vi "Straight.vi"() -> (4 "left":T2[](array[typedef])=[{"dt"=0.005, "x"=0.0, "y"=232.0, "position"=-3.125e-05, "velocity"=-0.0125, "acceleration"=-2.5, "jerk"=-500.0, "heading"=-0.0}, {"dt"=0.005, "x"=0.0, "y"=232.0, "position"=-3.125e-05, "velocity"=-0.0, "acceleration"=2.5, "jerk"=1000.0, "heading"=-0.0}, {"dt"=0.005, "x"=0.0, "y"=232.0, "position"=-3.125e-05, "velocity"=-0.0, "acceleration"=-0.0, "jerk"=-500.0, "heading"=-0.0}, {"dt"=0.005, "x"=0.0, "y"=232.0, "position"=-3.125e-05, "velocity"=-0.0, "acceleration"=-0.0, "jerk"=-0.0, "heading"=-0.0}, {"dt"=0.005, "x"=0.0, "y"=232.0, "position"=-3.125e-05, "velocity"=-0.0, "acceleration"=-0.0, "jerk"=-0.0, "heading"=-0.0}, {"dt"=0.005, "x"=0.0, "y"=232.0, "position"=-3.125e-05, "velocity"=-0.0, "acceleration"=-0.0, "jerk"=-0.0, "heading"=-0.0}, {"dt"=0.005, "x"=0.0, "y"=232.0, "position"=-3.125e-05, "velocity"=-0.0, "acceleration"=-0.0, "jerk"=-0.0, "heading"=-0.0}, {"dt"=0.005, "x"=0.0, "y"=232.0, "position"=-3.125e-05, "velocity"=-0.0, "acceleration"=-0.0, "jerk"=-0.0, "heading"=-0.0}, {"dt"=0.005, "x"=0.0, "y"=232.0, "position"=-3.125e-05, "velocity"=-0.0, "acceleration"=-0.0, "jerk"=-0.0, "heading"=-0.0}, {"dt"=0.005, "x"=3.124999999999981e-05, "y"=232.0, "position"=-6.249999999999981e-05, "velocity"=-0.006249999999999962, "acceleration"=-1.2499999999999925, "jerk"=-249.9999999999985, "heading"=-0.0}, {"dt"=0.005, "x"=0.003812499999999998, "y"=232.0, "position"=-0.0038437499999999978, "velocity"=-0.7562499999999996, "acceleration"=-149.99999999999994, "jerk"=-29749.99999999999, "heading"=-0.0}, {"dt"=0.005, "x"=0.008312499999999999, "y"=232.0, "position"=-0.008343749999999999, "velocity"=-0.9000000000000001, "acceleration"=-28.750000000000096, "jerk"=24249.999999999967, "heading"=-0.0}, {"dt"=0.005, "x"=0.013593749999999998, "y"=232.0, "position"=-0.013624999999999998, "velocity"=-1.05625, "acceleration"=-31.249999999999954, "jerk"=-499.9999999999716, "heading"=-0.0}, {"dt"=0.005, "x"=0.019718749999999997, "y"=232.0, "position"=-0.019749999999999997, "velocity"=-1.2249999999999996, "acceleration"=-33.74999999999994, "jerk"=-499.99999999999784, "heading"=-0.0}, {"dt"=0.005, "x"=0.026749999999999996, "y"=232.0, "position"=-0.026781249999999996, "velocity"=-1.4062499999999998, "acceleration"=-36.25000000000003, "jerk"=-500.00000000001705, "heading"=-0.0}, {"dt"=0.005, "x"=0.03474999999999999, "y"=232.0, "position"=-0.034781249999999986, "velocity"=-1.5999999999999985, "acceleration"=-38.74999999999975, "jerk"=-499.9999999999446, "heading"=-0.0}, {"dt"=0.005, "x"=0.04378125, "y"=232.0, "position"=-0.0438125, "velocity"=-1.8062500000000024, "acceleration"=-41.25000000000076, "jerk"=-500.0000000002018, "heading"=-0.0}, {"dt"=0.005, "x"=0.053906249999999996, "y"=232.0, "position"=-0.05393749999999999, "velocity"=-2.024999999999999, "acceleration"=-43.74999999999933, "jerk"=-499.99999999971436, "heading"=-0.0}, {"dt"=0.005, "x"=0.06518749999999998, "y"=232.0, "position"=-0.06521874999999998, "velocity"=-2.256249999999997, "acceleration"=-46.24999999999959, "jerk"=-500.00000000005116, "heading"=-0.0}, {"dt"=0.005, "x"=0.07768749999999996, "y"=232.0, "position"=-0.07771874999999996, "velocity"=-2.4999999999999964, "acceleration"=-48.74999999999989, "jerk"=-500.0000000000611, "heading"=-0.0}, {"dt"=0.005, "x"=0.09143749999999998, "y"=232.0, "position"=-0.09146874999999997, "velocity"=-2.750000000000002, "acceleration"=-50.00000000000115, "jerk"=-250.00000000025153, "heading"=-0.0}, {"dt"=0.005, "x"=0.10643749999999996, "y"=232.0, "position"=-0.10646874999999996, "velocity"=-2.999999999999997, "acceleration"=-49.999999999998934, "jerk"=4.433786671143025e-10, "heading"=-0.0}, {"dt"=0.005, "x"=0.12268749999999996, "y"=232.0, "position"=-0.12271874999999996, "velocity"=-3.25, "acceleration"=-50.00000000000062, "jerk"=-3.367972567502875e-10, "heading"=-0.0}, {"dt"=0.005, "x"=0.1401874999999999, "y"=232.0, "position"=-0.1402187499999999, "velocity"=-3.4999999999999893, "acceleration"=-49.99999999999787, "jerk"=5.499600774783175e-10, "heading"=-0.0}, {"dt"=0.005, "x"=0.1589374999999999, "y"=232.0, "position"=-0.15896874999999988, "velocity"=-3.749999999999998, "acceleration"=-50.000000000001684, "jerk"=-7.631228982063476e-10, "heading"=-0.0}, {"dt"=0.005, "x"=0.1789374999999999, "y"=232.0, "position"=-0.17896874999999987, "velocity"=-3.999999999999998, "acceleration"=-50.0, "jerk"=3.367972567502875e-10, "heading"=-0.0}, {"dt"=0.005, "x"=0.20018749999999985, "y"=232.0, "position"=-0.20021874999999983, "velocity"=-4.249999999999993, "acceleration"=-49.99999999999902, "jerk"=1.9610979506978765e-10, "heading"=-0.0}, {"dt"=0.005, "x"=0.22268749999999984, "y"=232.0, "position"=-0.22271874999999983, "velocity"=-4.499999999999998, "acceleration"=-50.000000000001066, "jerk"=-4.092726157978177e-10, "heading"=-0.0}, {"dt"=0.005, "x"=0.24643749999999992, "y"=232.0, "position"=-0.2464687499999999, "velocity"=-4.750000000000015, "acceleration"=-50.000000000003375, "jerk"=-4.618527782440651e-10, "heading"=-0.0}, {"dt"=0.005, "x"=0.2714375, "y"=232.0, "position"=-0.27146875, "velocity"=-5.000000000000015, "acceleration"=-50.0, "jerk"=6.750155989720952e-10, "heading"=-0.0}, {"dt"=0.005, "x"=0.2976875, "y"=232.0, "position"=-0.29771875, "velocity"=-5.249999999999999, "acceleration"=-49.9999999999968, "jerk"=6.394884621840902e-10, "heading"=-0.0}, {"dt"=0.005, "x"=0.3251875000000001, "y"=232.0, "position"=-0.32521875000000006, "velocity"=-5.500000000000016, "acceleration"=-50.000000000003375, "jerk"=-1.3145040611561853e-09, "heading"=-0.0}, {"dt"=0.005, "x"=0.3539375000000001, "y"=232.0, "position"=-0.3539687500000001, "velocity"=-5.750000000000011, "acceleration"=-49.999999999998934, "jerk"=8.881784197001252e-10, "heading"=-0.0}, {"dt"=0.005, "x"=0.38393750000000015, "y"=232.0, "position"=-0.38396875000000014, "velocity"=-6.000000000000005, "acceleration"=-49.999999999998934, "jerk"=-0.0, "heading"=-0.0}, {"dt"=0.005, "x"=0.4151875000000002, "y"=232.0, "position"=-0.4152187500000002, "velocity"=-6.250000000000011, "acceleration"=-50.000000000001066, "jerk"=-4.263256414560601e-10, "heading"=-0.0}, {"dt"=0.005, "x"=0.44768750000000024, "y"=232.0, "position"=-0.4477187500000002, "velocity"=-6.500000000000005, "acceleration"=-49.999999999998934, "jerk"=4.263256414560601e-10, "heading"=-0.0}, {"dt"=0.005, "x"=0.4814375000000002, "y"=232.0, "position"=-0.48146875000000017, "velocity"=-6.749999999999989, "acceleration"=-49.9999999999968, "jerk"=4.263256414560601e-10, "heading"=-0.0}, {"dt"=0.005, "x"=0.5164375000000001, "y"=232.0, "position"=-0.51646875, "velocity"=-6.999999999999984, "acceleration"=-49.999999999998934, "jerk"=-4.263256414560601e-10, "heading"=-0.0}, {"dt"=0.005, "x"=0.5526875, "y"=232.0, "position"=-0.5527187499999999, "velocity"=-7.249999999999979, "acceleration"=-49.999999999998934, "jerk"=-0.0, "heading"=-0.0}, {"dt"=0.005, "x"=0.5901874999999999, "y"=232.0, "position"=-0.5902187499999998, "velocity"=-7.499999999999973, "acceleration"=-49.999999999998934, "jerk"=-0.0, "heading"=-0.0}, {"dt"=0.005, "x"=0.6289374999999997, "y"=232.0, "position"=-0.6289687499999996, "velocity"=-7.749999999999968, "acceleration"=-49.999999999998934, "jerk"=-0.0, "heading"=-0.0}, {"dt"=0.005, "x"=0.6689374999999996, "y"=232.0, "position"=-0.6689687499999996, "velocity"=-7.999999999999985, "acceleration"=-50.000000000003375, "jerk"=-8.881784197001252e-10, "heading"=-0.0}, {"dt"=0.005, "x"=0.7101874999999995, "y"=232.0, "position"=-0.7102187499999995, "velocity"=-8.249999999999979, "acceleration"=-49.99999999999876, "jerk"=9.237055564881302e-10, "heading"=-0.0}, {"dt"=0.005, "x"=0.7526874999999994, "y"=232.0, "position"=-0.7527187499999993, "velocity"=-8.499999999999973, "acceleration"=-49.999999999998934, "jerk"=-3.552713678800501e-11, "heading"=-0.0}, {"dt"=0.005, "x"=0.7964374999999992, "y"=232.0, "position"=-0.7964687499999992, "velocity"=-8.749999999999968, "acceleration"=-49.999999999998934, "jerk"=-0.0, "heading"=-0.0}, {"dt"=0.005, "x"=0.8414374999999993, "y"=232.0, "position"=-0.8414687499999992, "velocity"=-9.000000000000007, "acceleration"=-50.000000000007816, "jerk"=-1.7763568394002505e-09, "heading"=-0.0}, {"dt"=0.005, "x"=0.8876874999999992, "y"=232.0, "position"=-0.8877187499999991, "velocity"=-9.24999999999998, "acceleration"=-49.99999999999467, "jerk"=2.6290081223123707e-09, "heading"=-0.0}, {"dt"=0.005, "x"=0.9351874999999988, "y"=232.0, "position"=-0.9352187499999988, "velocity"=-9.49999999999993, "acceleration"=-49.99999999999005, "jerk"=9.237055564881302e-10, "heading"=-0.0}, {"dt"=0.005, "x"=0.9839374999999992, "y"=232.0, "position"=-0.9839687499999992, "velocity"=-9.75000000000008, "acceleration"=-50.00000000002984, "jerk"=-7.958078640513122e-09, "heading"=-0.0}, {"dt"=0.005, "x"=1.0339374999999993, "y"=232.0, "position"=-1.0339687499999992, "velocity"=-10.000000000000009, "acceleration"=-49.99999999998579, "jerk"=8.810729923425242e-09, "heading"=-0.0}, {"dt"=0.005, "x"=1.0851874999999997, "y"=232.0, "position"=-1.0852187499999997, "velocity"=-10.250000000000092, "acceleration"=-50.0000000000167, "jerk"=-6.181721801112872e-09, "heading"=-0.0}, {"dt"=0.005, "x"=1.1376875, "y"=232.0, "position"=-1.13771875, "velocity"=-10.500000000000043, "acceleration"=-49.99999999999005, "jerk"=5.329070518200751e-09, "heading"=-0.0}, {"dt"=0.005, "x"=1.1914375000000004, "y"=232.0, "position"=-1.1914687500000003, "velocity"=-10.750000000000082, "acceleration"=-50.000000000007816, "jerk"=-3.552713678800501e-09, "heading"=-0.0}, {"dt"=0.005, "x"=1.2464375000000005, "y"=232.0, "position"=-1.2464687500000005, "velocity"=-11.000000000000032, "acceleration"=-49.99999999999005, "jerk"=3.552713678800501e-09, "heading"=-0.0}, {"dt"=0.005, "x"=1.3026875000000009, "y"=232.0, "position"=-1.3027187500000008, "velocity"=-11.250000000000071, "acceleration"=-50.000000000007816, "jerk"=-3.552713678800501e-09, "heading"=-0.0}, {"dt"=0.005, "x"=1.3601875000000012, "y"=232.0, "position"=-1.3602187500000011, "velocity"=-11.500000000000066, "acceleration"=-49.999999999998934, "jerk"=1.7763568394002505e-09, "heading"=-0.0}, {"dt"=0.005, "x"=1.418937500000002, "y"=232.0, "position"=-1.4189687500000019, "velocity"=-11.75000000000015, "acceleration"=-50.0000000000167, "jerk"=-3.552713678800501e-09, "heading"=-0.0}, {"dt"=0.005, "x"=1.4789375000000022, "y"=232.0, "position"=-1.4789687500000022, "velocity"=-12.000000000000055, "acceleration"=-49.99999999998117, "jerk"=7.105427357601002e-09, "heading"=-0.0}, {"dt"=0.005, "x"=1.5401875000000025, "y"=232.0, "position"=-1.5402187500000024, "velocity"=-12.25000000000005, "acceleration"=-49.999999999998934, "jerk"=-3.552713678800501e-09, "heading"=-0.0}, {"dt"=0.005, "x"=1.602687500000003, "y"=232.0, "position"=-1.6027187500000029, "velocity"=-12.500000000000089, "acceleration"=-50.000000000007816, "jerk"=-1.7763568394002505e-09, "heading"=-0.0}, {"dt"=0.005, "x"=1.6664375000000031, "y"=232.0, "position"=-1.666468750000003, "velocity"=-12.750000000000039, "acceleration"=-49.99999999999005, "jerk"=3.552713678800501e-09, "heading"=-0.0}, {"dt"=0.005, "x"=1.7314375000000037, "y"=232.0, "position"=-1.7314687500000037, "velocity"=-13.000000000000123, "acceleration"=-50.0000000000167, "jerk"=-5.329070518200751e-09, "heading"=-0.0}, {"dt"=0.005, "x"=1.7976875000000039, "y"=232.0, "position"=-1.7977187500000038, "velocity"=-13.250000000000028, "acceleration"=-49.99999999998117, "jerk"=7.105427357601002e-09, "heading"=-0.0}, {"dt"=0.005, "x"=1.8651875000000044, "y"=232.0, "position"=-1.8652187500000044, "velocity"=-13.500000000000112, "acceleration"=-50.0000000000167, "jerk"=-7.105427357601002e-09, "heading"=-0.0}, {"dt"=0.005, "x"=1.9339375000000047, "y"=232.0, "position"=-1.9339687500000047, "velocity"=-13.750000000000062, "acceleration"=-49.99999999999005, "jerk"=5.329070518200751e-09, "heading"=-0.0}, {"dt"=0.005, "x"=2.0039375000000055, "y"=232.0, "position"=-2.0039687500000056, "velocity"=-14.000000000000146, "acceleration"=-50.0000000000167, "jerk"=-5.329070518200751e-09, "heading"=-0.0}, {"dt"=0.005, "x"=2.075187500000006, "y"=232.0, "position"=-2.075218750000006, "velocity"=-14.250000000000096, "acceleration"=-49.99999999999005, "jerk"=5.329070518200751e-09, "heading"=-0.0}, {"dt"=0.005, "x"=2.1476875000000057, "y"=232.0, "position"=-2.147718750000006, "velocity"=-14.499999999999957, "acceleration"=-49.99999999997229, "jerk"=3.552713678800501e-09, "heading"=-0.0}, {"dt"=0.005, "x"=2.2214375000000066, "y"=232.0, "position"=-2.2214687500000068, "velocity"=-14.750000000000174, "acceleration"=-50.00000000004334, "jerk"=-1.4210854715202004e-08, "heading"=-0.0}, {"dt"=0.005, "x"=2.296437500000007, "y"=232.0, "position"=-2.296468750000007, "velocity"=-15.000000000000036, "acceleration"=-49.99999999997229, "jerk"=1.4210854715202004e-08, "heading"=-0.0}, {"dt"=0.005, "x"=2.3726875000000076, "y"=232.0, "position"=-2.3727187500000078, "velocity"=-15.250000000000163, "acceleration"=-50.00000000002558, "jerk"=-1.0658141036401503e-08, "heading"=-0.0}, {"dt"=0.005, "x"=2.450187500000008, "y"=232.0, "position"=-2.4502187500000083, "velocity"=-15.500000000000114, "acceleration"=-49.99999999999005, "jerk"=7.105427357601002e-09, "heading"=-0.0}, {"dt"=0.005, "x"=2.5289375000000085, "y"=232.0, "position"=-2.5289687500000086, "velocity"=-15.750000000000064, "acceleration"=-49.99999999999005, "jerk"=-0.0, "heading"=-0.0}, {"dt"=0.005, "x"=2.608937500000009, "y"=232.0, "position"=-2.608968750000009, "velocity"=-16.000000000000103, "acceleration"=-50.000000000007816, "jerk"=-3.552713678800501e-09, "heading"=-0.0}, {"dt"=0.005, "x"=2.6901875000000093, "y"=232.0, "position"=-2.6902187500000094, "velocity"=-16.250000000000053, "acceleration"=-49.99999999999005, "jerk"=3.552713678800501e-09, "heading"=-0.0}, {"dt"=0.005, "x"=2.7726875000000097, "y"=232.0, "position"=-2.77271875000001, "velocity"=-16.500000000000092, "acceleration"=-50.000000000007816, "jerk"=-3.552713678800501e-09, "heading"=-0.0}, {"dt"=0.005, "x"=2.8564375000000104, "y"=232.0, "position"=-2.8564687500000105, "velocity"=-16.75000000000013, "acceleration"=-50.000000000007816, "jerk"=-0.0, "heading"=-0.0}, {"dt"=0.005, "x"=2.9414375000000113, "y"=232.0, "position"=-2.9414687500000114, "velocity"=-17.00000000000017, "acceleration"=-50.000000000007816, "jerk"=-0.0, "heading"=-0.0}, {"dt"=0.005, "x"=3.027687500000012, "y"=232.0, "position"=-3.027718750000012, "velocity"=-17.25000000000012, "acceleration"=-49.99999999999005, "jerk"=3.552713678800501e-09, "heading"=-0.0}, {"dt"=0.005, "x"=3.115187500000012, "y"=232.0, "position"=-3.1152187500000124, "velocity"=-17.50000000000007, "acceleration"=-49.99999999999005, "jerk"=-0.0, "heading"=-0.0}, {"dt"=0.005, "x"=3.2039375000000128, "y"=232.0, "position"=-3.203968750000013, "velocity"=-17.75000000000011, "acceleration"=-50.000000000007816, "jerk"=-3.552713678800501e-09, "heading"=-0.0}, {"dt"=0.005, "x"=3.293937500000013, "y"=232.0, "position"=-3.293968750000013, "velocity"=-18.00000000000006, "acceleration"=-49.99999999999005, "jerk"=3.552713678800501e-09, "heading"=-0.0}, {"dt"=0.005, "x"=3.3851875000000136, "y"=232.0, "position"=-3.3852187500000137, "velocity"=-18.2500000000001, "acceleration"=-50.000000000007816, "jerk"=-3.552713678800501e-09, "heading"=-0.0}, {"dt"=0.005, "x"=3.4776875000000143, "y"=232.0, "position"=-3.4777187500000144, "velocity"=-18.50000000000014, "acceleration"=-50.000000000007816, "jerk"=-0.0, "heading"=-0.0}, {"dt"=0.005, "x"=3.5714375000000147, "y"=232.0, "position"=-3.571468750000015, "velocity"=-18.75000000000009, "acceleration"=-49.99999999999005, "jerk"=3.552713678800501e-09, "heading"=-0.0}, {"dt"=0.005, "x"=3.6664375000000153, "y"=232.0, "position"=-3.6664687500000155, "velocity"=-19.000000000000128, "acceleration"=-50.000000000007816, "jerk"=-3.552713678800501e-09, "heading"=-0.0}, {"dt"=0.005, "x"=3.762687500000014, "y"=232.0, "position"=-3.762718750000014, "velocity"=-19.249999999999723, "acceleration"=-49.999999999919, "jerk"=1.7763568394002505e-08, "heading"=-0.0}, {"dt"=0.005, "x"=3.8601875000000123, "y"=232.0, "position"=-3.8602187500000125, "velocity"=-19.499999999999673, "acceleration"=-49.99999999999005, "jerk"=-1.4210854715202004e-08, "heading"=-0.0}, {"dt"=0.005, "x"=3.958937500000009, "y"=232.0, "position"=-3.9589687500000093, "velocity"=-19.749999999999357, "acceleration"=-49.99999999993676, "jerk"=1.0658141036401503e-08, "heading"=-0.0}, {"dt"=0.005, "x"=4.058937500000005, "y"=232.0, "position"=-4.058968750000005, "velocity"=-19.99999999999922, "acceleration"=-49.99999999997229, "jerk"=-7.105427357601002e-09, "heading"=-0.0}, {"dt"=0.005, "x"=4.160187500000004, "y"=232.0, "position"=-4.160218750000004, "velocity"=-20.2499999999997, "acceleration"=-50.000000000096634, "jerk"=-2.4868995751603507e-08, "heading"=-0.0}, {"dt"=0.005, "x"=4.2626875, "y"=232.0, "position"=-4.26271875, "velocity"=-20.499999999999297, "acceleration"=-49.999999999919, "jerk"=3.552713678800501e-08, "heading"=-0.0}, {"dt"=0.005, "x"=4.366437499999997, "y"=232.0, "position"=-4.3664687499999975, "velocity"=-20.749999999999424, "acceleration"=-50.00000000002558, "jerk"=-2.1316282072803006e-08, "heading"=-0.0}, {"dt"=0.005, "x"=4.471437499999994, "y"=232.0, "position"=-4.471468749999994, "velocity"=-20.999999999999375, "acceleration"=-49.99999999999005, "jerk"=7.105427357601002e-09, "heading"=-0.0}, {"dt"=0.005, "x"=4.577687499999992, "y"=232.0, "position"=-4.577718749999992, "velocity"=-21.249999999999503, "acceleration"=-50.00000000002558, "jerk"=-7.105427357601002e-09, "heading"=-0.0}, {"dt"=0.005, "x"=4.685187499999989, "y"=232.0, "position"=-4.685218749999989, "velocity"=-21.499999999999453, "acceleration"=-49.99999999999005, "jerk"=7.105427357601002e-09, "heading"=-0.0}, {"dt"=0.005, "x"=4.793937499999985, "y"=232.0, "position"=-4.793968749999985, "velocity"=-21.749999999999226, "acceleration"=-49.999999999954525, "jerk"=7.105427357601002e-09, "heading"=-0.0}, {"dt"=0.005, "x"=4.903937499999983, "y"=232.0, "position"=-4.903968749999983, "velocity"=-21.99999999999953, "acceleration"=-50.00000000006111, "jerk"=-2.1316282072803006e-08, "heading"=-0.0}, {"dt"=0.005, "x"=5.015187499999979, "y"=232.0, "position"=-5.015218749999979, "velocity"=-22.249999999999304, "acceleration"=-49.999999999954525, "jerk"=2.1316282072803006e-08, "heading"=-0.0}, {"dt"=0.005, "x"=5.1276874999999755, "y"=232.0, "position"=-5.127718749999976, "velocity"=-22.499999999999254, "acceleration"=-49.99999999999005, "jerk"=-7.105427357601002e-09, "heading"=-0.0}, {"dt"=0.005, "x"=5.241437499999972, "y"=232.0, "position"=-5.241468749999973, "velocity"=-22.749999999999382, "acceleration"=-50.00000000002558, "jerk"=-7.105427357601002e-09, "heading"=-0.0}, {"dt"=0.005, "x"=5.356437499999968, "y"=232.0, "position"=-5.356468749999968, "velocity"=-22.999999999999154, "acceleration"=-49.999999999954525, "jerk"=1.4210854715202004e-08, "heading"=-0.0}, {"dt"=0.005, "x"=5.4726874999999655, "y"=232.0, "position"=-5.472718749999966, "velocity"=-23.24999999999946, "acceleration"=-50.00000000006111, "jerk"=-2.1316282072803006e-08, "heading"=-0.0}, {"dt"=0.005, "x"=5.590187499999963, "y"=232.0, "position"=-5.590218749999963, "velocity"=-23.49999999999941, "acceleration"=-49.99999999999005, "jerk"=1.4210854715202004e-08, "heading"=-0.0}, {"dt"=0.005, "x"=5.708937499999959, "y"=232.0, "position"=-5.7089687499999595, "velocity"=-23.74999999999936, "acceleration"=-49.99999999999005, "jerk"=-0.0, "heading"=-0.0}, {"dt"=0.005, "x"=5.828937499999956, "y"=232.0, "position"=-5.828968749999956, "velocity"=-23.99999999999931, "acceleration"=-49.99999999999005, "jerk"=-0.0, "heading"=-0.0}, {"dt"=0.005, "x"=5.950187499999952, "y"=232.0, "position"=-5.950218749999952, "velocity"=-24.24999999999926, "acceleration"=-49.99999999999005, "jerk"=-0.0, "heading"=-0.0}, {"dt"=0.005, "x"=6.072687499999948, "y"=232.0, "position"=-6.072718749999948, "velocity"=-24.49999999999921, "acceleration"=-49.99999999999005, "jerk"=-0.0, "heading"=-0.0}, {"dt"=0.005, "x"=6.196437499999945, "y"=232.0, "position"=-6.196468749999945, "velocity"=-24.74999999999934, "acceleration"=-50.00000000002558, "jerk"=-7.105427357601002e-09, "heading"=-0.0}, {"dt"=0.005, "x"=6.321437499999941, "y"=232.0, "position"=-6.321468749999942, "velocity"=-24.99999999999929, "acceleration"=-49.99999999999005, "jerk"=7.105427357601002e-09, "heading"=-0.0}, {"dt"=0.005, "x"=6.447687499999938, "y"=232.0, "position"=-6.447718749999938, "velocity"=-25.24999999999924, "acceleration"=-49.99999999999005, "jerk"=-0.0, "heading"=-0.0}, {"dt"=0.005, "x"=6.5751874999999345, "y"=232.0, "position"=-6.575218749999935, "velocity"=-25.499999999999368, "acceleration"=-50.00000000002558, "jerk"=-7.105427357601002e-09, "heading"=-0.0}, {"dt"=0.005, "x"=6.703937499999931, "y"=232.0, "position"=-6.703968749999931, "velocity"=-25.749999999999318, "acceleration"=-49.99999999999005, "jerk"=7.105427357601002e-09, "heading"=-0.0}, {"dt"=0.005, "x"=6.833937499999927, "y"=232.0, "position"=-6.8339687499999275, "velocity"=-25.999999999999268, "acceleration"=-49.99999999999005, "jerk"=-0.0, "heading"=-0.0}, {"dt"=0.005, "x"=6.965187499999923, "y"=232.0, "position"=-6.965218749999923, "velocity"=-26.24999999999904, "acceleration"=-49.999999999954525, "jerk"=7.105427357601002e-09, "heading"=-0.0}, {"dt"=0.005, "x"=7.09768749999992, "y"=232.0, "position"=-7.09771874999992, "velocity"=-26.499999999999524, "acceleration"=-50.000000000096634, "jerk"=-2.8421709430404007e-08, "heading"=-0.0}, {"dt"=0.005, "x"=7.231437499999915, "y"=232.0, "position"=-7.231468749999915, "velocity"=-26.74999999999894, "acceleration"=-49.99999999988347, "jerk"=4.263256414560601e-08, "heading"=-0.0}, {"dt"=0.005, "x"=7.366437499999912, "y"=232.0, "position"=-7.366468749999912, "velocity"=-26.999999999999424, "acceleration"=-50.000000000096634, "jerk"=-4.263256414560601e-08, "heading"=-0.0}, {"dt"=0.005, "x"=7.502687499999908, "y"=232.0, "position"=-7.502718749999908, "velocity"=-27.249999999999197, "acceleration"=-49.999999999954525, "jerk"=2.8421709430404007e-08, "heading"=-0.0}, {"dt"=0.005, "x"=7.640187499999904, "y"=232.0, "position"=-7.640218749999904, "velocity"=-27.499999999999147, "acceleration"=-49.99999999999005, "jerk"=-7.105427357601002e-09, "heading"=-0.0}, {"dt"=0.005, "x"=7.7789374999999, "y"=232.0, "position"=-7.7789687499999, "velocity"=-27.749999999999275, "acceleration"=-50.00000000002558, "jerk"=-7.105427357601002e-09, "heading"=-0.0}, {"dt"=0.005, "x"=7.918937499999897, "y"=232.0, "position"=-7.918968749999897, "velocity"=-27.999999999999403, "acceleration"=-50.00000000002558, "jerk"=-0.0, "heading"=-0.0}, {"dt"=0.005, "x"=8.060187499999891, "y"=232.0, "position"=-8.06021874999989, "velocity"=-28.24999999999882, "acceleration"=-49.99999999988347, "jerk"=2.8421709430404007e-08, "heading"=-0.0}, {"dt"=0.005, "x"=8.20268749999989, "y"=232.0, "position"=-8.202718749999889, "velocity"=-28.49999999999966, "acceleration"=-50.00000000016769, "jerk"=-5.6843418860808015e-08, "heading"=-0.0}, {"dt"=0.005, "x"=8.346437499999885, "y"=232.0, "position"=-8.346468749999884, "velocity"=-28.749999999999076, "acceleration"=-49.99999999988347, "jerk"=5.6843418860808015e-08, "heading"=-0.0}, {"dt"=0.005, "x"=8.491437499999881, "y"=232.0, "position"=-8.49146874999988, "velocity"=-28.999999999999204, "acceleration"=-50.00000000002558, "jerk"=-2.8421709430404007e-08, "heading"=-0.0}, {"dt"=0.005, "x"=8.637687499999876, "y"=232.0, "position"=-8.637718749999875, "velocity"=-29.249999999998977, "acceleration"=-49.999999999954525, "jerk"=1.4210854715202004e-08, "heading"=-0.0}, {"dt"=0.005, "x"=8.785187499999873, "y"=232.0, "position"=-8.785218749999872, "velocity"=-29.49999999999946, "acceleration"=-50.000000000096634, "jerk"=-2.8421709430404007e-08, "heading"=-0.0}, {"dt"=0.005, "x"=8.933937499999868, "y"=232.0, "position"=-8.933968749999867, "velocity"=-29.749999999998877, "acceleration"=-49.99999999988347, "jerk"=4.263256414560601e-08, "heading"=-0.0}, {"dt"=0.005, "x"=9.083937499999864, "y"=232.0, "position"=-9.083968749999864, "velocity"=-29.99999999999936, "acceleration"=-50.000000000096634, "jerk"=-4.263256414560601e-08, "heading"=-0.0}, {"dt"=0.005, "x"=9.235187499999858, "y"=232.0, "position"=-9.235218749999857, "velocity"=-30.249999999998778, "acceleration"=-49.99999999988347, "jerk"=4.263256414560601e-08, "heading"=-0.0}, {"dt"=0.005, "x"=9.387687499999853, "y"=232.0, "position"=-9.387718749999852, "velocity"=-30.499999999998906, "acceleration"=-50.00000000002558, "jerk"=-2.8421709430404007e-08, "heading"=-0.0}, {"dt"=0.005, "x"=9.541437499999851, "y"=232.0, "position"=-9.54146874999985, "velocity"=-30.749999999999744, "acceleration"=-50.00000000016769, "jerk"=-2.8421709430404007e-08, "heading"=-0.0}, {"dt"=0.005, "x"=9.696437499999845, "y"=232.0, "position"=-9.696468749999845, "velocity"=-30.999999999998806, "acceleration"=-49.99999999981242, "jerk"=7.105427357601002e-08, "heading"=-0.0}, {"dt"=0.005, "x"=9.85268749999984, "y"=232.0, "position"=-9.85271874999984, "velocity"=-31.249999999998934, "acceleration"=-50.00000000002558, "jerk"=-4.263256414560601e-08, "heading"=-0.0}, {"dt"=0.005, "x"=10.010187499999837, "y"=232.0, "position"=-10.010218749999837, "velocity"=-31.499999999999417, "acceleration"=-50.000000000096634, "jerk"=-1.4210854715202004e-08, "heading"=-0.0}, {"dt"=0.005, "x"=10.168937499999831, "y"=232.0, "position"=-10.16896874999983, "velocity"=-31.749999999998835, "acceleration"=-49.99999999988347, "jerk"=4.263256414560601e-08, "heading"=-0.0}, {"dt"=0.005, "x"=10.328937499999828, "y"=232.0, "position"=-10.328968749999827, "velocity"=-31.999999999999318, "acceleration"=-50.000000000096634, "jerk"=-4.263256414560601e-08, "heading"=-0.0}, {"dt"=0.005, "x"=10.490187499999823, "y"=232.0, "position"=-10.490218749999823, "velocity"=-32.24999999999909, "acceleration"=-49.999999999954525, "jerk"=2.8421709430404007e-08, "heading"=-0.0}, {"dt"=0.005, "x"=10.65268749999982, "y"=232.0, "position"=-10.652718749999819, "velocity"=-32.49999999999922, "acceleration"=-50.00000000002558, "jerk"=-1.4210854715202004e-08, "heading"=-0.0}, {"dt"=0.005, "x"=10.816437499999815, "y"=232.0, "position"=-10.816468749999814, "velocity"=-32.74999999999899, "acceleration"=-49.999999999954525, "jerk"=1.4210854715202004e-08, "heading"=-0.0}, {"dt"=0.005, "x"=10.98143749999981, "y"=232.0, "position"=-10.98146874999981, "velocity"=-32.99999999999912, "acceleration"=-50.00000000002558, "jerk"=-1.4210854715202004e-08, "heading"=-0.0}, {"dt"=0.005, "x"=11.147687499999805, "y"=232.0, "position"=-11.147718749999804, "velocity"=-33.24999999999889, "acceleration"=-49.999999999954525, "jerk"=1.4210854715202004e-08, "heading"=-0.0}, {"dt"=0.005, "x"=11.3151874999998, "y"=232.0, "position"=-11.315218749999799, "velocity"=-33.49999999999902, "acceleration"=-50.00000000002558, "jerk"=-1.4210854715202004e-08, "heading"=-0.0}, {"dt"=0.005, "x"=11.483937499999794, "y"=232.0, "position"=-11.483968749999793, "velocity"=-33.74999999999879, "acceleration"=-49.999999999954525, "jerk"=1.4210854715202004e-08, "heading"=-0.0}, {"dt"=0.005, "x"=11.653937499999788, "y"=232.0, "position"=-11.653968749999787, "velocity"=-33.99999999999892, "acceleration"=-50.00000000002558, "jerk"=-1.4210854715202004e-08, "heading"=-0.0}, {"dt"=0.005, "x"=11.825187499999783, "y"=232.0, "position"=-11.825218749999783, "velocity"=-34.24999999999905, "acceleration"=-50.00000000002558, "jerk"=-0.0, "heading"=-0.0}, {"dt"=0.005, "x"=11.997687499999781, "y"=232.0, "position"=-11.99771874999978, "velocity"=-34.49999999999953, "acceleration"=-50.000000000096634, "jerk"=-1.4210854715202004e-08, "heading"=-0.0}, {"dt"=0.005, "x"=12.171437499999774, "y"=232.0, "position"=-12.171468749999773, "velocity"=-34.74999999999859, "acceleration"=-49.99999999981242, "jerk"=5.6843418860808015e-08, "heading"=-0.0}, {"dt"=0.005, "x"=12.346437499999771, "y"=232.0, "position"=-12.34646874999977, "velocity"=-34.99999999999943, "acceleration"=-50.00000000016769, "jerk"=-7.105427357601002e-08, "heading"=-0.0}, {"dt"=0.005, "x"=12.522687499999764, "y"=232.0, "position"=-12.522718749999763, "velocity"=-35.249999999998494, "acceleration"=-49.99999999981242, "jerk"=7.105427357601002e-08, "heading"=-0.0}, {"dt"=0.005, "x"=12.700187499999759, "y"=232.0, "position"=-12.700218749999758, "velocity"=-35.49999999999898, "acceleration"=-50.000000000096634, "jerk"=-5.6843418860808015e-08, "heading"=-0.0}, {"dt"=0.005, "x"=12.878937499999756, "y"=232.0, "position"=-12.878968749999755, "velocity"=-35.74999999999946, "acceleration"=-50.000000000096634, "jerk"=-0.0, "heading"=-0.0}, {"dt"=0.005, "x"=13.058937499999749, "y"=232.0, "position"=-13.058968749999748, "velocity"=-35.99999999999852, "acceleration"=-49.99999999981242, "jerk"=5.6843418860808015e-08, "heading"=-0.0}, {"dt"=0.005, "x"=13.240187499999745, "y"=232.0, "position"=-13.240218749999745, "velocity"=-36.24999999999936, "acceleration"=-50.00000000016769, "jerk"=-7.105427357601002e-08, "heading"=-0.0}, {"dt"=0.005, "x"=13.42268749999974, "y"=232.0, "position"=-13.422718749999738, "velocity"=-36.49999999999878, "acceleration"=-49.99999999988347, "jerk"=5.6843418860808015e-08, "heading"=-0.0}, {"dt"=0.005, "x"=13.606437499999734, "y"=232.0, "position"=-13.606468749999733, "velocity"=-36.749999999998906, "acceleration"=-50.00000000002558, "jerk"=-2.8421709430404007e-08, "heading"=-0.0}, {"dt"=0.005, "x"=13.791437499999729, "y"=232.0, "position"=-13.791468749999728, "velocity"=-36.999999999999034, "acceleration"=-50.00000000002558, "jerk"=-0.0, "heading"=-0.0}, {"dt"=0.005, "x"=13.977687499999725, "y"=232.0, "position"=-13.977718749999724, "velocity"=-37.24999999999916, "acceleration"=-50.00000000002558, "jerk"=-0.0, "heading"=-0.0}, {"dt"=0.005, "x"=14.165187499999718, "y"=232.0, "position"=-14.165218749999717, "velocity"=-37.49999999999858, "acceleration"=-49.99999999988347, "jerk"=2.8421709430404007e-08, "heading"=-0.0}, {"dt"=0.005, "x"=14.353937499999713, "y"=232.0, "position"=-14.353968749999712, "velocity"=-37.74999999999906, "acceleration"=-50.000000000096634, "jerk"=-4.263256414560601e-08, "heading"=-0.0}, {"dt"=0.005, "x"=14.543937499999707, "y"=232.0, "position"=-14.543968749999706, "velocity"=-37.999999999998835, "acceleration"=-49.999999999954525, "jerk"=2.8421709430404007e-08, "heading"=-0.0}, {"dt"=0.005, "x"=14.735187499999702, "y"=232.0, "position"=-14.735218749999701, "velocity"=-38.24999999999896, "acceleration"=-50.00000000002558, "jerk"=-1.4210854715202004e-08, "heading"=-0.0}, {"dt"=0.005, "x"=14.927687499999696, "y"=232.0, "position"=-14.927718749999695, "velocity"=-38.499999999998735, "acceleration"=-49.999999999954525, "jerk"=1.4210854715202004e-08, "heading"=-0.0}, {"dt"=0.005, "x"=15.121437499999708, "y"=232.0, "position"=-15.121468749999707, "velocity"=-38.750000000002416, "acceleration"=-50.00000000073612, "jerk"=-1.5631940186722204e-07, "heading"=-0.0}, {"dt"=0.005, "x"=15.316437499999733, "y"=232.0, "position"=-15.316468749999732, "velocity"=-39.00000000000503, "acceleration"=-50.00000000052296, "jerk"=4.263256414560601e-08, "heading"=-0.0}, {"dt"=0.005, "x"=15.512687499999753, "y"=232.0, "position"=-15.512718749999753, "velocity"=-39.25000000000409, "acceleration"=-49.99999999981242, "jerk"=1.4210854715202004e-07, "heading"=-0.0}, {"dt"=0.005, "x"=15.710187499999774, "y"=232.0, "position"=-15.710218749999774, "velocity"=-39.50000000000422, "acceleration"=-50.00000000002558, "jerk"=-4.263256414560601e-08, "heading"=-0.0}, {"dt"=0.005, "x"=15.908937499999794, "y"=232.0, "position"=-15.908968749999794, "velocity"=-39.75000000000399, "acceleration"=-49.999999999954525, "jerk"=1.4210854715202004e-08, "heading"=-0.0}, {"dt"=0.005, "x"=16.10893749999982, "y"=232.0, "position"=-16.108968749999818, "velocity"=-40.00000000000483, "acceleration"=-50.00000000016769, "jerk"=-4.263256414560601e-08, "heading"=-0.0}, {"dt"=0.005, "x"=16.31018749999984, "y"=232.0, "position"=-16.31021874999984, "velocity"=-40.250000000004604, "acceleration"=-49.999999999954525, "jerk"=4.263256414560601e-08, "heading"=-0.0}, {"dt"=0.005, "x"=16.512687499999863, "y"=232.0, "position"=-16.512718749999863, "velocity"=-40.50000000000438, "acceleration"=-49.999999999954525, "jerk"=-0.0, "heading"=-0.0}, {"dt"=0.005, "x"=16.716437499999884, "y"=232.0, "position"=-16.716468749999883, "velocity"=-40.75000000000415, "acceleration"=-49.999999999954525, "jerk"=-0.0, "heading"=-0.0}, {"dt"=0.005, "x"=16.92143749999991, "y"=232.0, "position"=-16.92146874999991, "velocity"=-41.00000000000534, "acceleration"=-50.00000000023874, "jerk"=-5.6843418860808015e-08, "heading"=-0.0}, {"dt"=0.005, "x"=17.127687499999933, "y"=232.0, "position"=-17.127718749999932, "velocity"=-41.250000000004405, "acceleration"=-49.99999999981242, "jerk"=8.526512829121202e-08, "heading"=-0.0}, {"dt"=0.005, "x"=17.335187499999954, "y"=232.0, "position"=-17.335218749999953, "velocity"=-41.50000000000418, "acceleration"=-49.999999999954525, "jerk"=-2.8421709430404007e-08, "heading"=-0.0}, {"dt"=0.005, "x"=17.543937499999974, "y"=232.0, "position"=-17.543968749999973, "velocity"=-41.75000000000395, "acceleration"=-49.999999999954525, "jerk"=-0.0, "heading"=-0.0}, {"dt"=0.005, "x"=17.7539375, "y"=232.0, "position"=-17.75396875, "velocity"=-42.000000000005144, "acceleration"=-50.00000000023874, "jerk"=-5.6843418860808015e-08, "heading"=-0.0}, {"dt"=0.005, "x"=17.96518750000002, "y"=232.0, "position"=-17.96521875000002, "velocity"=-42.250000000004206, "acceleration"=-49.99999999981242, "jerk"=8.526512829121202e-08, "heading"=-0.0}, {"dt"=0.005, "x"=18.177687500000044, "y"=232.0, "position"=-18.177718750000043, "velocity"=-42.50000000000469, "acceleration"=-50.000000000096634, "jerk"=-5.6843418860808015e-08, "heading"=-0.0}, {"dt"=0.005, "x"=18.391437500000066, "y"=232.0, "position"=-18.391468750000065, "velocity"=-42.75000000000446, "acceleration"=-49.999999999954525, "jerk"=2.8421709430404007e-08, "heading"=-0.0}, {"dt"=0.005, "x"=18.60643750000009, "y"=232.0, "position"=-18.60646875000009, "velocity"=-43.000000000004945, "acceleration"=-50.000000000096634, "jerk"=-2.8421709430404007e-08, "heading"=-0.0}, {"dt"=0.005, "x"=18.822687500000114, "y"=232.0, "position"=-18.822718750000114, "velocity"=-43.25000000000472, "acceleration"=-49.999999999954525, "jerk"=2.8421709430404007e-08, "heading"=-0.0}, {"dt"=0.005, "x"=19.04018750000014, "y"=232.0, "position"=-19.04021875000014, "velocity"=-43.5000000000052, "acceleration"=-50.000000000096634, "jerk"=-2.8421709430404007e-08, "heading"=-0.0}, {"dt"=0.005, "x"=19.25893750000016, "y"=232.0, "position"=-19.25896875000016, "velocity"=-43.75000000000426, "acceleration"=-49.99999999981242, "jerk"=5.6843418860808015e-08, "heading"=-0.0}, {"dt"=0.005, "x"=19.478937500000185, "y"=232.0, "position"=-19.478968750000185, "velocity"=-44.000000000004746, "acceleration"=-50.000000000096634, "jerk"=-5.6843418860808015e-08, "heading"=-0.0}, {"dt"=0.005, "x"=19.700187500000215, "y"=232.0, "position"=-19.700218750000214, "velocity"=-44.25000000000594, "acceleration"=-50.00000000023874, "jerk"=-2.8421709430404007e-08, "heading"=-0.0}, {"dt"=0.005, "x"=19.922687500000237, "y"=232.0, "position"=-19.922718750000236, "velocity"=-44.50000000000429, "acceleration"=-49.99999999967031, "jerk"=1.1368683772161603e-07, "heading"=-0.0}, {"dt"=0.005, "x"=20.14643750000026, "y"=232.0, "position"=-20.14646875000026, "velocity"=-44.750000000004775, "acceleration"=-50.000000000096634, "jerk"=-8.526512829121202e-08, "heading"=-0.0}, {"dt"=0.005, "x"=20.371437500000287, "y"=232.0, "position"=-20.371468750000286, "velocity"=-45.00000000000526, "acceleration"=-50.000000000096634, "jerk"=-0.0, "heading"=-0.0}, {"dt"=0.005, "x"=20.597687500000312, "y"=232.0, "position"=-20.59771875000031, "velocity"=-45.25000000000503, "acceleration"=-49.999999999954525, "jerk"=2.8421709430404007e-08, "heading"=-0.0}, {"dt"=0.005, "x"=20.825187500000336, "y"=232.0, "position"=-20.825218750000335, "velocity"=-45.5000000000048, "acceleration"=-49.999999999954525, "jerk"=-0.0, "heading"=-0.0}, {"dt"=0.005, "x"=21.05393750000036, "y"=232.0, "position"=-21.053968750000358, "velocity"=-45.750000000004576, "acceleration"=-49.999999999954525, "jerk"=-0.0, "heading"=-0.0}, {"dt"=0.005, "x"=21.283937500000388, "y"=232.0, "position"=-21.283968750000387, "velocity"=-46.00000000000577, "acceleration"=-50.00000000023874, "jerk"=-5.6843418860808015e-08, "heading"=-0.0}, {"dt"=0.005, "x"=21.515187500000412, "y"=232.0, "position"=-21.51521875000041, "velocity"=-46.25000000000483, "acceleration"=-49.99999999981242, "jerk"=8.526512829121202e-08, "heading"=-0.0}, {"dt"=0.005, "x"=21.74768750000044, "y"=232.0, "position"=-21.747718750000438, "velocity"=-46.500000000005315, "acceleration"=-50.000000000096634, "jerk"=-5.6843418860808015e-08, "heading"=-0.0}, {"dt"=0.005, "x"=21.981437500000467, "y"=232.0, "position"=-21.981468750000467, "velocity"=-46.7500000000058, "acceleration"=-50.000000000096634, "jerk"=-0.0, "heading"=-0.0}, {"dt"=0.005, "x"=22.21643750000049, "y"=232.0, "position"=-22.21646875000049, "velocity"=-47.00000000000486, "acceleration"=-49.99999999981242, "jerk"=5.6843418860808015e-08, "heading"=-0.0}, {"dt"=0.005, "x"=22.45268750000052, "y"=232.0, "position"=-22.452718750000518, "velocity"=-47.25000000000534, "acceleration"=-50.000000000096634, "jerk"=-5.6843418860808015e-08, "heading"=-0.0}, {"dt"=0.005, "x"=22.69018750000054, "y"=232.0, "position"=-22.69021875000054, "velocity"=-47.500000000004405, "acceleration"=-49.99999999981242, "jerk"=5.6843418860808015e-08, "heading"=-0.0}, {"dt"=0.005, "x"=22.92890625000057, "y"=232.0, "position"=-22.92893750000057, "velocity"=-47.74375000000575, "acceleration"=-48.7500000002683, "jerk"=249.99999990882316, "heading"=-0.0}, {"dt"=0.005, "x"=23.168781250000595, "y"=232.0, "position"=-23.168812500000595, "velocity"=-47.97500000000525, "acceleration"=-46.24999999990109, "jerk"=500.0000000734417, "heading"=-0.0}, {"dt"=0.005, "x"=23.409750000000624, "y"=232.0, "position"=-23.409781250000623, "velocity"=-48.193750000005764, "acceleration"=-43.75000000010232, "jerk"=499.99999995975486, "heading"=-0.0}, {"dt"=0.005, "x"=23.65175000000065, "y"=232.0, "position"=-23.65178125000065, "velocity"=-48.40000000000515, "acceleration"=-41.24999999987722, "jerk"=500.00000004502, "heading"=-0.0}, {"dt"=0.005, "x"=23.894718750000678, "y"=232.0, "position"=-23.894750000000677, "velocity"=-48.59375000000554, "acceleration"=-38.750000000078444, "jerk"=499.99999995975486, "heading"=-0.0}, {"dt"=0.005, "x"=24.1385937500007, "y"=232.0, "position"=-24.1386250000007, "velocity"=-48.77500000000481, "acceleration"=-36.249999999853344, "jerk"=500.00000004502, "heading"=-0.0}, {"dt"=0.005, "x"=24.383312500000727, "y"=232.0, "position"=-24.383343750000726, "velocity"=-48.94375000000508, "acceleration"=-33.75000000005457, "jerk"=499.99999995975486, "heading"=-0.0}, {"dt"=0.005, "x"=24.62881250000076, "y"=232.0, "position"=-24.628843750000758, "velocity"=-49.10000000000636, "acceleration"=-31.250000000255795, "jerk"=499.99999995975486, "heading"=-0.0}, {"dt"=0.005, "x"=24.875031250000788, "y"=232.0, "position"=-24.875062500000787, "velocity"=-49.243750000005804, "acceleration"=-28.749999999888587, "jerk"=500.0000000734417, "heading"=-0.0}, {"dt"=0.005, "x"=25.121906250000812, "y"=232.0, "position"=-25.12193750000081, "velocity"=-49.37500000000483, "acceleration"=-26.249999999805596, "jerk"=500.0000000165983, "heading"=-0.0}, {"dt"=0.005, "x"=25.36937500000084, "y"=232.0, "position"=-25.36940625000084, "velocity"=-49.493750000005576, "acceleration"=-23.75000000014893, "jerk"=499.99999993133315, "heading"=-0.0}, {"dt"=0.005, "x"=25.61737500000087, "y"=232.0, "position"=-25.61740625000087, "velocity"=-49.600000000005906, "acceleration"=-21.25000000006594, "jerk"=500.0000000165983, "heading"=-0.0}, {"dt"=0.005, "x"=25.865843750000895, "y"=232.0, "position"=-25.865875000000894, "velocity"=-49.69375000000511, "acceleration"=-18.74999999984084, "jerk"=500.00000004502, "heading"=-0.0}, {"dt"=0.005, "x"=26.114718750000925, "y"=232.0, "position"=-26.114750000000925, "velocity"=-49.77500000000603, "acceleration"=-16.250000000184173, "jerk"=499.99999993133315, "heading"=-0.0}, {"dt"=0.005, "x"=26.363937500000954, "y"=232.0, "position"=-26.363968750000954, "velocity"=-49.84375000000583, "acceleration"=-13.749999999959073, "jerk"=500.00000004502, "heading"=-0.0}, {"dt"=0.005, "x"=26.61343750000098, "y"=232.0, "position"=-26.61346875000098, "velocity"=-49.90000000000521, "acceleration"=-11.249999999876081, "jerk"=500.0000000165983, "heading"=-0.0}, {"dt"=0.005, "x"=26.86315625000101, "y"=232.0, "position"=-26.863187500001008, "velocity"=-49.94375000000559, "acceleration"=-8.750000000077307, "jerk"=499.99999995975486, "heading"=-0.0}, {"dt"=0.005, "x"=27.11303125000104, "y"=232.0, "position"=-27.11306250000104, "velocity"=-49.975000000006276, "acceleration"=-6.250000000136424, "jerk"=499.99999998817657, "heading"=-0.0}, {"dt"=0.005, "x"=27.363000000001062, "y"=232.0, "position"=-27.36303125000106, "velocity"=-49.99375000000441, "acceleration"=-3.749999999627107, "jerk"=500.0000001018634, "heading"=-0.0}, {"dt"=0.005, "x"=27.613000000001094, "y"=232.0, "position"=-27.613031250001093, "velocity"=-50.000000000006395, "acceleration"=-1.250000000396767, "jerk"=499.999999846068, "heading"=-0.0}, {"dt"=0.005, "x"=27.86300000000112, "y"=232.0, "position"=-27.863031250001118, "velocity"=-50.000000000004974, "acceleration"=2.842170943040401e-10, "jerk"=250.00000013619683, "heading"=-0.0}, {"dt"=0.005, "x"=28.113000000001147, "y"=232.0, "position"=-28.113031250001146, "velocity"=-50.000000000005684, "acceleration"=-1.4210854715202004e-10, "jerk"=-8.526512829121202e-08, "heading"=-0.0}, {"dt"=0.005, "x"=28.363000000001172, "y"=232.0, "position"=-28.36303125000117, "velocity"=-50.000000000004974, "acceleration"=1.4210854715202004e-10, "jerk"=5.6843418860808015e-08, "heading"=-0.0}, {"dt"=0.005, "x"=28.6130000000012, "y"=232.0, "position"=-28.6130312500012, "velocity"=-50.000000000005684, "acceleration"=-1.4210854715202004e-10, "jerk"=-5.6843418860808015e-08, "heading"=-0.0}, {"dt"=0.005, "x"=28.863000000001232, "y"=232.0, "position"=-28.86303125000123, "velocity"=-50.000000000006395, "acceleration"=-1.4210854715202004e-10, "jerk"=-0.0, "heading"=-0.0}, {"dt"=0.005, "x"=29.113000000001257, "y"=232.0, "position"=-29.113031250001256, "velocity"=-50.000000000004974, "acceleration"=2.842170943040401e-10, "jerk"=8.526512829121202e-08, "heading"=-0.0}, {"dt"=0.005, "x"=29.363000000001282, "y"=232.0, "position"=-29.36303125000128, "velocity"=-50.000000000004974, "acceleration"=-0.0, "jerk"=-5.6843418860808015e-08, "heading"=-0.0}, {"dt"=0.005, "x"=29.61300000000131, "y"=232.0, "position"=-29.61303125000131, "velocity"=-50.000000000005684, "acceleration"=-1.4210854715202004e-10, "jerk"=-2.8421709430404007e-08, "heading"=-0.0}, {"dt"=0.005, "x"=29.863000000001342, "y"=232.0, "position"=-29.86303125000134, "velocity"=-50.000000000006395, "acceleration"=-1.4210854715202004e-10, "jerk"=-0.0, "heading"=-0.0}, {"dt"=0.005, "x"=30.113000000001367, "y"=232.0, "position"=-30.113031250001367, "velocity"=-50.000000000004974, "acceleration"=2.842170943040401e-10, "jerk"=8.526512829121202e-08, "heading"=-0.0}, {"dt"=0.005, "x"=30.363000000001392, "y"=232.0, "position"=-30.36303125000139, "velocity"=-50.000000000004974, "acceleration"=-0.0, "jerk"=-5.6843418860808015e-08, "heading"=-0.0}, {"dt"=0.005, "x"=30.613000000001417, "y"=232.0, "position"=-30.613031250001416, "velocity"=-50.000000000004974, "acceleration"=-0.0, "jerk"=-0.0, "heading"=-0.0}, {"dt"=0.005, "x"=30.86300000000145, "y"=232.0, "position"=-30.86303125000145, "velocity"=-50.000000000006395, "acceleration"=-2.842170943040401e-10, "jerk"=-5.6843418860808015e-08, "heading"=-0.0}, {"dt"=0.005, "x"=31.113000000001477, "y"=232.0, "position"=-31.113031250001477, "velocity"=-50.000000000005684, "acceleration"=1.4210854715202004e-10, "jerk"=8.526512829121202e-08, "heading"=-0.0}, {"dt"=0.005, "x"=31.36300000000151, "y"=232.0, "position"=-31.36303125000151, "velocity"=-50.000000000006395, "acceleration"=-1.4210854715202004e-10, "jerk"=-5.6843418860808015e-08, "heading"=-0.0}, {"dt"=0.005, "x"=31.613000000001534, "y"=232.0, "position"=-31.613031250001534, "velocity"=-50.000000000004974, "acceleration"=2.842170943040401e-10, "jerk"=8.526512829121202e-08, "heading"=-0.0}, {"dt"=0.005, "x"=31.86300000000156, "y"=232.0, "position"=-31.86303125000156, "velocity"=-50.000000000004974, "acceleration"=-0.0, "jerk"=-5.6843418860808015e-08, "heading"=-0.0}, {"dt"=0.005, "x"=32.113000000001584, "y"=232.0, "position"=-32.11303125000158, "velocity"=-50.000000000004974, "acceleration"=-0.0, "jerk"=-0.0, "heading"=-0.0}, {"dt"=0.005, "x"=32.36300000000161, "y"=232.0, "position"=-32.36303125000161, "velocity"=-50.000000000005684, "acceleration"=-1.4210854715202004e-10, "jerk"=-2.8421709430404007e-08, "heading"=-0.0}, {"dt"=0.005, "x"=32.613000000001634, "y"=232.0, "position"=-32.61303125000163, "velocity"=-50.00000000000426, "acceleration"=2.842170943040401e-10, "jerk"=8.526512829121202e-08, "heading"=-0.0}, {"dt"=0.005, "x"=32.86300000000167, "y"=232.0, "position"=-32.86303125000167, "velocity"=-50.000000000007105, "acceleration"=-5.684341886080801e-10, "jerk"=-1.7053025658242404e-07, "heading"=-0.0}, {"dt"=0.005, "x"=33.113000000001705, "y"=232.0, "position"=-33.113031250001704, "velocity"=-50.000000000007105, "acceleration"=-0.0, "jerk"=1.1368683772161603e-07, "heading"=-0.0}, {"dt"=0.005, "x"=33.363000000001726, "y"=232.0, "position"=-33.363031250001725, "velocity"=-50.00000000000426, "acceleration"=5.684341886080801e-10, "jerk"=1.1368683772161603e-07, "heading"=-0.0}, {"dt"=0.005, "x"=33.613000000001755, "y"=232.0, "position"=-33.613031250001754, "velocity"=-50.000000000005684, "acceleration"=-2.842170943040401e-10, "jerk"=-1.7053025658242404e-07, "heading"=-0.0}, {"dt"=0.005, "x"=33.863000000001776, "y"=232.0, "position"=-33.863031250001775, "velocity"=-50.00000000000426, "acceleration"=2.842170943040401e-10, "jerk"=1.1368683772161603e-07, "heading"=-0.0}, {"dt"=0.005, "x"=34.113000000001804, "y"=232.0, "position"=-34.113031250001804, "velocity"=-50.000000000005684, "acceleration"=-2.842170943040401e-10, "jerk"=-1.1368683772161603e-07, "heading"=-0.0}, {"dt"=0.005, "x"=34.36300000000183, "y"=232.0, "position"=-34.36303125000183, "velocity"=-50.000000000005684, "acceleration"=-0.0, "jerk"=5.6843418860808015e-08, "heading"=-0.0}, {"dt"=0.005, "x"=34.61300000000186, "y"=232.0, "position"=-34.61303125000186, "velocity"=-50.000000000005684, "acceleration"=-0.0, "jerk"=-0.0, "heading"=-0.0}, {"dt"=0.005, "x"=34.8630000000019, "y"=232.0, "position"=-34.863031250001896, "velocity"=-50.000000000007105, "acceleration"=-2.842170943040401e-10, "jerk"=-5.6843418860808015e-08, "heading"=-0.0}, {"dt"=0.005, "x"=35.11300000000192, "y"=232.0, "position"=-35.11303125000192, "velocity"=-50.00000000000426, "acceleration"=5.684341886080801e-10, "jerk"=1.7053025658242404e-07, "heading"=-0.0}, {"dt"=0.005, "x"=35.363000000001946, "y"=232.0, "position"=-35.363031250001946, "velocity"=-50.000000000005684, "acceleration"=-2.842170943040401e-10, "jerk"=-1.7053025658242404e-07, "heading"=-0.0}, {"dt"=0.005, "x"=35.613000000001975, "y"=232.0, "position"=-35.613031250001974, "velocity"=-50.000000000005684, "acceleration"=-0.0, "jerk"=5.6843418860808015e-08, "heading"=-0.0}, {"dt"=0.005, "x"=35.863000000001996, "y"=232.0, "position"=-35.863031250001995, "velocity"=-50.00000000000426, "acceleration"=2.842170943040401e-10, "jerk"=5.6843418860808015e-08, "heading"=-0.0}, {"dt"=0.005, "x"=36.113000000002025, "y"=232.0, "position"=-36.113031250002024, "velocity"=-50.000000000005684, "acceleration"=-2.842170943040401e-10, "jerk"=-1.1368683772161603e-07, "heading"=-0.0}, {"dt"=0.005, "x"=36.36300000000205, "y"=232.0, "position"=-36.36303125000205, "velocity"=-50.000000000005684, "acceleration"=-0.0, "jerk"=5.6843418860808015e-08, "heading"=-0.0}, {"dt"=0.005, "x"=36.61300000000209, "y"=232.0, "position"=-36.61303125000209, "velocity"=-50.000000000007105, "acceleration"=-2.842170943040401e-10, "jerk"=-5.6843418860808015e-08, "heading"=-0.0}, {"dt"=0.005, "x"=36.86300000000211, "y"=232.0, "position"=-36.86303125000211, "velocity"=-50.00000000000426, "acceleration"=5.684341886080801e-10, "jerk"=1.7053025658242404e-07, "heading"=-0.0}, {"dt"=0.005, "x"=37.11300000000214, "y"=232.0, "position"=-37.11303125000214, "velocity"=-50.000000000005684, "acceleration"=-2.842170943040401e-10, "jerk"=-1.7053025658242404e-07, "heading"=-0.0}, {"dt"=0.005, "x"=37.36300000000217, "y"=232.0, "position"=-37.363031250002166, "velocity"=-50.000000000005684, "acceleration"=-0.0, "jerk"=5.6843418860808015e-08, "heading"=-0.0}, {"dt"=0.005, "x"=37.613000000002195, "y"=232.0, "position"=-37.613031250002194, "velocity"=-50.000000000005684, "acceleration"=-0.0, "jerk"=-0.0, "heading"=-0.0}, {"dt"=0.005, "x"=37.863000000002216, "y"=232.0, "position"=-37.863031250002216, "velocity"=-50.00000000000426, "acceleration"=2.842170943040401e-10, "jerk"=5.6843418860808015e-08, "heading"=-0.0}, {"dt"=0.005, "x"=38.113000000002245, "y"=232.0, "position"=-38.113031250002244, "velocity"=-50.000000000005684, "acceleration"=-2.842170943040401e-10, "jerk"=-1.1368683772161603e-07, "heading"=-0.0}, {"dt"=0.005, "x"=38.36300000000227, "y"=232.0, "position"=-38.36303125000227, "velocity"=-50.000000000005684, "acceleration"=-0.0, "jerk"=5.6843418860808015e-08, "heading"=-0.0}, {"dt"=0.005, "x"=38.6130000000023, "y"=232.0, "position"=-38.6130312500023, "velocity"=-50.000000000005684, "acceleration"=-0.0, "jerk"=-0.0, "heading"=-0.0}, {"dt"=0.005, "x"=38.86300000000234, "y"=232.0, "position"=-38.86303125000234, "velocity"=-50.000000000007105, "acceleration"=-2.842170943040401e-10, "jerk"=-5.6843418860808015e-08, "heading"=-0.0}, {"dt"=0.005, "x"=39.11300000000236, "y"=232.0, "position"=-39.11303125000236, "velocity"=-50.00000000000426, "acceleration"=5.684341886080801e-10, "jerk"=1.7053025658242404e-07, "heading"=-0.0}, {"dt"=0.005, "x"=39.36300000000239, "y"=232.0, "position"=-39.363031250002386, "velocity"=-50.000000000005684, "acceleration"=-2.842170943040401e-10, "jerk"=-1.7053025658242404e-07, "heading"=-0.0}, {"dt"=0.005, "x"=39.613000000002415, "y"=232.0, "position"=-39.613031250002415, "velocity"=-50.000000000005684, "acceleration"=-0.0, "jerk"=5.6843418860808015e-08, "heading"=-0.0}, {"dt"=0.005, "x"=39.86300000000244, "y"=232.0, "position"=-39.863031250002436, "velocity"=-50.00000000000426, "acceleration"=2.842170943040401e-10, "jerk"=5.6843418860808015e-08, "heading"=-0.0}, {"dt"=0.005, "x"=40.113000000002465, "y"=232.0, "position"=-40.113031250002464, "velocity"=-50.000000000005684, "acceleration"=-2.842170943040401e-10, "jerk"=-1.1368683772161603e-07, "heading"=-0.0}, {"dt"=0.005, "x"=40.36300000000249, "y"=232.0, "position"=-40.36303125000249, "velocity"=-50.000000000005684, "acceleration"=-0.0, "jerk"=5.6843418860808015e-08, "heading"=-0.0}, {"dt"=0.005, "x"=40.61300000000253, "y"=232.0, "position"=-40.61303125000253, "velocity"=-50.000000000007105, "acceleration"=-2.842170943040401e-10, "jerk"=-5.6843418860808015e-08, "heading"=-0.0}, {"dt"=0.005, "x"=40.86300000000256, "y"=232.0, "position"=-40.86303125000256, "velocity"=-50.000000000005684, "acceleration"=2.842170943040401e-10, "jerk"=1.1368683772161603e-07, "heading"=-0.0}, {"dt"=0.005, "x"=41.11300000000258, "y"=232.0, "position"=-41.11303125000258, "velocity"=-50.00000000000426, "acceleration"=2.842170943040401e-10, "jerk"=-0.0, "heading"=-0.0}, {"dt"=0.005, "x"=41.36300000000261, "y"=232.0, "position"=-41.36303125000261, "velocity"=-50.000000000005684, "acceleration"=-2.842170943040401e-10, "jerk"=-1.1368683772161603e-07, "heading"=-0.0}, {"dt"=0.005, "x"=41.61300000000263, "y"=232.0, "position"=-41.61303125000263, "velocity"=-50.00000000000426, "acceleration"=2.842170943040401e-10, "jerk"=1.1368683772161603e-07, "heading"=-0.0}, {"dt"=0.005, "x"=41.86300000000266, "y"=232.0, "position"=-41.863031250002656, "velocity"=-50.000000000005684, "acceleration"=-2.842170943040401e-10, "jerk"=-1.1368683772161603e-07, "heading"=-0.0}, {"dt"=0.005, "x"=42.11300000000269, "y"=232.0, "position"=-42.11303125000269, "velocity"=-50.000000000007105, "acceleration"=-2.842170943040401e-10, "jerk"=-0.0, "heading"=-0.0}, {"dt"=0.005, "x"=42.36300000000272, "y"=232.0, "position"=-42.36303125000272, "velocity"=-50.000000000005684, "acceleration"=2.842170943040401e-10, "jerk"=1.1368683772161603e-07, "heading"=-0.0}, {"dt"=0.005, "x"=42.61300000000275, "y"=232.0, "position"=-42.61303125000275, "velocity"=-50.000000000005684, "acceleration"=-0.0, "jerk"=-5.6843418860808015e-08, "heading"=-0.0}, {"dt"=0.005, "x"=42.86300000000277, "y"=232.0, "position"=-42.86303125000277, "velocity"=-50.00000000000426, "acceleration"=2.842170943040401e-10, "jerk"=5.6843418860808015e-08, "heading"=-0.0}, {"dt"=0.005, "x"=43.1130000000028, "y"=232.0, "position"=-43.1130312500028, "velocity"=-50.000000000005684, "acceleration"=-2.842170943040401e-10, "jerk"=-1.1368683772161603e-07, "heading"=-0.0}, {"dt"=0.005, "x"=43.36300000000283, "y"=232.0, "position"=-43.36303125000283, "velocity"=-50.000000000005684, "acceleration"=-0.0, "jerk"=5.6843418860808015e-08, "heading"=-0.0}, {"dt"=0.005, "x"=43.61300000000285, "y"=232.0, "position"=-43.61303125000285, "velocity"=-50.00000000000426, "acceleration"=2.842170943040401e-10, "jerk"=5.6843418860808015e-08, "heading"=-0.0}, {"dt"=0.005, "x"=43.86300000000288, "y"=232.0, "position"=-43.86303125000288, "velocity"=-50.000000000005684, "acceleration"=-2.842170943040401e-10, "jerk"=-1.1368683772161603e-07, "heading"=-0.0}, {"dt"=0.005, "x"=44.11300000000291, "y"=232.0, "position"=-44.11303125000291, "velocity"=-50.000000000007105, "acceleration"=-2.842170943040401e-10, "jerk"=-0.0, "heading"=-0.0}, {"dt"=0.005, "x"=44.363000000002934, "y"=232.0, "position"=-44.36303125000293, "velocity"=-50.00000000000426, "acceleration"=5.684341886080801e-10, "jerk"=1.7053025658242404e-07, "heading"=-0.0}, {"dt"=0.005, "x"=44.61300000000297, "y"=232.0, "position"=-44.61303125000297, "velocity"=-50.000000000007105, "acceleration"=-5.684341886080801e-10, "jerk"=-2.2737367544323206e-07, "heading"=-0.0}, {"dt"=0.005, "x"=44.86300000000299, "y"=232.0, "position"=-44.86303125000299, "velocity"=-50.00000000000426, "acceleration"=5.684341886080801e-10, "jerk"=2.2737367544323206e-07, "heading"=-0.0}, {"dt"=0.005, "x"=45.11300000000302, "y"=232.0, "position"=-45.11303125000302, "velocity"=-50.000000000005684, "acceleration"=-2.842170943040401e-10, "jerk"=-1.7053025658242404e-07, "heading"=-0.0}, {"dt"=0.005, "x"=45.36300000000304, "y"=232.0, "position"=-45.36303125000304, "velocity"=-50.00000000000426, "acceleration"=2.842170943040401e-10, "jerk"=1.1368683772161603e-07, "heading"=-0.0}, {"dt"=0.005, "x"=45.61300000000307, "y"=232.0, "position"=-45.61303125000307, "velocity"=-50.000000000005684, "acceleration"=-2.842170943040401e-10, "jerk"=-1.1368683772161603e-07, "heading"=-0.0}, {"dt"=0.005, "x"=45.863000000003105, "y"=232.0, "position"=-45.863031250003104, "velocity"=-50.000000000007105, "acceleration"=-2.842170943040401e-10, "jerk"=-0.0, "heading"=-0.0}, {"dt"=0.005, "x"=46.113000000003126, "y"=232.0, "position"=-46.113031250003125, "velocity"=-50.00000000000426, "acceleration"=5.684341886080801e-10, "jerk"=1.7053025658242404e-07, "heading"=-0.0}, {"dt"=0.005, "x"=46.36300000000316, "y"=232.0, "position"=-46.36303125000316, "velocity"=-50.000000000007105, "acceleration"=-5.684341886080801e-10, "jerk"=-2.2737367544323206e-07, "heading"=-0.0}, {"dt"=0.005, "x"=46.61300000000318, "y"=232.0, "position"=-46.61303125000318, "velocity"=-50.00000000000426, "acceleration"=5.684341886080801e-10, "jerk"=2.2737367544323206e-07, "heading"=-0.0}, {"dt"=0.005, "x"=46.86300000000321, "y"=232.0, "position"=-46.86303125000321, "velocity"=-50.000000000005684, "acceleration"=-2.842170943040401e-10, "jerk"=-1.7053025658242404e-07, "heading"=-0.0}, {"dt"=0.005, "x"=47.11300000000324, "y"=232.0, "position"=-47.11303125000324, "velocity"=-50.000000000005684, "acceleration"=-0.0, "jerk"=5.6843418860808015e-08, "heading"=-0.0}, {"dt"=0.005, "x"=47.36300000000326, "y"=232.0, "position"=-47.36303125000326, "velocity"=-50.00000000000426, "acceleration"=2.842170943040401e-10, "jerk"=5.6843418860808015e-08, "heading"=-0.0}, {"dt"=0.005, "x"=47.61300000000329, "y"=232.0, "position"=-47.61303125000329, "velocity"=-50.000000000005684, "acceleration"=-2.842170943040401e-10, "jerk"=-1.1368683772161603e-07, "heading"=-0.0}, {"dt"=0.005, "x"=47.863000000003325, "y"=232.0, "position"=-47.863031250003324, "velocity"=-50.000000000007105, "acceleration"=-2.842170943040401e-10, "jerk"=-0.0, "heading"=-0.0}, {"dt"=0.005, "x"=48.11300000000335, "y"=232.0, "position"=-48.11303125000335, "velocity"=-50.000000000005684, "acceleration"=2.842170943040401e-10, "jerk"=1.1368683772161603e-07, "heading"=-0.0}, {"dt"=0.005, "x"=48.36300000000338, "y"=232.0, "position"=-48.36303125000338, "velocity"=-50.000000000005684, "acceleration"=-0.0, "jerk"=-5.6843418860808015e-08, "heading"=-0.0}, {"dt"=0.005, "x"=48.6130000000034, "y"=232.0, "position"=-48.6130312500034, "velocity"=-50.00000000000426, "acceleration"=2.842170943040401e-10, "jerk"=5.6843418860808015e-08, "heading"=-0.0}, {"dt"=0.005, "x"=48.86300000000343, "y"=232.0, "position"=-48.86303125000343, "velocity"=-50.000000000005684, "acceleration"=-2.842170943040401e-10, "jerk"=-1.1368683772161603e-07, "heading"=-0.0}, {"dt"=0.005, "x"=49.11300000000346, "y"=232.0, "position"=-49.11303125000346, "velocity"=-50.000000000005684, "acceleration"=-0.0, "jerk"=5.6843418860808015e-08, "heading"=-0.0}, {"dt"=0.005, "x"=49.36300000000348, "y"=232.0, "position"=-49.36303125000348, "velocity"=-50.00000000000426, "acceleration"=2.842170943040401e-10, "jerk"=5.6843418860808015e-08, "heading"=-0.0}, {"dt"=0.005, "x"=49.61300000000352, "y"=232.0, "position"=-49.613031250003516, "velocity"=-50.000000000007105, "acceleration"=-5.684341886080801e-10, "jerk"=-1.7053025658242404e-07, "heading"=-0.0}, {"dt"=0.005, "x"=49.863000000003545, "y"=232.0, "position"=-49.863031250003544, "velocity"=-50.000000000005684, "acceleration"=2.842170943040401e-10, "jerk"=1.7053025658242404e-07, "heading"=-0.0}, {"dt"=0.005, "x"=50.113000000003574, "y"=232.0, "position"=-50.11303125000357, "velocity"=-50.000000000005684, "acceleration"=-0.0, "jerk"=-5.6843418860808015e-08, "heading"=-0.0}, {"dt"=0.005, "x"=50.3630000000036, "y"=232.0, "position"=-50.3630312500036, "velocity"=-50.000000000005684, "acceleration"=-0.0, "jerk"=-0.0, "heading"=-0.0}, {"dt"=0.005, "x"=50.61300000000362, "y"=232.0, "position"=-50.61303125000362, "velocity"=-50.00000000000426, "acceleration"=2.842170943040401e-10, "jerk"=5.6843418860808015e-08, "heading"=-0.0}, {"dt"=0.005, "x"=50.86300000000365, "y"=232.0, "position"=-50.86303125000365, "velocity"=-50.000000000005684, "acceleration"=-2.842170943040401e-10, "jerk"=-1.1368683772161603e-07, "heading"=-0.0}, {"dt"=0.005, "x"=51.11300000000368, "y"=232.0, "position"=-51.11303125000368, "velocity"=-50.000000000005684, "acceleration"=-0.0, "jerk"=5.6843418860808015e-08, "heading"=-0.0}, {"dt"=0.005, "x"=51.3630000000037, "y"=232.0, "position"=-51.3630312500037, "velocity"=-50.00000000000426, "acceleration"=2.842170943040401e-10, "jerk"=5.6843418860808015e-08, "heading"=-0.0}, {"dt"=0.005, "x"=51.613000000003744, "y"=232.0, "position"=-51.61303125000374, "velocity"=-50.00000000000853, "acceleration"=-8.526512829121202e-10, "jerk"=-2.2737367544323206e-07, "heading"=-0.0}, {"dt"=0.005, "x"=51.86300000000376, "y"=232.0, "position"=-51.86303125000376, "velocity"=-50.00000000000284, "acceleration"=1.1368683772161603e-09, "jerk"=3.979039320256561e-07, "heading"=-0.0}, {"dt"=0.005, "x"=52.113000000003794, "y"=232.0, "position"=-52.11303125000379, "velocity"=-50.000000000007105, "acceleration"=-8.526512829121202e-10, "jerk"=-3.979039320256561e-07, "heading"=-0.0}, {"dt"=0.005, "x"=52.36300000000382, "y"=232.0, "position"=-52.36303125000382, "velocity"=-50.000000000005684, "acceleration"=2.842170943040401e-10, "jerk"=2.2737367544323206e-07, "heading"=-0.0}, {"dt"=0.005, "x"=52.613000000003844, "y"=232.0, "position"=-52.61303125000384, "velocity"=-50.00000000000426, "acceleration"=2.842170943040401e-10, "jerk"=-0.0, "heading"=-0.0}, {"dt"=0.005, "x"=52.86300000000387, "y"=232.0, "position"=-52.86303125000387, "velocity"=-50.000000000005684, "acceleration"=-2.842170943040401e-10, "jerk"=-1.1368683772161603e-07, "heading"=-0.0}, {"dt"=0.005, "x"=53.11300000000389, "y"=232.0, "position"=-53.11303125000389, "velocity"=-50.00000000000426, "acceleration"=2.842170943040401e-10, "jerk"=1.1368683772161603e-07, "heading"=-0.0}, {"dt"=0.005, "x"=53.36300000000393, "y"=232.0, "position"=-53.36303125000393, "velocity"=-50.000000000007105, "acceleration"=-5.684341886080801e-10, "jerk"=-1.7053025658242404e-07, "heading"=-0.0}, {"dt"=0.005, "x"=53.61300000000396, "y"=232.0, "position"=-53.61303125000396, "velocity"=-50.000000000005684, "acceleration"=2.842170943040401e-10, "jerk"=1.7053025658242404e-07, "heading"=-0.0}, {"dt"=0.005, "x"=53.863000000003986, "y"=232.0, "position"=-53.863031250003985, "velocity"=-50.000000000005684, "acceleration"=-0.0, "jerk"=-5.6843418860808015e-08, "heading"=-0.0}, {"dt"=0.005, "x"=54.113000000004014, "y"=232.0, "position"=-54.11303125000401, "velocity"=-50.000000000005684, "acceleration"=-0.0, "jerk"=-0.0, "heading"=-0.0}, {"dt"=0.005, "x"=54.363000000004035, "y"=232.0, "position"=-54.363031250004035, "velocity"=-50.00000000000426, "acceleration"=2.842170943040401e-10, "jerk"=5.6843418860808015e-08, "heading"=-0.0}, {"dt"=0.005, "x"=54.613000000004064, "y"=232.0, "position"=-54.61303125000406, "velocity"=-50.000000000005684, "acceleration"=-2.842170943040401e-10, "jerk"=-1.1368683772161603e-07, "heading"=-0.0}, {"dt"=0.005, "x"=54.86300000000409, "y"=232.0, "position"=-54.86303125000409, "velocity"=-50.000000000005684, "acceleration"=-0.0, "jerk"=5.6843418860808015e-08, "heading"=-0.0}, {"dt"=0.005, "x"=55.113000000004114, "y"=232.0, "position"=-55.11303125000411, "velocity"=-50.00000000000426, "acceleration"=2.842170943040401e-10, "jerk"=5.6843418860808015e-08, "heading"=-0.0}, {"dt"=0.005, "x"=55.36300000000415, "y"=232.0, "position"=-55.36303125000415, "velocity"=-50.000000000007105, "acceleration"=-5.684341886080801e-10, "jerk"=-1.7053025658242404e-07, "heading"=-0.0}, {"dt"=0.005, "x"=55.61300000000418, "y"=232.0, "position"=-55.61303125000418, "velocity"=-50.000000000005684, "acceleration"=2.842170943040401e-10, "jerk"=1.7053025658242404e-07, "heading"=-0.0}, {"dt"=0.005, "x"=55.863000000004206, "y"=232.0, "position"=-55.863031250004205, "velocity"=-50.000000000005684, "acceleration"=-0.0, "jerk"=-5.6843418860808015e-08, "heading"=-0.0}, {"dt"=0.005, "x"=56.113000000004234, "y"=232.0, "position"=-56.113031250004234, "velocity"=-50.000000000005684, "acceleration"=-0.0, "jerk"=-0.0, "heading"=-0.0}, {"dt"=0.005, "x"=56.363000000004256, "y"=232.0, "position"=-56.363031250004255, "velocity"=-50.00000000000426, "acceleration"=2.842170943040401e-10, "jerk"=5.6843418860808015e-08, "heading"=-0.0}, {"dt"=0.005, "x"=56.613000000004284, "y"=232.0, "position"=-56.61303125000428, "velocity"=-50.000000000005684, "acceleration"=-2.842170943040401e-10, "jerk"=-1.1368683772161603e-07, "heading"=-0.0}, {"dt"=0.005, "x"=56.863000000004305, "y"=232.0, "position"=-56.863031250004305, "velocity"=-50.00000000000426, "acceleration"=2.842170943040401e-10, "jerk"=1.1368683772161603e-07, "heading"=-0.0}, {"dt"=0.005, "x"=57.11300000000434, "y"=232.0, "position"=-57.11303125000434, "velocity"=-50.000000000007105, "acceleration"=-5.684341886080801e-10, "jerk"=-1.7053025658242404e-07, "heading"=-0.0}, {"dt"=0.005, "x"=57.36300000000438, "y"=232.0, "position"=-57.363031250004376, "velocity"=-50.000000000007105, "acceleration"=-0.0, "jerk"=1.1368683772161603e-07, "heading"=-0.0}, {"dt"=0.005, "x"=57.6130000000044, "y"=232.0, "position"=-57.6130312500044, "velocity"=-50.00000000000426, "acceleration"=5.684341886080801e-10, "jerk"=1.1368683772161603e-07, "heading"=-0.0}, {"dt"=0.005, "x"=57.863000000004426, "y"=232.0, "position"=-57.863031250004425, "velocity"=-50.000000000005684, "acceleration"=-2.842170943040401e-10, "jerk"=-1.7053025658242404e-07, "heading"=-0.0}, {"dt"=0.005, "x"=58.11300000000445, "y"=232.0, "position"=-58.11303125000445, "velocity"=-50.00000000000426, "acceleration"=2.842170943040401e-10, "jerk"=1.1368683772161603e-07, "heading"=-0.0}, {"dt"=0.005, "x"=58.363000000004476, "y"=232.0, "position"=-58.363031250004475, "velocity"=-50.000000000005684, "acceleration"=-2.842170943040401e-10, "jerk"=-1.1368683772161603e-07, "heading"=-0.0}, {"dt"=0.005, "x"=58.613000000004504, "y"=232.0, "position"=-58.613031250004504, "velocity"=-50.000000000005684, "acceleration"=-0.0, "jerk"=5.6843418860808015e-08, "heading"=-0.0}, {"dt"=0.005, "x"=58.863000000004526, "y"=232.0, "position"=-58.863031250004525, "velocity"=-50.00000000000426, "acceleration"=2.842170943040401e-10, "jerk"=5.6843418860808015e-08, "heading"=-0.0}, {"dt"=0.005, "x"=59.11300000000457, "y"=232.0, "position"=-59.11303125000457, "velocity"=-50.00000000000853, "acceleration"=-8.526512829121202e-10, "jerk"=-2.2737367544323206e-07, "heading"=-0.0}, {"dt"=0.005, "x"=59.36300000000459, "y"=232.0, "position"=-59.36303125000459, "velocity"=-50.00000000000426, "acceleration"=8.526512829121202e-10, "jerk"=3.410605131648481e-07, "heading"=-0.0}, {"dt"=0.005, "x"=59.61300000000462, "y"=232.0, "position"=-59.61303125000462, "velocity"=-50.000000000005684, "acceleration"=-2.842170943040401e-10, "jerk"=-2.2737367544323206e-07, "heading"=-0.0}, {"dt"=0.005, "x"=59.86300000000465, "y"=232.0, "position"=-59.863031250004646, "velocity"=-50.000000000005684, "acceleration"=-0.0, "jerk"=5.6843418860808015e-08, "heading"=-0.0}, {"dt"=0.005, "x"=60.11300000000467, "y"=232.0, "position"=-60.11303125000467, "velocity"=-50.00000000000426, "acceleration"=2.842170943040401e-10, "jerk"=5.6843418860808015e-08, "heading"=-0.0}, {"dt"=0.005, "x"=60.363000000004696, "y"=232.0, "position"=-60.363031250004695, "velocity"=-50.000000000005684, "acceleration"=-2.842170943040401e-10, "jerk"=-1.1368683772161603e-07, "heading"=-0.0}, {"dt"=0.005, "x"=60.613000000004725, "y"=232.0, "position"=-60.613031250004724, "velocity"=-50.000000000005684, "acceleration"=-0.0, "jerk"=5.6843418860808015e-08, "heading"=-0.0}, {"dt"=0.005, "x"=60.863000000004746, "y"=232.0, "position"=-60.863031250004745, "velocity"=-50.00000000000426, "acceleration"=2.842170943040401e-10, "jerk"=5.6843418860808015e-08, "heading"=-0.0}, {"dt"=0.005, "x"=61.113000000004774, "y"=232.0, "position"=-61.113031250004774, "velocity"=-50.000000000005684, "acceleration"=-2.842170943040401e-10, "jerk"=-1.1368683772161603e-07, "heading"=-0.0}, {"dt"=0.005, "x"=61.3630000000048, "y"=232.0, "position"=-61.3630312500048, "velocity"=-50.000000000005684, "acceleration"=-0.0, "jerk"=5.6843418860808015e-08, "heading"=-0.0}, {"dt"=0.005, "x"=61.613000000004824, "y"=232.0, "position"=-61.61303125000482, "velocity"=-50.00000000000426, "acceleration"=2.842170943040401e-10, "jerk"=5.6843418860808015e-08, "heading"=-0.0}, {"dt"=0.005, "x"=61.86300000000487, "y"=232.0, "position"=-61.863031250004866, "velocity"=-50.00000000000853, "acceleration"=-8.526512829121202e-10, "jerk"=-2.2737367544323206e-07, "heading"=-0.0}, {"dt"=0.005, "x"=62.1130000000049, "y"=232.0, "position"=-62.1130312500049, "velocity"=-50.000000000007105, "acceleration"=2.842170943040401e-10, "jerk"=2.2737367544323206e-07, "heading"=-0.0}, {"dt"=0.005, "x"=62.36300000000493, "y"=232.0, "position"=-62.36303125000493, "velocity"=-50.000000000005684, "acceleration"=2.842170943040401e-10, "jerk"=-0.0, "heading"=-0.0}, {"dt"=0.005, "x"=62.61300000000495, "y"=232.0, "position"=-62.61303125000495, "velocity"=-50.00000000000426, "acceleration"=2.842170943040401e-10, "jerk"=-0.0, "heading"=-0.0}, {"dt"=0.005, "x"=62.86300000000498, "y"=232.0, "position"=-62.86303125000498, "velocity"=-50.000000000005684, "acceleration"=-2.842170943040401e-10, "jerk"=-1.1368683772161603e-07, "heading"=-0.0}, {"dt"=0.005, "x"=63.11300000000501, "y"=232.0, "position"=-63.11303125000501, "velocity"=-50.000000000005684, "acceleration"=-0.0, "jerk"=5.6843418860808015e-08, "heading"=-0.0}, {"dt"=0.005, "x"=63.36300000000503, "y"=232.0, "position"=-63.36303125000503, "velocity"=-50.00000000000426, "acceleration"=2.842170943040401e-10, "jerk"=5.6843418860808015e-08, "heading"=-0.0}, {"dt"=0.005, "x"=63.61300000000506, "y"=232.0, "position"=-63.61303125000506, "velocity"=-50.000000000005684, "acceleration"=-2.842170943040401e-10, "jerk"=-1.1368683772161603e-07, "heading"=-0.0}, {"dt"=0.005, "x"=63.86300000000509, "y"=232.0, "position"=-63.863031250005086, "velocity"=-50.000000000005684, "acceleration"=-0.0, "jerk"=5.6843418860808015e-08, "heading"=-0.0}, {"dt"=0.005, "x"=64.11300000000512, "y"=232.0, "position"=-64.11303125000512, "velocity"=-50.000000000005684, "acceleration"=-0.0, "jerk"=-0.0, "heading"=-0.0}, {"dt"=0.005, "x"=64.36300000000513, "y"=232.0, "position"=-64.36303125000514, "velocity"=-50.00000000000284, "acceleration"=5.684341886080801e-10, "jerk"=1.1368683772161603e-07, "heading"=-0.0}, {"dt"=0.005, "x"=64.61300000000516, "y"=232.0, "position"=-64.61303125000516, "velocity"=-50.000000000005684, "acceleration"=-5.684341886080801e-10, "jerk"=-2.2737367544323206e-07, "heading"=-0.0}, {"dt"=0.005, "x"=64.86300000000519, "y"=232.0, "position"=-64.86303125000519, "velocity"=-50.000000000005684, "acceleration"=-0.0, "jerk"=1.1368683772161603e-07, "heading"=-0.0}, {"dt"=0.005, "x"=65.11300000000521, "y"=232.0, "position"=-65.11303125000522, "velocity"=-50.000000000005684, "acceleration"=-0.0, "jerk"=-0.0, "heading"=-0.0}, {"dt"=0.005, "x"=65.36300000000524, "y"=232.0, "position"=-65.36303125000525, "velocity"=-50.000000000005684, "acceleration"=-0.0, "jerk"=-0.0, "heading"=-0.0}, {"dt"=0.005, "x"=65.61300000000526, "y"=232.0, "position"=-65.61303125000526, "velocity"=-50.00000000000284, "acceleration"=5.684341886080801e-10, "jerk"=1.1368683772161603e-07, "heading"=-0.0}, {"dt"=0.005, "x"=65.8630000000053, "y"=232.0, "position"=-65.8630312500053, "velocity"=-50.00000000000853, "acceleration"=-1.1368683772161603e-09, "jerk"=-3.410605131648481e-07, "heading"=-0.0}, {"dt"=0.005, "x"=66.11300000000533, "y"=232.0, "position"=-66.11303125000533, "velocity"=-50.000000000005684, "acceleration"=5.684341886080801e-10, "jerk"=3.410605131648481e-07, "heading"=-0.0}, {"dt"=0.005, "x"=66.36300000000536, "y"=232.0, "position"=-66.36303125000536, "velocity"=-50.000000000005684, "acceleration"=-0.0, "jerk"=-1.1368683772161603e-07, "heading"=-0.0}, {"dt"=0.005, "x"=66.61300000000539, "y"=232.0, "position"=-66.61303125000539, "velocity"=-50.000000000005684, "acceleration"=-0.0, "jerk"=-0.0, "heading"=-0.0}, {"dt"=0.005, "x"=66.8630000000054, "y"=232.0, "position"=-66.8630312500054, "velocity"=-50.00000000000284, "acceleration"=5.684341886080801e-10, "jerk"=1.1368683772161603e-07, "heading"=-0.0}, {"dt"=0.005, "x"=67.11300000000543, "y"=232.0, "position"=-67.11303125000543, "velocity"=-50.000000000005684, "acceleration"=-5.684341886080801e-10, "jerk"=-2.2737367544323206e-07, "heading"=-0.0}, {"dt"=0.005, "x"=67.36300000000546, "y"=232.0, "position"=-67.36303125000546, "velocity"=-50.000000000005684, "acceleration"=-0.0, "jerk"=1.1368683772161603e-07, "heading"=-0.0}, {"dt"=0.005, "x"=67.6130000000055, "y"=232.0, "position"=-67.6130312500055, "velocity"=-50.00000000000853, "acceleration"=-5.684341886080801e-10, "jerk"=-1.1368683772161603e-07, "heading"=-0.0}, {"dt"=0.005, "x"=67.86300000000553, "y"=232.0, "position"=-67.86303125000553, "velocity"=-50.000000000005684, "acceleration"=5.684341886080801e-10, "jerk"=2.2737367544323206e-07, "heading"=-0.0}, {"dt"=0.005, "x"=68.11300000000554, "y"=232.0, "position"=-68.11303125000555, "velocity"=-50.00000000000284, "acceleration"=5.684341886080801e-10, "jerk"=-0.0, "heading"=-0.0}, {"dt"=0.005, "x"=68.36300000000557, "y"=232.0, "position"=-68.36303125000558, "velocity"=-50.000000000005684, "acceleration"=-5.684341886080801e-10, "jerk"=-2.2737367544323206e-07, "heading"=-0.0}, {"dt"=0.005, "x"=68.6130000000056, "y"=232.0, "position"=-68.6130312500056, "velocity"=-50.000000000005684, "acceleration"=-0.0, "jerk"=1.1368683772161603e-07, "heading"=-0.0}, {"dt"=0.005, "x"=68.86300000000563, "y"=232.0, "position"=-68.86303125000563, "velocity"=-50.000000000005684, "acceleration"=-0.0, "jerk"=-0.0, "heading"=-0.0}, {"dt"=0.005, "x"=69.11300000000566, "y"=232.0, "position"=-69.11303125000566, "velocity"=-50.000000000005684, "acceleration"=-0.0, "jerk"=-0.0, "heading"=-0.0}, {"dt"=0.005, "x"=69.36300000000568, "y"=232.0, "position"=-69.36303125000569, "velocity"=-50.000000000005684, "acceleration"=-0.0, "jerk"=-0.0, "heading"=-0.0}, {"dt"=0.005, "x"=69.61300000000571, "y"=232.0, "position"=-69.61303125000572, "velocity"=-50.000000000005684, "acceleration"=-0.0, "jerk"=-0.0, "heading"=-0.0}, {"dt"=0.005, "x"=69.86300000000574, "y"=232.0, "position"=-69.86303125000575, "velocity"=-50.000000000005684, "acceleration"=-0.0, "jerk"=-0.0, "heading"=-0.0}, {"dt"=0.005, "x"=70.11300000000577, "y"=232.0, "position"=-70.11303125000578, "velocity"=-50.000000000005684, "acceleration"=-0.0, "jerk"=-0.0, "heading"=-0.0}, {"dt"=0.005, "x"=70.3630000000058, "y"=232.0, "position"=-70.3630312500058, "velocity"=-50.000000000005684, "acceleration"=-0.0, "jerk"=-0.0, "heading"=-0.0}, {"dt"=0.005, "x"=70.61300000000583, "y"=232.0, "position"=-70.61303125000583, "velocity"=-50.000000000005684, "acceleration"=-0.0, "jerk"=-0.0, "heading"=-0.0}, {"dt"=0.005, "x"=70.86300000000584, "y"=232.0, "position"=-70.86303125000585, "velocity"=-50.00000000000284, "acceleration"=5.684341886080801e-10, "jerk"=1.1368683772161603e-07, "heading"=-0.0}, {"dt"=0.005, "x"=71.11300000000587, "y"=232.0, "position"=-71.11303125000587, "velocity"=-50.000000000005684, "acceleration"=-5.684341886080801e-10, "jerk"=-2.2737367544323206e-07, "heading"=-0.0}, {"dt"=0.005, "x"=71.36300000000591, "y"=232.0, "position"=-71.36303125000592, "velocity"=-50.00000000000853, "acceleration"=-5.684341886080801e-10, "jerk"=-0.0, "heading"=-0.0}, {"dt"=0.005, "x"=71.61300000000594, "y"=232.0, "position"=-71.61303125000595, "velocity"=-50.000000000005684, "acceleration"=5.684341886080801e-10, "jerk"=2.2737367544323206e-07, "heading"=-0.0}, {"dt"=0.005, "x"=71.86300000000597, "y"=232.0, "position"=-71.86303125000597, "velocity"=-50.000000000005684, "acceleration"=-0.0, "jerk"=-1.1368683772161603e-07, "heading"=-0.0}, {"dt"=0.005, "x"=72.11300000000598, "y"=232.0, "position"=-72.11303125000599, "velocity"=-50.00000000000284, "acceleration"=5.684341886080801e-10, "jerk"=1.1368683772161603e-07, "heading"=-0.0}, {"dt"=0.005, "x"=72.36300000000601, "y"=232.0, "position"=-72.36303125000602, "velocity"=-50.000000000005684, "acceleration"=-5.684341886080801e-10, "jerk"=-2.2737367544323206e-07, "heading"=-0.0}, {"dt"=0.005, "x"=72.61300000000604, "y"=232.0, "position"=-72.61303125000605, "velocity"=-50.000000000005684, "acceleration"=-0.0, "jerk"=1.1368683772161603e-07, "heading"=-0.0}, {"dt"=0.005, "x"=72.86300000000607, "y"=232.0, "position"=-72.86303125000607, "velocity"=-50.000000000005684, "acceleration"=-0.0, "jerk"=-0.0, "heading"=-0.0}, {"dt"=0.005, "x"=73.1130000000061, "y"=232.0, "position"=-73.1130312500061, "velocity"=-50.000000000005684, "acceleration"=-0.0, "jerk"=-0.0, "heading"=-0.0}, {"dt"=0.005, "x"=73.36300000000612, "y"=232.0, "position"=-73.36303125000613, "velocity"=-50.000000000005684, "acceleration"=-0.0, "jerk"=-0.0, "heading"=-0.0}, {"dt"=0.005, "x"=73.61300000000615, "y"=232.0, "position"=-73.61303125000616, "velocity"=-50.000000000005684, "acceleration"=-0.0, "jerk"=-0.0, "heading"=-0.0}, {"dt"=0.005, "x"=73.86300000000618, "y"=232.0, "position"=-73.86303125000619, "velocity"=-50.000000000005684, "acceleration"=-0.0, "jerk"=-0.0, "heading"=-0.0}, {"dt"=0.005, "x"=74.11300000000621, "y"=232.0, "position"=-74.11303125000622, "velocity"=-50.000000000005684, "acceleration"=-0.0, "jerk"=-0.0, "heading"=-0.0}, {"dt"=0.005, "x"=74.36300000000624, "y"=232.0, "position"=-74.36303125000624, "velocity"=-50.000000000005684, "acceleration"=-0.0, "jerk"=-0.0, "heading"=-0.0}, {"dt"=0.005, "x"=74.61300000000625, "y"=232.0, "position"=-74.61303125000626, "velocity"=-50.00000000000284, "acceleration"=5.684341886080801e-10, "jerk"=1.1368683772161603e-07, "heading"=-0.0}, {"dt"=0.005, "x"=74.86300000000628, "y"=232.0, "position"=-74.86303125000629, "velocity"=-50.000000000005684, "acceleration"=-5.684341886080801e-10, "jerk"=-2.2737367544323206e-07, "heading"=-0.0}, {"dt"=0.005, "x"=75.11300000000632, "y"=232.0, "position"=-75.11303125000633, "velocity"=-50.00000000000853, "acceleration"=-5.684341886080801e-10, "jerk"=-0.0, "heading"=-0.0}, {"dt"=0.005, "x"=75.36300000000635, "y"=232.0, "position"=-75.36303125000636, "velocity"=-50.000000000005684, "acceleration"=5.684341886080801e-10, "jerk"=2.2737367544323206e-07, "heading"=-0.0}, {"dt"=0.005, "x"=75.61300000000638, "y"=232.0, "position"=-75.61303125000639, "velocity"=-50.000000000005684, "acceleration"=-0.0, "jerk"=-1.1368683772161603e-07, "heading"=-0.0}, {"dt"=0.005, "x"=75.8630000000064, "y"=232.0, "position"=-75.8630312500064, "velocity"=-50.00000000000284, "acceleration"=5.684341886080801e-10, "jerk"=1.1368683772161603e-07, "heading"=-0.0}, {"dt"=0.005, "x"=76.11300000000642, "y"=232.0, "position"=-76.11303125000643, "velocity"=-50.000000000005684, "acceleration"=-5.684341886080801e-10, "jerk"=-2.2737367544323206e-07, "heading"=-0.0}, {"dt"=0.005, "x"=76.36300000000645, "y"=232.0, "position"=-76.36303125000646, "velocity"=-50.000000000005684, "acceleration"=-0.0, "jerk"=1.1368683772161603e-07, "heading"=-0.0}, {"dt"=0.005, "x"=76.61300000000648, "y"=232.0, "position"=-76.61303125000649, "velocity"=-50.000000000005684, "acceleration"=-0.0, "jerk"=-0.0, "heading"=-0.0}, {"dt"=0.005, "x"=76.86300000000651, "y"=232.0, "position"=-76.86303125000651, "velocity"=-50.000000000005684, "acceleration"=-0.0, "jerk"=-0.0, "heading"=-0.0}, {"dt"=0.005, "x"=77.11300000000654, "y"=232.0, "position"=-77.11303125000654, "velocity"=-50.000000000005684, "acceleration"=-0.0, "jerk"=-0.0, "heading"=-0.0}, {"dt"=0.005, "x"=77.36300000000656, "y"=232.0, "position"=-77.36303125000657, "velocity"=-50.000000000005684, "acceleration"=-0.0, "jerk"=-0.0, "heading"=-0.0}, {"dt"=0.005, "x"=77.6130000000066, "y"=232.0, "position"=-77.6130312500066, "velocity"=-50.000000000005684, "acceleration"=-0.0, "jerk"=-0.0, "heading"=-0.0}, {"dt"=0.005, "x"=77.86300000000662, "y"=232.0, "position"=-77.86303125000663, "velocity"=-50.000000000005684, "acceleration"=-0.0, "jerk"=-0.0, "heading"=-0.0}, {"dt"=0.005, "x"=78.11300000000665, "y"=232.0, "position"=-78.11303125000666, "velocity"=-50.000000000005684, "acceleration"=-0.0, "jerk"=-0.0, "heading"=-0.0}, {"dt"=0.005, "x"=78.36300000000666, "y"=232.0, "position"=-78.36303125000667, "velocity"=-50.00000000000284, "acceleration"=5.684341886080801e-10, "jerk"=1.1368683772161603e-07, "heading"=-0.0}, {"dt"=0.005, "x"=78.61300000000669, "y"=232.0, "position"=-78.6130312500067, "velocity"=-50.000000000005684, "acceleration"=-5.684341886080801e-10, "jerk"=-2.2737367544323206e-07, "heading"=-0.0}, {"dt"=0.005, "x"=78.86300000000674, "y"=232.0, "position"=-78.86303125000674, "velocity"=-50.00000000000853, "acceleration"=-5.684341886080801e-10, "jerk"=-0.0, "heading"=-0.0}, {"dt"=0.005, "x"=79.11300000000676, "y"=232.0, "position"=-79.11303125000677, "velocity"=-50.000000000005684, "acceleration"=5.684341886080801e-10, "jerk"=2.2737367544323206e-07, "heading"=-0.0}, {"dt"=0.005, "x"=79.36300000000679, "y"=232.0, "position"=-79.3630312500068, "velocity"=-50.000000000005684, "acceleration"=-0.0, "jerk"=-1.1368683772161603e-07, "heading"=-0.0}, {"dt"=0.005, "x"=79.6130000000068, "y"=232.0, "position"=-79.61303125000681, "velocity"=-50.00000000000284, "acceleration"=5.684341886080801e-10, "jerk"=1.1368683772161603e-07, "heading"=-0.0}, {"dt"=0.005, "x"=79.86300000000683, "y"=232.0, "position"=-79.86303125000684, "velocity"=-50.000000000005684, "acceleration"=-5.684341886080801e-10, "jerk"=-2.2737367544323206e-07, "heading"=-0.0}, {"dt"=0.005, "x"=80.11300000000686, "y"=232.0, "position"=-80.11303125000687, "velocity"=-50.000000000005684, "acceleration"=-0.0, "jerk"=1.1368683772161603e-07, "heading"=-0.0}, {"dt"=0.005, "x"=80.36300000000689, "y"=232.0, "position"=-80.3630312500069, "velocity"=-50.000000000005684, "acceleration"=-0.0, "jerk"=-0.0, "heading"=-0.0}, {"dt"=0.005, "x"=80.61300000000692, "y"=232.0, "position"=-80.61303125000693, "velocity"=-50.000000000005684, "acceleration"=-0.0, "jerk"=-0.0, "heading"=-0.0}, {"dt"=0.005, "x"=80.86300000000695, "y"=232.0, "position"=-80.86303125000696, "velocity"=-50.000000000005684, "acceleration"=-0.0, "jerk"=-0.0, "heading"=-0.0}, {"dt"=0.005, "x"=81.11300000000698, "y"=232.0, "position"=-81.11303125000698, "velocity"=-50.000000000005684, "acceleration"=-0.0, "jerk"=-0.0, "heading"=-0.0}, {"dt"=0.005, "x"=81.363000000007, "y"=232.0, "position"=-81.36303125000701, "velocity"=-50.000000000005684, "acceleration"=-0.0, "jerk"=-0.0, "heading"=-0.0}, {"dt"=0.005, "x"=81.61300000000703, "y"=232.0, "position"=-81.61303125000704, "velocity"=-50.000000000005684, "acceleration"=-0.0, "jerk"=-0.0, "heading"=-0.0}, {"dt"=0.005, "x"=81.86300000000706, "y"=232.0, "position"=-81.86303125000707, "velocity"=-50.000000000005684, "acceleration"=-0.0, "jerk"=-0.0, "heading"=-0.0}, {"dt"=0.005, "x"=82.11300000000708, "y"=232.0, "position"=-82.11303125000708, "velocity"=-50.00000000000284, "acceleration"=5.684341886080801e-10, "jerk"=1.1368683772161603e-07, "heading"=-0.0}, {"dt"=0.005, "x"=82.3630000000071, "y"=232.0, "position"=-82.36303125000711, "velocity"=-50.000000000005684, "acceleration"=-5.684341886080801e-10, "jerk"=-2.2737367544323206e-07, "heading"=-0.0}, {"dt"=0.005, "x"=82.61300000000715, "y"=232.0, "position"=-82.61303125000715, "velocity"=-50.00000000000853, "acceleration"=-5.684341886080801e-10, "jerk"=-0.0, "heading"=-0.0}, {"dt"=0.005, "x"=82.86300000000718, "y"=232.0, "position"=-82.86303125000718, "velocity"=-50.000000000005684, "acceleration"=5.684341886080801e-10, "jerk"=2.2737367544323206e-07, "heading"=-0.0}, {"dt"=0.005, "x"=83.1130000000072, "y"=232.0, "position"=-83.11303125000721, "velocity"=-50.000000000005684, "acceleration"=-0.0, "jerk"=-1.1368683772161603e-07, "heading"=-0.0}, {"dt"=0.005, "x"=83.36300000000722, "y"=232.0, "position"=-83.36303125000723, "velocity"=-50.00000000000284, "acceleration"=5.684341886080801e-10, "jerk"=1.1368683772161603e-07, "heading"=-0.0}, {"dt"=0.005, "x"=83.61300000000725, "y"=232.0, "position"=-83.61303125000725, "velocity"=-50.000000000005684, "acceleration"=-5.684341886080801e-10, "jerk"=-2.2737367544323206e-07, "heading"=-0.0}, {"dt"=0.005, "x"=83.86300000000728, "y"=232.0, "position"=-83.86303125000728, "velocity"=-50.000000000005684, "acceleration"=-0.0, "jerk"=1.1368683772161603e-07, "heading"=-0.0}, {"dt"=0.005, "x"=84.1130000000073, "y"=232.0, "position"=-84.11303125000731, "velocity"=-50.000000000005684, "acceleration"=-0.0, "jerk"=-0.0, "heading"=-0.0}, {"dt"=0.005, "x"=84.36300000000733, "y"=232.0, "position"=-84.36303125000734, "velocity"=-50.000000000005684, "acceleration"=-0.0, "jerk"=-0.0, "heading"=-0.0}, {"dt"=0.005, "x"=84.61300000000736, "y"=232.0, "position"=-84.61303125000737, "velocity"=-50.000000000005684, "acceleration"=-0.0, "jerk"=-0.0, "heading"=-0.0}, {"dt"=0.005, "x"=84.86300000000739, "y"=232.0, "position"=-84.8630312500074, "velocity"=-50.000000000005684, "acceleration"=-0.0, "jerk"=-0.0, "heading"=-0.0}, {"dt"=0.005, "x"=85.11300000000742, "y"=232.0, "position"=-85.11303125000742, "velocity"=-50.000000000005684, "acceleration"=-0.0, "jerk"=-0.0, "heading"=-0.0}, {"dt"=0.005, "x"=85.36300000000745, "y"=232.0, "position"=-85.36303125000745, "velocity"=-50.000000000005684, "acceleration"=-0.0, "jerk"=-0.0, "heading"=-0.0}, {"dt"=0.005, "x"=85.61300000000747, "y"=232.0, "position"=-85.61303125000748, "velocity"=-50.000000000005684, "acceleration"=-0.0, "jerk"=-0.0, "heading"=-0.0}, {"dt"=0.005, "x"=85.8630000000075, "y"=232.0, "position"=-85.86303125000751, "velocity"=-50.000000000005684, "acceleration"=-0.0, "jerk"=-0.0, "heading"=-0.0}, {"dt"=0.005, "x"=86.11300000000752, "y"=232.0, "position"=-86.11303125000752, "velocity"=-50.00000000000284, "acceleration"=5.684341886080801e-10, "jerk"=1.1368683772161603e-07, "heading"=-0.0}, {"dt"=0.005, "x"=86.36300000000756, "y"=232.0, "position"=-86.36303125000757, "velocity"=-50.00000000000853, "acceleration"=-1.1368683772161603e-09, "jerk"=-3.410605131648481e-07, "heading"=-0.0}, {"dt"=0.005, "x"=86.61300000000759, "y"=232.0, "position"=-86.6130312500076, "velocity"=-50.000000000005684, "acceleration"=5.684341886080801e-10, "jerk"=3.410605131648481e-07, "heading"=-0.0}, {"dt"=0.005, "x"=86.86300000000762, "y"=232.0, "position"=-86.86303125000762, "velocity"=-50.000000000005684, "acceleration"=-0.0, "jerk"=-1.1368683772161603e-07, "heading"=-0.0}, {"dt"=0.005, "x"=87.11300000000764, "y"=232.0, "position"=-87.11303125000765, "velocity"=-50.000000000005684, "acceleration"=-0.0, "jerk"=-0.0, "heading"=-0.0}, {"dt"=0.005, "x"=87.36300000000766, "y"=232.0, "position"=-87.36303125000767, "velocity"=-50.00000000000284, "acceleration"=5.684341886080801e-10, "jerk"=1.1368683772161603e-07, "heading"=-0.0}, {"dt"=0.005, "x"=87.61300000000769, "y"=232.0, "position"=-87.6130312500077, "velocity"=-50.000000000005684, "acceleration"=-5.684341886080801e-10, "jerk"=-2.2737367544323206e-07, "heading"=-0.0}, {"dt"=0.005, "x"=87.86300000000772, "y"=232.0, "position"=-87.86303125000772, "velocity"=-50.000000000005684, "acceleration"=-0.0, "jerk"=1.1368683772161603e-07, "heading"=-0.0}, {"dt"=0.005, "x"=88.11300000000774, "y"=232.0, "position"=-88.11303125000775, "velocity"=-50.000000000005684, "acceleration"=-0.0, "jerk"=-0.0, "heading"=-0.0}, {"dt"=0.005, "x"=88.36300000000779, "y"=232.0, "position"=-88.3630312500078, "velocity"=-50.00000000000853, "acceleration"=-5.684341886080801e-10, "jerk"=-1.1368683772161603e-07, "heading"=-0.0}, {"dt"=0.005, "x"=88.6130000000078, "y"=232.0, "position"=-88.61303125000781, "velocity"=-50.00000000000284, "acceleration"=1.1368683772161603e-09, "jerk"=3.410605131648481e-07, "heading"=-0.0}, {"dt"=0.005, "x"=88.86300000000783, "y"=232.0, "position"=-88.86303125000784, "velocity"=-50.000000000005684, "acceleration"=-5.684341886080801e-10, "jerk"=-3.410605131648481e-07, "heading"=-0.0}, {"dt"=0.005, "x"=89.11300000000786, "y"=232.0, "position"=-89.11303125000786, "velocity"=-50.000000000005684, "acceleration"=-0.0, "jerk"=1.1368683772161603e-07, "heading"=-0.0}, {"dt"=0.005, "x"=89.36300000000789, "y"=232.0, "position"=-89.3630312500079, "velocity"=-50.000000000005684, "acceleration"=-0.0, "jerk"=-0.0, "heading"=-0.0}, {"dt"=0.005, "x"=89.61300000000791, "y"=232.0, "position"=-89.61303125000792, "velocity"=-50.000000000005684, "acceleration"=-0.0, "jerk"=-0.0, "heading"=-0.0}, {"dt"=0.005, "x"=89.86300000000793, "y"=232.0, "position"=-89.86303125000794, "velocity"=-50.00000000000284, "acceleration"=5.684341886080801e-10, "jerk"=1.1368683772161603e-07, "heading"=-0.0}, {"dt"=0.005, "x"=90.11300000000797, "y"=232.0, "position"=-90.11303125000798, "velocity"=-50.00000000000853, "acceleration"=-1.1368683772161603e-09, "jerk"=-3.410605131648481e-07, "heading"=-0.0}, {"dt"=0.005, "x"=90.363000000008, "y"=232.0, "position"=-90.363031250008, "velocity"=-50.000000000005684, "acceleration"=5.684341886080801e-10, "jerk"=3.410605131648481e-07, "heading"=-0.0}, {"dt"=0.005, "x"=90.61300000000803, "y"=232.0, "position"=-90.61303125000804, "velocity"=-50.000000000005684, "acceleration"=-0.0, "jerk"=-1.1368683772161603e-07, "heading"=-0.0}, {"dt"=0.005, "x"=90.86300000000806, "y"=232.0, "position"=-90.86303125000806, "velocity"=-50.000000000005684, "acceleration"=-0.0, "jerk"=-0.0, "heading"=-0.0}, {"dt"=0.005, "x"=91.11300000000807, "y"=232.0, "position"=-91.11303125000808, "velocity"=-50.00000000000284, "acceleration"=5.684341886080801e-10, "jerk"=1.1368683772161603e-07, "heading"=-0.0}, {"dt"=0.005, "x"=91.3630000000081, "y"=232.0, "position"=-91.3630312500081, "velocity"=-50.000000000005684, "acceleration"=-5.684341886080801e-10, "jerk"=-2.2737367544323206e-07, "heading"=-0.0}, {"dt"=0.005, "x"=91.61300000000813, "y"=232.0, "position"=-91.61303125000813, "velocity"=-50.000000000005684, "acceleration"=-0.0, "jerk"=1.1368683772161603e-07, "heading"=-0.0}, {"dt"=0.005, "x"=91.86300000000816, "y"=232.0, "position"=-91.86303125000816, "velocity"=-50.000000000005684, "acceleration"=-0.0, "jerk"=-0.0, "heading"=-0.0}, {"dt"=0.005, "x"=92.1130000000082, "y"=232.0, "position"=-92.1130312500082, "velocity"=-50.00000000000853, "acceleration"=-5.684341886080801e-10, "jerk"=-1.1368683772161603e-07, "heading"=-0.0}, {"dt"=0.005, "x"=92.36300000000821, "y"=232.0, "position"=-92.36303125000822, "velocity"=-50.00000000000284, "acceleration"=1.1368683772161603e-09, "jerk"=3.410605131648481e-07, "heading"=-0.0}, {"dt"=0.005, "x"=92.61300000000824, "y"=232.0, "position"=-92.61303125000825, "velocity"=-50.000000000005684, "acceleration"=-5.684341886080801e-10, "jerk"=-3.410605131648481e-07, "heading"=-0.0}, {"dt"=0.005, "x"=92.86297025000827, "y"=232.0, "position"=-92.86300150000828, "velocity"=-49.994050000006496, "acceleration"=1.1899999998377098, "jerk"=238.0000000812288, "heading"=-0.0}, {"dt"=0.005, "x"=93.1128497500083, "y"=232.0, "position"=-93.1128810000083, "velocity"=-49.975900000004, "acceleration"=3.6300000004985122, "jerk"=488.0000001321605, "heading"=-0.0}, {"dt"=0.005, "x"=93.36257600000832, "y"=232.0, "position"=-93.36260725000832, "velocity"=-49.94525000000465, "acceleration"=6.129999999870961, "jerk"=499.99999987448973, "heading"=-0.0}, {"dt"=0.005, "x"=93.61208650000833, "y"=232.0, "position"=-93.61211775000834, "velocity"=-49.90210000000275, "acceleration"=8.630000000380278, "jerk"=500.0000001018634, "heading"=-0.0}, {"dt"=0.005, "x"=93.86131875000834, "y"=232.0, "position"=-93.86135000000834, "velocity"=-49.84645000000114, "acceleration"=11.13000000032116, "jerk"=499.99999998817657, "heading"=-0.0}, {"dt"=0.005, "x"=94.11021025000836, "y"=232.0, "position"=-94.11024150000837, "velocity"=-49.778300000005515, "acceleration"=13.629999999125175, "jerk"=499.9999997608029, "heading"=-0.0}, {"dt"=0.005, "x"=94.35869850000837, "y"=232.0, "position"=-94.35872975000838, "velocity"=-49.69765000000166, "acceleration"=16.13000000077136, "jerk"=500.0000003292371, "heading"=-0.0}, {"dt"=0.005, "x"=94.60672100000838, "y"=232.0, "position"=-94.60675225000838, "velocity"=-49.60450000000094, "acceleration"=18.63000000014381, "jerk"=499.99999987448973, "heading"=-0.0}, {"dt"=0.005, "x"=94.85421525000838, "y"=232.0, "position"=-94.85424650000839, "velocity"=-49.498850000000516, "acceleration"=21.130000000084692, "jerk"=499.99999998817657, "heading"=-0.0}, {"dt"=0.005, "x"=95.10111875000837, "y"=232.0, "position"=-95.10115000000837, "velocity"=-49.380699999997546, "acceleration"=23.63000000059401, "jerk"=500.0000001018634, "heading"=-0.0}, {"dt"=0.005, "x"=95.34736900000837, "y"=232.0, "position"=-95.34740025000838, "velocity"=-49.250050000000556, "acceleration"=26.129999999398024, "jerk"=499.9999997608029, "heading"=-0.0}, {"dt"=0.005, "x"=95.59290350000836, "y"=232.0, "position"=-95.59293475000837, "velocity"=-49.10689999999818, "acceleration"=28.630000000475775, "jerk"=500.00000021555024, "heading"=-0.0}, {"dt"=0.005, "x"=95.83765975000834, "y"=232.0, "position"=-95.83769100000835, "velocity"=-48.951249999996094, "acceleration"=31.130000000416658, "jerk"=499.99999998817657, "heading"=-0.0}, {"dt"=0.005, "x"=96.08157525000834, "y"=232.0, "position"=-96.08160650000835, "velocity"=-48.78309999999999, "acceleration"=33.62999999922067, "jerk"=499.9999997608029, "heading"=-0.0}, {"dt"=0.005, "x"=96.32458750000833, "y"=232.0, "position"=-96.32461875000834, "velocity"=-48.6024499999985, "acceleration"=36.13000000029842, "jerk"=500.00000021555024, "heading"=-0.0}, {"dt"=0.005, "x"=96.56663400000832, "y"=232.0, "position"=-96.56666525000833, "velocity"=-48.4092999999973, "acceleration"=38.630000000239306, "jerk"=499.99999998817657, "heading"=-0.0}, {"dt"=0.005, "x"=96.80765225000829, "y"=232.0, "position"=-96.8076835000083, "velocity"=-48.20364999999356, "acceleration"=41.13000000074862, "jerk"=500.0000001018634, "heading"=-0.0}, {"dt"=0.005, "x"=97.04757975000827, "y"=232.0, "position"=-97.04761100000827, "velocity"=-47.985499999995795, "acceleration"=43.62999999955264, "jerk"=499.9999997608029, "heading"=-0.0}, {"dt"=0.005, "x"=97.28635400000825, "y"=232.0, "position"=-97.28638525000825, "velocity"=-47.754849999995486, "acceleration"=46.130000000061955, "jerk"=500.0000001018634, "heading"=-0.0}, {"dt"=0.005, "x"=97.52391250000822, "y"=232.0, "position"=-97.52394375000823, "velocity"=-47.51169999999547, "acceleration"=48.63000000000284, "jerk"=499.99999998817657, "heading"=-0.0}, {"dt"=0.005, "x"=97.76022250000818, "y"=232.0, "position"=-97.76025375000819, "velocity"=-47.2619999999921, "acceleration"=49.940000000674445, "jerk"=262.00000013432145, "heading"=-0.0}, {"dt"=0.005, "x"=97.99528250000816, "y"=232.0, "position"=-97.99531375000817, "velocity"=-47.01199999999517, "acceleration"=49.99999999938609, "jerk"=11.999999742329237, "heading"=-0.0}, {"dt"=0.005, "x"=98.22909250000814, "y"=232.0, "position"=-98.22912375000814, "velocity"=-46.761999999995396, "acceleration"=49.999999999954525, "jerk"=1.1368683772161603e-07, "heading"=-0.0}, {"dt"=0.005, "x"=98.46165250000813, "y"=232.0, "position"=-98.46168375000813, "velocity"=-46.511999999998466, "acceleration"=49.99999999938609, "jerk"=-1.1368683772161603e-07, "heading"=-0.0}, {"dt"=0.005, "x"=98.6929625000081, "y"=232.0, "position"=-98.6929937500081, "velocity"=-46.26199999999301, "acceleration"=50.000000001091394, "jerk"=3.410605131648481e-07, "heading"=-0.0}, {"dt"=0.005, "x"=98.92302250000807, "y"=232.0, "position"=-98.92305375000808, "velocity"=-46.01199999999608, "acceleration"=49.99999999938609, "jerk"=-3.410605131648481e-07, "heading"=-0.0}, {"dt"=0.005, "x"=99.15183250000803, "y"=232.0, "position"=-99.15186375000803, "velocity"=-45.76199999999062, "acceleration"=50.000000001091394, "jerk"=3.410605131648481e-07, "heading"=-0.0}, {"dt"=0.005, "x"=99.37939250000798, "y"=232.0, "position"=-99.37942375000799, "velocity"=-45.51199999999085, "acceleration"=49.999999999954525, "jerk"=-2.2737367544323206e-07, "heading"=-0.0}, {"dt"=0.005, "x"=99.60570250000795, "y"=232.0, "position"=-99.60573375000796, "velocity"=-45.26199999999392, "acceleration"=49.99999999938609, "jerk"=-1.1368683772161603e-07, "heading"=-0.0}, {"dt"=0.005, "x"=99.83076250000792, "y"=232.0, "position"=-99.83079375000793, "velocity"=-45.011999999994146, "acceleration"=49.999999999954525, "jerk"=1.1368683772161603e-07, "heading"=-0.0}, {"dt"=0.005, "x"=100.0545725000079, "y"=232.0, "position"=-100.0546037500079, "velocity"=-44.76199999999437, "acceleration"=49.999999999954525, "jerk"=-0.0, "heading"=-0.0}, {"dt"=0.005, "x"=100.27713250000785, "y"=232.0, "position"=-100.27716375000786, "velocity"=-44.51199999999176, "acceleration"=50.00000000052296, "jerk"=1.1368683772161603e-07, "heading"=-0.0}, {"dt"=0.005, "x"=100.49844250000783, "y"=232.0, "position"=-100.49847375000783, "velocity"=-44.26199999999483, "acceleration"=49.99999999938609, "jerk"=-2.2737367544323206e-07, "heading"=-0.0}, {"dt"=0.005, "x"=100.71850250000782, "y"=232.0, "position"=-100.71853375000782, "velocity"=-44.0119999999979, "acceleration"=49.99999999938609, "jerk"=-0.0, "heading"=-0.0}, {"dt"=0.005, "x"=100.93731250000776, "y"=232.0, "position"=-100.93734375000777, "velocity"=-43.7619999999896, "acceleration"=50.00000000165983, "jerk"=4.547473508864641e-07, "heading"=-0.0}, {"dt"=0.005, "x"=101.15487250000774, "y"=232.0, "position"=-101.15490375000775, "velocity"=-43.51199999999551, "acceleration"=49.99999999881766, "jerk"=-5.684341886080801e-07, "heading"=-0.0}, {"dt"=0.005, "x"=101.3711825000077, "y"=232.0, "position"=-101.37121375000771, "velocity"=-43.261999999992895, "acceleration"=50.00000000052296, "jerk"=3.410605131648481e-07, "heading"=-0.0}, {"dt"=0.005, "x"=101.58624250000767, "y"=232.0, "position"=-101.58627375000768, "velocity"=-43.01199999999312, "acceleration"=49.999999999954525, "jerk"=-1.1368683772161603e-07, "heading"=-0.0}, {"dt"=0.005, "x"=101.80005250000765, "y"=232.0, "position"=-101.80008375000766, "velocity"=-42.76199999999619, "acceleration"=49.99999999938609, "jerk"=-1.1368683772161603e-07, "heading"=-0.0}, {"dt"=0.005, "x"=102.0126125000076, "y"=232.0, "position"=-102.01264375000761, "velocity"=-42.511999999990735, "acceleration"=50.000000001091394, "jerk"=3.410605131648481e-07, "heading"=-0.0}, {"dt"=0.005, "x"=102.22392250000756, "y"=232.0, "position"=-102.22395375000757, "velocity"=-42.26199999999096, "acceleration"=49.999999999954525, "jerk"=-2.2737367544323206e-07, "heading"=-0.0}, {"dt"=0.005, "x"=102.43398250000753, "y"=232.0, "position"=-102.43401375000754, "velocity"=-42.01199999999403, "acceleration"=49.99999999938609, "jerk"=-1.1368683772161603e-07, "heading"=-0.0}, {"dt"=0.005, "x"=102.6427925000075, "y"=232.0, "position"=-102.64282375000751, "velocity"=-41.76199999999426, "acceleration"=49.999999999954525, "jerk"=1.1368683772161603e-07, "heading"=-0.0}, {"dt"=0.005, "x"=102.85035250000746, "y"=232.0, "position"=-102.85038375000747, "velocity"=-41.511999999991644, "acceleration"=50.00000000052296, "jerk"=1.1368683772161603e-07, "heading"=-0.0}, {"dt"=0.005, "x"=103.05666250000743, "y"=232.0, "position"=-103.05669375000744, "velocity"=-41.261999999994714, "acceleration"=49.99999999938609, "jerk"=-2.2737367544323206e-07, "heading"=-0.0}, {"dt"=0.005, "x"=103.26172250000741, "y"=232.0, "position"=-103.26175375000741, "velocity"=-41.01199999999494, "acceleration"=49.999999999954525, "jerk"=1.1368683772161603e-07, "heading"=-0.0}, {"dt"=0.005, "x"=103.46553250000737, "y"=232.0, "position"=-103.46556375000738, "velocity"=-40.76199999999233, "acceleration"=50.00000000052296, "jerk"=1.1368683772161603e-07, "heading"=-0.0}, {"dt"=0.005, "x"=103.66809250000735, "y"=232.0, "position"=-103.66812375000735, "velocity"=-40.511999999995396, "acceleration"=49.99999999938609, "jerk"=-2.2737367544323206e-07, "heading"=-0.0}, {"dt"=0.005, "x"=103.86940250000733, "y"=232.0, "position"=-103.86943375000733, "velocity"=-40.26199999999562, "acceleration"=49.999999999954525, "jerk"=1.1368683772161603e-07, "heading"=-0.0}, {"dt"=0.005, "x"=104.06946250000728, "y"=232.0, "position"=-104.06949375000728, "velocity"=-40.01199999999017, "acceleration"=50.000000001091394, "jerk"=2.2737367544323206e-07, "heading"=-0.0}, {"dt"=0.005, "x"=104.26827250000726, "y"=232.0, "position"=-104.26830375000726, "velocity"=-39.76199999999608, "acceleration"=49.99999999881766, "jerk"=-4.547473508864641e-07, "heading"=-0.0}, {"dt"=0.005, "x"=104.46583250000721, "y"=232.0, "position"=-104.46586375000722, "velocity"=-39.51199999999062, "acceleration"=50.000000001091394, "jerk"=4.547473508864641e-07, "heading"=-0.0}, {"dt"=0.005, "x"=104.66214250000716, "y"=232.0, "position"=-104.66217375000717, "velocity"=-39.26199999999085, "acceleration"=49.999999999954525, "jerk"=-2.2737367544323206e-07, "heading"=-0.0}, {"dt"=0.005, "x"=104.85720250000713, "y"=232.0, "position"=-104.85723375000714, "velocity"=-39.01199999999392, "acceleration"=49.99999999938609, "jerk"=-1.1368683772161603e-07, "heading"=-0.0}, {"dt"=0.005, "x"=105.05101250000709, "y"=232.0, "position"=-105.0510437500071, "velocity"=-38.7619999999913, "acceleration"=50.00000000052296, "jerk"=2.2737367544323206e-07, "heading"=-0.0}, {"dt"=0.005, "x"=105.24357250000706, "y"=232.0, "position"=-105.24360375000707, "velocity"=-38.51199999999437, "acceleration"=49.99999999938609, "jerk"=-2.2737367544323206e-07, "heading"=-0.0}, {"dt"=0.005, "x"=105.43488250000703, "y"=232.0, "position"=-105.43491375000704, "velocity"=-38.2619999999946, "acceleration"=49.999999999954525, "jerk"=1.1368683772161603e-07, "heading"=-0.0}, {"dt"=0.005, "x"=105.624942500007, "y"=232.0, "position"=-105.624973750007, "velocity"=-38.011999999991986, "acceleration"=50.00000000052296, "jerk"=1.1368683772161603e-07, "heading"=-0.0}, {"dt"=0.005, "x"=105.81375250000697, "y"=232.0, "position"=-105.81378375000698, "velocity"=-37.761999999995055, "acceleration"=49.99999999938609, "jerk"=-2.2737367544323206e-07, "heading"=-0.0}, {"dt"=0.005, "x"=106.00131250000693, "y"=232.0, "position"=-106.00134375000694, "velocity"=-37.51199999999244, "acceleration"=50.00000000052296, "jerk"=2.2737367544323206e-07, "heading"=-0.0}, {"dt"=0.005, "x"=106.1876225000069, "y"=232.0, "position"=-106.1876537500069, "velocity"=-37.26199999999267, "acceleration"=49.999999999954525, "jerk"=-1.1368683772161603e-07, "heading"=-0.0}, {"dt"=0.005, "x"=106.37268250000686, "y"=232.0, "position"=-106.37271375000687, "velocity"=-37.011999999992895, "acceleration"=49.999999999954525, "jerk"=-0.0, "heading"=-0.0}, {"dt"=0.005, "x"=106.55649250000683, "y"=232.0, "position"=-106.55652375000683, "velocity"=-36.76199999999312, "acceleration"=49.999999999954525, "jerk"=-0.0, "heading"=-0.0}, {"dt"=0.005, "x"=106.73905250000678, "y"=232.0, "position"=-106.73908375000678, "velocity"=-36.51199999999051, "acceleration"=50.00000000052296, "jerk"=1.1368683772161603e-07, "heading"=-0.0}, {"dt"=0.005, "x"=106.92036250000675, "y"=232.0, "position"=-106.92039375000675, "velocity"=-36.26199999999358, "acceleration"=49.99999999938609, "jerk"=-2.2737367544323206e-07, "heading"=-0.0}, {"dt"=0.005, "x"=107.1004225000067, "y"=232.0, "position"=-107.10045375000671, "velocity"=-36.01199999999096, "acceleration"=50.00000000052296, "jerk"=2.2737367544323206e-07, "heading"=-0.0}, {"dt"=0.005, "x"=107.27923250000667, "y"=232.0, "position"=-107.27926375000668, "velocity"=-35.76199999999403, "acceleration"=49.99999999938609, "jerk"=-2.2737367544323206e-07, "heading"=-0.0}, {"dt"=0.005, "x"=107.45679250000663, "y"=232.0, "position"=-107.45682375000663, "velocity"=-35.51199999999142, "acceleration"=50.00000000052296, "jerk"=2.2737367544323206e-07, "heading"=-0.0}, {"dt"=0.005, "x"=107.6331025000066, "y"=232.0, "position"=-107.6331337500066, "velocity"=-35.26199999999449, "acceleration"=49.99999999938609, "jerk"=-2.2737367544323206e-07, "heading"=-0.0}, {"dt"=0.005, "x"=107.80816250000656, "y"=232.0, "position"=-107.80819375000657, "velocity"=-35.01199999999187, "acceleration"=50.00000000052296, "jerk"=2.2737367544323206e-07, "heading"=-0.0}, {"dt"=0.005, "x"=107.98197250000652, "y"=232.0, "position"=-107.98200375000653, "velocity"=-34.7619999999921, "acceleration"=49.999999999954525, "jerk"=-1.1368683772161603e-07, "heading"=-0.0}, {"dt"=0.005, "x"=108.15453250000648, "y"=232.0, "position"=-108.15456375000649, "velocity"=-34.51199999999233, "acceleration"=49.999999999954525, "jerk"=-0.0, "heading"=-0.0}, {"dt"=0.005, "x"=108.32584250000647, "y"=232.0, "position"=-108.32587375000648, "velocity"=-34.26199999999824, "acceleration"=49.99999999881766, "jerk"=-2.2737367544323206e-07, "heading"=-0.0}, {"dt"=0.005, "x"=108.49590250000642, "y"=232.0, "position"=-108.49593375000643, "velocity"=-34.01199999998994, "acceleration"=50.00000000165983, "jerk"=5.684341886080801e-07, "heading"=-0.0}, {"dt"=0.005, "x"=108.66471250000639, "y"=232.0, "position"=-108.6647437500064, "velocity"=-33.76199999999301, "acceleration"=49.99999999938609, "jerk"=-4.547473508864641e-07, "heading"=-0.0}, {"dt"=0.005, "x"=108.83227250000635, "y"=232.0, "position"=-108.83230375000636, "velocity"=-33.511999999993236, "acceleration"=49.999999999954525, "jerk"=1.1368683772161603e-07, "heading"=-0.0}, {"dt"=0.005, "x"=108.99858250000631, "y"=232.0, "position"=-108.99861375000631, "velocity"=-33.26199999999062, "acceleration"=50.00000000052296, "jerk"=1.1368683772161603e-07, "heading"=-0.0}, {"dt"=0.005, "x"=109.16364250000626, "y"=232.0, "position"=-109.16367375000627, "velocity"=-33.01199999999085, "acceleration"=49.999999999954525, "jerk"=-1.1368683772161603e-07, "heading"=-0.0}, {"dt"=0.005, "x"=109.32745250000623, "y"=232.0, "position"=-109.32748375000624, "velocity"=-32.76199999999392, "acceleration"=49.99999999938609, "jerk"=-1.1368683772161603e-07, "heading"=-0.0}, {"dt"=0.005, "x"=109.49001250000619, "y"=232.0, "position"=-109.4900437500062, "velocity"=-32.5119999999913, "acceleration"=50.00000000052296, "jerk"=2.2737367544323206e-07, "heading"=-0.0}, {"dt"=0.005, "x"=109.65132250000615, "y"=232.0, "position"=-109.65135375000615, "velocity"=-32.26199999999153, "acceleration"=49.999999999954525, "jerk"=-1.1368683772161603e-07, "heading"=-0.0}, {"dt"=0.005, "x"=109.81138250000612, "y"=232.0, "position"=-109.81141375000612, "velocity"=-32.0119999999946, "acceleration"=49.99999999938609, "jerk"=-1.1368683772161603e-07, "heading"=-0.0}, {"dt"=0.005, "x"=109.97019250000606, "y"=232.0, "position"=-109.97022375000607, "velocity"=-31.761999999989143, "acceleration"=50.000000001091394, "jerk"=3.410605131648481e-07, "heading"=-0.0}, {"dt"=0.005, "x"=110.12775250000603, "y"=232.0, "position"=-110.12778375000603, "velocity"=-31.511999999992213, "acceleration"=49.99999999938609, "jerk"=-3.410605131648481e-07, "heading"=-0.0}, {"dt"=0.005, "x"=110.284062500006, "y"=232.0, "position"=-110.28409375000601, "velocity"=-31.261999999995282, "acceleration"=49.99999999938609, "jerk"=-0.0, "heading"=-0.0}, {"dt"=0.005, "x"=110.43912250000598, "y"=232.0, "position"=-110.43915375000599, "velocity"=-31.01199999999551, "acceleration"=49.999999999954525, "jerk"=1.1368683772161603e-07, "heading"=-0.0}, {"dt"=0.005, "x"=110.59293250000593, "y"=232.0, "position"=-110.59296375000594, "velocity"=-30.761999999990053, "acceleration"=50.000000001091394, "jerk"=2.2737367544323206e-07, "heading"=-0.0}, {"dt"=0.005, "x"=110.7454925000059, "y"=232.0, "position"=-110.7455237500059, "velocity"=-30.511999999993122, "acceleration"=49.99999999938609, "jerk"=-3.410605131648481e-07, "heading"=-0.0}, {"dt"=0.005, "x"=110.89680250000585, "y"=232.0, "position"=-110.89683375000585, "velocity"=-30.261999999990508, "acceleration"=50.00000000052296, "jerk"=2.2737367544323206e-07, "heading"=-0.0}, {"dt"=0.005, "x"=111.0468625000058, "y"=232.0, "position"=-111.04689375000581, "velocity"=-30.011999999990735, "acceleration"=49.999999999954525, "jerk"=-1.1368683772161603e-07, "heading"=-0.0}, {"dt"=0.005, "x"=111.19567250000576, "y"=232.0, "position"=-111.19570375000576, "velocity"=-29.761999999990962, "acceleration"=49.999999999954525, "jerk"=-0.0, "heading"=-0.0}, {"dt"=0.005, "x"=111.34323250000571, "y"=232.0, "position"=-111.34326375000572, "velocity"=-29.51199999999119, "acceleration"=49.999999999954525, "jerk"=-0.0, "heading"=-0.0}, {"dt"=0.005, "x"=111.48954250000568, "y"=232.0, "position"=-111.48957375000569, "velocity"=-29.26199999999426, "acceleration"=49.99999999938609, "jerk"=-1.1368683772161603e-07, "heading"=-0.0}, {"dt"=0.005, "x"=111.63460250000564, "y"=232.0, "position"=-111.63463375000565, "velocity"=-29.011999999991644, "acceleration"=50.00000000052296, "jerk"=2.2737367544323206e-07, "heading"=-0.0}, {"dt"=0.005, "x"=111.77841250000559, "y"=232.0, "position"=-111.7784437500056, "velocity"=-28.76199999998903, "acceleration"=50.00000000052296, "jerk"=-0.0, "heading"=-0.0}, {"dt"=0.005, "x"=111.92097250000555, "y"=232.0, "position"=-111.92100375000555, "velocity"=-28.5119999999921, "acceleration"=49.99999999938609, "jerk"=-2.2737367544323206e-07, "heading"=-0.0}, {"dt"=0.005, "x"=112.06228250000552, "y"=232.0, "position"=-112.06231375000553, "velocity"=-28.26199999999517, "acceleration"=49.99999999938609, "jerk"=-0.0, "heading"=-0.0}, {"dt"=0.005, "x"=112.2023425000055, "y"=232.0, "position"=-112.2023737500055, "velocity"=-28.011999999995396, "acceleration"=49.999999999954525, "jerk"=1.1368683772161603e-07, "heading"=-0.0}, {"dt"=0.005, "x"=112.34115250000545, "y"=232.0, "position"=-112.34118375000546, "velocity"=-27.76199999998994, "acceleration"=50.000000001091394, "jerk"=2.2737367544323206e-07, "heading"=-0.0}, {"dt"=0.005, "x"=112.4787125000054, "y"=232.0, "position"=-112.4787437500054, "velocity"=-27.511999999990167, "acceleration"=49.999999999954525, "jerk"=-2.2737367544323206e-07, "heading"=-0.0}, {"dt"=0.005, "x"=112.61502250000535, "y"=232.0, "position"=-112.61505375000536, "velocity"=-27.261999999990394, "acceleration"=49.999999999954525, "jerk"=-0.0, "heading"=-0.0}, {"dt"=0.005, "x"=112.7500825000053, "y"=232.0, "position"=-112.75011375000531, "velocity"=-27.01199999999062, "acceleration"=49.999999999954525, "jerk"=-0.0, "heading"=-0.0}, {"dt"=0.005, "x"=112.88389250000526, "y"=232.0, "position"=-112.88392375000527, "velocity"=-26.76199999999085, "acceleration"=49.999999999954525, "jerk"=-0.0, "heading"=-0.0}, {"dt"=0.005, "x"=113.01645250000522, "y"=232.0, "position"=-113.01648375000522, "velocity"=-26.511999999991076, "acceleration"=49.999999999954525, "jerk"=-0.0, "heading"=-0.0}, {"dt"=0.005, "x"=113.14776250000517, "y"=232.0, "position"=-113.14779375000518, "velocity"=-26.261999999991303, "acceleration"=49.999999999954525, "jerk"=-0.0, "heading"=-0.0}, {"dt"=0.005, "x"=113.27782250000513, "y"=232.0, "position"=-113.27785375000514, "velocity"=-26.01199999999153, "acceleration"=49.999999999954525, "jerk"=-0.0, "heading"=-0.0}, {"dt"=0.005, "x"=113.4066325000051, "y"=232.0, "position"=-113.40666375000511, "velocity"=-25.7619999999946, "acceleration"=49.99999999938609, "jerk"=-1.1368683772161603e-07, "heading"=-0.0}, {"dt"=0.005, "x"=113.53419250000506, "y"=232.0, "position"=-113.53422375000507, "velocity"=-25.511999999991986, "acceleration"=50.00000000052296, "jerk"=2.2737367544323206e-07, "heading"=-0.0}, {"dt"=0.005, "x"=113.66050250000501, "y"=232.0, "position"=-113.66053375000502, "velocity"=-25.26199999998937, "acceleration"=50.00000000052296, "jerk"=-0.0, "heading"=-0.0}, {"dt"=0.005, "x"=113.78556250000497, "y"=232.0, "position"=-113.78559375000498, "velocity"=-25.01199999999244, "acceleration"=49.99999999938609, "jerk"=-2.2737367544323206e-07, "heading"=-0.0}, {"dt"=0.005, "x"=113.90937250000495, "y"=232.0, "position"=-113.90940375000496, "velocity"=-24.76199999999551, "acceleration"=49.99999999938609, "jerk"=-0.0, "heading"=-0.0}, {"dt"=0.005, "x"=114.0319325000049, "y"=232.0, "position"=-114.0319637500049, "velocity"=-24.511999999990053, "acceleration"=50.000000001091394, "jerk"=3.410605131648481e-07, "heading"=-0.0}, {"dt"=0.005, "x"=114.15324250000486, "y"=232.0, "position"=-114.15327375000487, "velocity"=-24.261999999993122, "acceleration"=49.99999999938609, "jerk"=-3.410605131648481e-07, "heading"=-0.0}, {"dt"=0.005, "x"=114.2733025000048, "y"=232.0, "position"=-114.27333375000481, "velocity"=-24.011999999987665, "acceleration"=50.000000001091394, "jerk"=3.410605131648481e-07, "heading"=-0.0}, {"dt"=0.005, "x"=114.39211250000476, "y"=232.0, "position"=-114.39214375000476, "velocity"=-23.761999999990735, "acceleration"=49.99999999938609, "jerk"=-3.410605131648481e-07, "heading"=-0.0}, {"dt"=0.005, "x"=114.50967250000471, "y"=232.0, "position"=-114.50970375000472, "velocity"=-23.511999999990962, "acceleration"=49.999999999954525, "jerk"=1.1368683772161603e-07, "heading"=-0.0}, {"dt"=0.005, "x"=114.62598250000467, "y"=232.0, "position"=-114.62601375000467, "velocity"=-23.26199999999119, "acceleration"=49.999999999954525, "jerk"=-0.0, "heading"=-0.0}, {"dt"=0.005, "x"=114.74104250000462, "y"=232.0, "position"=-114.74107375000463, "velocity"=-23.011999999991417, "acceleration"=49.999999999954525, "jerk"=-0.0, "heading"=-0.0}, {"dt"=0.005, "x"=114.85485250000458, "y"=232.0, "position"=-114.85488375000459, "velocity"=-22.761999999991644, "acceleration"=49.999999999954525, "jerk"=-0.0, "heading"=-0.0}, {"dt"=0.005, "x"=114.96741250000453, "y"=232.0, "position"=-114.96744375000453, "velocity"=-22.51199999998903, "acceleration"=50.00000000052296, "jerk"=1.1368683772161603e-07, "heading"=-0.0}, {"dt"=0.005, "x"=115.07872250000449, "y"=232.0, "position"=-115.0787537500045, "velocity"=-22.2619999999921, "acceleration"=49.99999999938609, "jerk"=-2.2737367544323206e-07, "heading"=-0.0}, {"dt"=0.005, "x"=115.18878250000444, "y"=232.0, "position"=-115.18881375000444, "velocity"=-22.011999999989484, "acceleration"=50.00000000052296, "jerk"=2.2737367544323206e-07, "heading"=-0.0}, {"dt"=0.005, "x"=115.29759250000441, "y"=232.0, "position"=-115.29762375000442, "velocity"=-21.761999999995396, "acceleration"=49.99999999881766, "jerk"=-3.410605131648481e-07, "heading"=-0.0}, {"dt"=0.005, "x"=115.40515250000438, "y"=232.0, "position"=-115.40518375000438, "velocity"=-21.51199999999278, "acceleration"=50.00000000052296, "jerk"=3.410605131648481e-07, "heading"=-0.0}, {"dt"=0.005, "x"=115.51146250000434, "y"=232.0, "position"=-115.51149375000435, "velocity"=-21.26199999999301, "acceleration"=49.999999999954525, "jerk"=-1.1368683772161603e-07, "heading"=-0.0}, {"dt"=0.005, "x"=115.6165225000043, "y"=232.0, "position"=-115.6165537500043, "velocity"=-21.011999999990394, "acceleration"=50.00000000052296, "jerk"=1.1368683772161603e-07, "heading"=-0.0}, {"dt"=0.005, "x"=115.72033250000425, "y"=232.0, "position"=-115.72036375000425, "velocity"=-20.76199999999062, "acceleration"=49.999999999954525, "jerk"=-1.1368683772161603e-07, "heading"=-0.0}, {"dt"=0.005, "x"=115.82289250000417, "y"=232.0, "position"=-115.82292375000418, "velocity"=-20.511999999985164, "acceleration"=50.000000001091394, "jerk"=2.2737367544323206e-07, "heading"=-0.0}, {"dt"=0.005, "x"=115.92420250000413, "y"=232.0, "position"=-115.92423375000413, "velocity"=-20.261999999991076, "acceleration"=49.99999999881766, "jerk"=-4.547473508864641e-07, "heading"=-0.0}, {"dt"=0.005, "x"=116.02426250000408, "y"=232.0, "position"=-116.02429375000409, "velocity"=-20.011999999991303, "acceleration"=49.999999999954525, "jerk"=2.2737367544323206e-07, "heading"=-0.0}, {"dt"=0.005, "x"=116.12307250000404, "y"=232.0, "position"=-116.12310375000405, "velocity"=-19.76199999999153, "acceleration"=49.999999999954525, "jerk"=-0.0, "heading"=-0.0}, {"dt"=0.005, "x"=116.220632500004, "y"=232.0, "position"=-116.22066375000401, "velocity"=-19.511999999991758, "acceleration"=49.999999999954525, "jerk"=-0.0, "heading"=-0.0}, {"dt"=0.005, "x"=116.31694250000396, "y"=232.0, "position"=-116.31697375000397, "velocity"=-19.261999999991986, "acceleration"=49.999999999954525, "jerk"=-0.0, "heading"=-0.0}, {"dt"=0.005, "x"=116.41200250000391, "y"=232.0, "position"=-116.41203375000391, "velocity"=-19.01199999998937, "acceleration"=50.00000000052296, "jerk"=1.1368683772161603e-07, "heading"=-0.0}, {"dt"=0.005, "x"=116.50581250000387, "y"=232.0, "position"=-116.50584375000388, "velocity"=-18.76199999999244, "acceleration"=49.99999999938609, "jerk"=-2.2737367544323206e-07, "heading"=-0.0}, {"dt"=0.005, "x"=116.59837250000383, "y"=232.0, "position"=-116.59840375000384, "velocity"=-18.511999999992668, "acceleration"=49.999999999954525, "jerk"=1.1368683772161603e-07, "heading"=-0.0}, {"dt"=0.005, "x"=116.6896825000038, "y"=232.0, "position"=-116.6897137500038, "velocity"=-18.261999999992895, "acceleration"=49.999999999954525, "jerk"=-0.0, "heading"=-0.0}, {"dt"=0.005, "x"=116.77974250000374, "y"=232.0, "position"=-116.77977375000374, "velocity"=-18.011999999987438, "acceleration"=50.000000001091394, "jerk"=2.2737367544323206e-07, "heading"=-0.0}, {"dt"=0.005, "x"=116.86855250000369, "y"=232.0, "position"=-116.8685837500037, "velocity"=-17.761999999990508, "acceleration"=49.99999999938609, "jerk"=-3.410605131648481e-07, "heading"=-0.0}, {"dt"=0.005, "x"=116.95611250000364, "y"=232.0, "position"=-116.95614375000365, "velocity"=-17.511999999990735, "acceleration"=49.999999999954525, "jerk"=1.1368683772161603e-07, "heading"=-0.0}, {"dt"=0.005, "x"=117.0424225000036, "y"=232.0, "position"=-117.0424537500036, "velocity"=-17.261999999990962, "acceleration"=49.999999999954525, "jerk"=-0.0, "heading"=-0.0}, {"dt"=0.005, "x"=117.12748250000354, "y"=232.0, "position"=-117.12751375000354, "velocity"=-17.011999999988348, "acceleration"=50.00000000052296, "jerk"=1.1368683772161603e-07, "heading"=-0.0}, {"dt"=0.005, "x"=117.2112925000035, "y"=232.0, "position"=-117.2113237500035, "velocity"=-16.761999999991417, "acceleration"=49.99999999938609, "jerk"=-2.2737367544323206e-07, "heading"=-0.0}, {"dt"=0.005, "x"=117.29385250000345, "y"=232.0, "position"=-117.29388375000346, "velocity"=-16.511999999991644, "acceleration"=49.999999999954525, "jerk"=1.1368683772161603e-07, "heading"=-0.0}, {"dt"=0.005, "x"=117.37516250000338, "y"=232.0, "position"=-117.37519375000339, "velocity"=-16.261999999986188, "acceleration"=50.000000001091394, "jerk"=2.2737367544323206e-07, "heading"=-0.0}, {"dt"=0.005, "x"=117.45522250000334, "y"=232.0, "position"=-117.45525375000335, "velocity"=-16.0119999999921, "acceleration"=49.99999999881766, "jerk"=-4.547473508864641e-07, "heading"=-0.0}, {"dt"=0.005, "x"=117.53403250000332, "y"=232.0, "position"=-117.53406375000333, "velocity"=-15.761999999995169, "acceleration"=49.99999999938609, "jerk"=1.1368683772161603e-07, "heading"=-0.0}, {"dt"=0.005, "x"=117.61159250000327, "y"=232.0, "position"=-117.61162375000328, "velocity"=-15.511999999989712, "acceleration"=50.000000001091394, "jerk"=3.410605131648481e-07, "heading"=-0.0}, {"dt"=0.005, "x"=117.68790250000323, "y"=232.0, "position"=-117.68793375000324, "velocity"=-15.261999999992781, "acceleration"=49.99999999938609, "jerk"=-3.410605131648481e-07, "heading"=-0.0}, {"dt"=0.005, "x"=117.76296250000318, "y"=232.0, "position"=-117.76299375000319, "velocity"=-15.011999999990167, "acceleration"=50.00000000052296, "jerk"=2.2737367544323206e-07, "heading"=-0.0}, {"dt"=0.005, "x"=117.83677250000312, "y"=232.0, "position"=-117.83680375000313, "velocity"=-14.761999999987552, "acceleration"=50.00000000052296, "jerk"=-0.0, "heading"=-0.0}, {"dt"=0.005, "x"=117.90933250000307, "y"=232.0, "position"=-117.90936375000308, "velocity"=-14.511999999990621, "acceleration"=49.99999999938609, "jerk"=-2.2737367544323206e-07, "heading"=-0.0}, {"dt"=0.005, "x"=117.98064250000303, "y"=232.0, "position"=-117.98067375000304, "velocity"=-14.261999999990849, "acceleration"=49.999999999954525, "jerk"=1.1368683772161603e-07, "heading"=-0.0}, {"dt"=0.005, "x"=118.05070250000297, "y"=232.0, "position"=-118.05073375000298, "velocity"=-14.011999999988234, "acceleration"=50.00000000052296, "jerk"=1.1368683772161603e-07, "heading"=-0.0}, {"dt"=0.005, "x"=118.11951250000293, "y"=232.0, "position"=-118.11954375000293, "velocity"=-13.761999999991303, "acceleration"=49.99999999938609, "jerk"=-2.2737367544323206e-07, "heading"=-0.0}, {"dt"=0.005, "x"=118.18707250000287, "y"=232.0, "position"=-118.18710375000288, "velocity"=-13.511999999988689, "acceleration"=50.00000000052296, "jerk"=2.2737367544323206e-07, "heading"=-0.0}, {"dt"=0.005, "x"=118.25338250000283, "y"=232.0, "position"=-118.25341375000284, "velocity"=-13.261999999991758, "acceleration"=49.99999999938609, "jerk"=-2.2737367544323206e-07, "heading"=-0.0}, {"dt"=0.005, "x"=118.31844250000277, "y"=232.0, "position"=-118.31847375000278, "velocity"=-13.011999999989143, "acceleration"=50.00000000052296, "jerk"=2.2737367544323206e-07, "heading"=-0.0}, {"dt"=0.005, "x"=118.38225250000274, "y"=232.0, "position"=-118.38228375000274, "velocity"=-12.761999999992213, "acceleration"=49.99999999938609, "jerk"=-2.2737367544323206e-07, "heading"=-0.0}, {"dt"=0.005, "x"=118.44481250000268, "y"=232.0, "position"=-118.44484375000269, "velocity"=-12.511999999989598, "acceleration"=50.00000000052296, "jerk"=2.2737367544323206e-07, "heading"=-0.0}, {"dt"=0.005, "x"=118.50612250000265, "y"=232.0, "position"=-118.50615375000265, "velocity"=-12.261999999992668, "acceleration"=49.99999999938609, "jerk"=-2.2737367544323206e-07, "heading"=-0.0}, {"dt"=0.005, "x"=118.5661825000026, "y"=232.0, "position"=-118.5662137500026, "velocity"=-12.011999999990053, "acceleration"=50.00000000052296, "jerk"=2.2737367544323206e-07, "heading"=-0.0}, {"dt"=0.005, "x"=118.62499250000255, "y"=232.0, "position"=-118.62502375000255, "velocity"=-11.76199999999028, "acceleration"=49.999999999954525, "jerk"=-1.1368683772161603e-07, "heading"=-0.0}, {"dt"=0.005, "x"=118.68255250000249, "y"=232.0, "position"=-118.6825837500025, "velocity"=-11.511999999987665, "acceleration"=50.00000000052296, "jerk"=1.1368683772161603e-07, "heading"=-0.0}, {"dt"=0.005, "x"=118.73886250000244, "y"=232.0, "position"=-118.73889375000245, "velocity"=-11.261999999990735, "acceleration"=49.99999999938609, "jerk"=-2.2737367544323206e-07, "heading"=-0.0}, {"dt"=0.005, "x"=118.79392250000238, "y"=232.0, "position"=-118.79395375000239, "velocity"=-11.01199999998812, "acceleration"=50.00000000052296, "jerk"=2.2737367544323206e-07, "heading"=-0.0}, {"dt"=0.005, "x"=118.84773250000232, "y"=232.0, "position"=-118.84776375000233, "velocity"=-10.761999999988348, "acceleration"=49.999999999954525, "jerk"=-1.1368683772161603e-07, "heading"=-0.0}, {"dt"=0.005, "x"=118.90029250000228, "y"=232.0, "position"=-118.90032375000229, "velocity"=-10.511999999991417, "acceleration"=49.99999999938609, "jerk"=-1.1368683772161603e-07, "heading"=-0.0}, {"dt"=0.005, "x"=118.95160250000222, "y"=232.0, "position"=-118.95163375000223, "velocity"=-10.261999999988802, "acceleration"=50.00000000052296, "jerk"=2.2737367544323206e-07, "heading"=-0.0}, {"dt"=0.005, "x"=119.00166250000217, "y"=232.0, "position"=-119.00169375000218, "velocity"=-10.01199999998903, "acceleration"=49.999999999954525, "jerk"=-1.1368683772161603e-07, "heading"=-0.0}, {"dt"=0.005, "x"=119.05047250000212, "y"=232.0, "position"=-119.05050375000212, "velocity"=-9.761999999989257, "acceleration"=49.999999999954525, "jerk"=-0.0, "heading"=-0.0}, {"dt"=0.005, "x"=119.09803250000208, "y"=232.0, "position"=-119.09806375000208, "velocity"=-9.511999999992327, "acceleration"=49.99999999938609, "jerk"=-1.1368683772161603e-07, "heading"=-0.0}, {"dt"=0.005, "x"=119.14434250000204, "y"=232.0, "position"=-119.14437375000205, "velocity"=-9.261999999992554, "acceleration"=49.999999999954525, "jerk"=1.1368683772161603e-07, "heading"=-0.0}, {"dt"=0.005, "x"=119.18940250000199, "y"=232.0, "position"=-119.189433750002, "velocity"=-9.01199999998994, "acceleration"=50.00000000052296, "jerk"=1.1368683772161603e-07, "heading"=-0.0}, {"dt"=0.005, "x"=119.23321250000195, "y"=232.0, "position"=-119.23324375000196, "velocity"=-8.761999999993009, "acceleration"=49.99999999938609, "jerk"=-2.2737367544323206e-07, "heading"=-0.0}, {"dt"=0.005, "x"=119.27577250000189, "y"=232.0, "position"=-119.2758037500019, "velocity"=-8.511999999987552, "acceleration"=50.000000001091394, "jerk"=3.410605131648481e-07, "heading"=-0.0}, {"dt"=0.005, "x"=119.31708250000183, "y"=232.0, "position"=-119.31711375000184, "velocity"=-8.26199999998778, "acceleration"=49.999999999954525, "jerk"=-2.2737367544323206e-07, "heading"=-0.0}, {"dt"=0.005, "x"=119.35714250000179, "y"=232.0, "position"=-119.35717375000179, "velocity"=-8.011999999990849, "acceleration"=49.99999999938609, "jerk"=-1.1368683772161603e-07, "heading"=-0.0}, {"dt"=0.005, "x"=119.39595250000171, "y"=232.0, "position"=-119.39598375000172, "velocity"=-7.761999999985392, "acceleration"=50.000000001091394, "jerk"=3.410605131648481e-07, "heading"=-0.0}, {"dt"=0.005, "x"=119.43351250000167, "y"=232.0, "position"=-119.43354375000168, "velocity"=-7.511999999991303, "acceleration"=49.99999999881766, "jerk"=-4.547473508864641e-07, "heading"=-0.0}, {"dt"=0.005, "x"=119.46982250000163, "y"=232.0, "position"=-119.46985375000163, "velocity"=-7.261999999991531, "acceleration"=49.999999999954525, "jerk"=2.2737367544323206e-07, "heading"=-0.0}, {"dt"=0.005, "x"=119.50488250000157, "y"=232.0, "position"=-119.50491375000158, "velocity"=-7.011999999988916, "acceleration"=50.00000000052296, "jerk"=1.1368683772161603e-07, "heading"=-0.0}, {"dt"=0.005, "x"=119.53869250000152, "y"=232.0, "position"=-119.53872375000152, "velocity"=-6.761999999989143, "acceleration"=49.999999999954525, "jerk"=-1.1368683772161603e-07, "heading"=-0.0}, {"dt"=0.005, "x"=119.57125250000146, "y"=232.0, "position"=-119.57128375000147, "velocity"=-6.511999999989371, "acceleration"=49.999999999954525, "jerk"=-0.0, "heading"=-0.0}, {"dt"=0.005, "x"=119.60256250000143, "y"=232.0, "position"=-119.60259375000143, "velocity"=-6.26199999999244, "acceleration"=49.99999999938609, "jerk"=-1.1368683772161603e-07, "heading"=-0.0}, {"dt"=0.005, "x"=119.63262250000137, "y"=232.0, "position"=-119.63265375000138, "velocity"=-6.0119999999898255, "acceleration"=50.00000000052296, "jerk"=2.2737367544323206e-07, "heading"=-0.0}, {"dt"=0.005, "x"=119.66143250000133, "y"=232.0, "position"=-119.66146375000133, "velocity"=-5.761999999990053, "acceleration"=49.999999999954525, "jerk"=-1.1368683772161603e-07, "heading"=-0.0}, {"dt"=0.005, "x"=119.68899250000128, "y"=232.0, "position"=-119.68902375000128, "velocity"=-5.51199999999028, "acceleration"=49.999999999954525, "jerk"=-0.0, "heading"=-0.0}, {"dt"=0.005, "x"=119.7153025000012, "y"=232.0, "position"=-119.71533375000121, "velocity"=-5.261999999984823, "acceleration"=50.000000001091394, "jerk"=2.2737367544323206e-07, "heading"=-0.0}, {"dt"=0.005, "x"=119.74036250000115, "y"=232.0, "position"=-119.74039375000116, "velocity"=-5.011999999990735, "acceleration"=49.99999999881766, "jerk"=-4.547473508864641e-07, "heading"=-0.0}, {"dt"=0.005, "x"=119.76417250000108, "y"=232.0, "position"=-119.76420375000109, "velocity"=-4.761999999985278, "acceleration"=50.000000001091394, "jerk"=4.547473508864641e-07, "heading"=-0.0}, {"dt"=0.005, "x"=119.78673250000102, "y"=232.0, "position"=-119.78676375000103, "velocity"=-4.5119999999883476, "acceleration"=49.99999999938609, "jerk"=-3.410605131648481e-07, "heading"=-0.0}, {"dt"=0.005, "x"=119.80804250000098, "y"=232.0, "position"=-119.80807375000099, "velocity"=-4.261999999991417, "acceleration"=49.99999999938609, "jerk"=-0.0, "heading"=-0.0}, {"dt"=0.005, "x"=119.82810250000094, "y"=232.0, "position"=-119.82813375000094, "velocity"=-4.0119999999916445, "acceleration"=49.999999999954525, "jerk"=1.1368683772161603e-07, "heading"=-0.0}, {"dt"=0.005, "x"=119.84691250000087, "y"=232.0, "position"=-119.84694375000088, "velocity"=-3.7619999999861875, "acceleration"=50.000000001091394, "jerk"=2.2737367544323206e-07, "heading"=-0.0}, {"dt"=0.005, "x"=119.86447250000082, "y"=232.0, "position"=-119.86450375000082, "velocity"=-3.511999999989257, "acceleration"=49.99999999938609, "jerk"=-3.410605131648481e-07, "heading"=-0.0}, {"dt"=0.005, "x"=119.88078250000076, "y"=232.0, "position"=-119.88081375000077, "velocity"=-3.2619999999894844, "acceleration"=49.999999999954525, "jerk"=1.1368683772161603e-07, "heading"=-0.0}, {"dt"=0.005, "x"=119.89584250000071, "y"=232.0, "position"=-119.89587375000072, "velocity"=-3.011999999989712, "acceleration"=49.999999999954525, "jerk"=-0.0, "heading"=-0.0}, {"dt"=0.005, "x"=119.90965250000066, "y"=232.0, "position"=-119.90968375000067, "velocity"=-2.761999999989939, "acceleration"=49.999999999954525, "jerk"=-0.0, "heading"=-0.0}, {"dt"=0.005, "x"=119.92221250000061, "y"=232.0, "position"=-119.92224375000062, "velocity"=-2.5119999999901665, "acceleration"=49.999999999954525, "jerk"=-0.0, "heading"=-0.0}, {"dt"=0.005, "x"=119.93355225000059, "y"=232.0, "position"=-119.9335835000006, "velocity"=-2.267949999995267, "acceleration"=48.80999999897995, "jerk"=-238.00000019491563, "heading"=-0.0}, {"dt"=0.005, "x"=119.94373275000054, "y"=232.0, "position"=-119.94376400000054, "velocity"=-2.0360999999894602, "acceleration"=46.370000001161316, "jerk"=-487.9999995637263, "heading"=-0.0}, {"dt"=0.005, "x"=119.95281650000047, "y"=232.0, "position"=-119.95284775000047, "velocity"=-1.8167499999862002, "acceleration"=43.870000000652, "jerk"=-500.0000001018634, "heading"=-0.0}, {"dt"=0.005, "x"=119.96086600000042, "y"=232.0, "position"=-119.96089725000043, "velocity"=-1.6098999999911712, "acceleration"=41.36999999900581, "jerk"=-500.0000003292371, "heading"=-0.0}, {"dt"=0.005, "x"=119.96794375000037, "y"=232.0, "position"=-119.96797500000038, "velocity"=-1.4155499999901622, "acceleration"=38.8700000002018, "jerk"=-499.9999997608029, "heading"=-0.0}, {"dt"=0.005, "x"=119.97411225000033, "y"=232.0, "position"=-119.97414350000034, "velocity"=-1.2336999999916998, "acceleration"=36.36999999969248, "jerk"=-500.0000001018634, "heading"=-0.0}, {"dt"=0.005, "x"=119.97943400000031, "y"=232.0, "position"=-119.97946525000032, "velocity"=-1.064349999995784, "acceleration"=33.869999999183165, "jerk"=-500.0000001018634, "heading"=-0.0}, {"dt"=0.005, "x"=119.98397150000027, "y"=232.0, "position"=-119.98400275000027, "velocity"=-0.907499999991046, "acceleration"=31.370000000947584, "jerk"=-499.99999964711606, "heading"=-0.0}, {"dt"=0.005, "x"=119.98778725000024, "y"=232.0, "position"=-119.98781850000024, "velocity"=-0.763149999994539, "acceleration"=28.8699999993014, "jerk"=-500.0000003292371, "heading"=-0.0}, {"dt"=0.005, "x"=119.99094375000023, "y"=232.0, "position"=-119.99097500000023, "velocity"=-0.6312999999977364, "acceleration"=26.369999999360516, "jerk"=-499.99999998817657, "heading"=-0.0}, {"dt"=0.005, "x"=119.99350350000017, "y"=232.0, "position"=-119.99353475000018, "velocity"=-0.5119499999892696, "acceleration"=23.87000000169337, "jerk"=-499.9999995334292, "heading"=-0.0}, {"dt"=0.005, "x"=119.99552900000015, "y"=232.0, "position"=-119.99556025000015, "velocity"=-0.405099999994718, "acceleration"=21.369999998910316, "jerk"=-500.00000055661076, "heading"=-0.0}, {"dt"=0.005, "x"=119.99708275000015, "y"=232.0, "position"=-119.99711400000015, "velocity"=-0.31074999999987085, "acceleration"=18.869999998969433, "jerk"=-499.99999998817657, "heading"=-0.0}, {"dt"=0.005, "x"=119.99822725000011, "y"=232.0, "position"=-119.99825850000012, "velocity"=-0.22889999999335942, "acceleration"=16.370000001302287, "jerk"=-499.9999995334292, "heading"=-0.0}, {"dt"=0.005, "x"=119.99902500000012, "y"=232.0, "position"=-119.99905625000012, "velocity"=-0.15955000000076325, "acceleration"=13.869999998519233, "jerk"=-500.00000055661076, "heading"=-0.0}, {"dt"=0.005, "x"=119.99953850000009, "y"=232.0, "position"=-119.99956975000009, "velocity"=-0.10269999999366064, "acceleration"=11.370000001420522, "jerk"=-499.9999994197424, "heading"=-0.0}, {"dt"=0.005, "x"=119.99983025000007, "y"=232.0, "position"=-119.99986150000008, "velocity"=-0.05834999999763113, "acceleration"=8.869999999205902, "jerk"=-500.0000004429239, "heading"=-0.0}, {"dt"=0.005, "x"=119.99996275000007, "y"=232.0, "position"=-119.99999400000007, "velocity"=-0.026499999998463863, "acceleration"=6.369999999833453, "jerk"=-499.99999987448973, "heading"=-0.0}, {"dt"=0.005, "x"=119.99999850000006, "y"=232.0, "position"=-120.00002975000007, "velocity"=-0.007149999999001011, "acceleration"=3.8699999998925705, "jerk"=-499.99999998817657, "heading"=-0.0}, {"dt"=0.005, "x"=120.0, "y"=232.0, "position"=-120.00003125, "velocity"=-0.00029999998787388904, "acceleration"=1.3700000022254244, "jerk"=-499.9999995334292, "heading"=-0.0}, {"dt"=0.005, "x"=120.0, "y"=232.0, "position"=-120.00003125, "velocity"=-0.0, "acceleration"=0.05999999757477781, "jerk"=-262.0000009301293, "heading"=-0.0}], 6 "right":T2[](array[typedef])=[{"dt"=0.005, "x"=0.0, "y"=260.0, "position"=-3.125e-05, "velocity"=-0.0125, "acceleration"=-2.5, "jerk"=-500.0, "heading"=-0.0}, {"dt"=0.005, "x"=0.0, "y"=260.0, "position"=-3.125e-05, "velocity"=-0.0, "acceleration"=2.5, "jerk"=1000.0, "heading"=-0.0}, {"dt"=0.005, "x"=0.0, "y"=260.0, "position"=-3.125e-05, "velocity"=-0.0, "acceleration"=-0.0, "jerk"=-500.0, "heading"=-0.0}, {"dt"=0.005, "x"=0.0, "y"=260.0, "position"=-3.125e-05, "velocity"=-0.0, "acceleration"=-0.0, "jerk"=-0.0, "heading"=-0.0}, {"dt"=0.005, "x"=0.0, "y"=260.0, "position"=-3.125e-05, "velocity"=-0.0, "acceleration"=-0.0, "jerk"=-0.0, "heading"=-0.0}, {"dt"=0.005, "x"=0.0, "y"=260.0, "position"=-3.125e-05, "velocity"=-0.0, "acceleration"=-0.0, "jerk"=-0.0, "heading"=-0.0}, {"dt"=0.005, "x"=0.0, "y"=260.0, "position"=-3.125e-05, "velocity"=-0.0, "acceleration"=-0.0, "jerk"=-0.0, "heading"=-0.0}, {"dt"=0.005, "x"=0.0, "y"=260.0, "position"=-3.125e-05, "velocity"=-0.0, "acceleration"=-0.0, "jerk"=-0.0, "heading"=-0.0}, {"dt"=0.005, "x"=0.0, "y"=260.0, "position"=-3.125e-05, "velocity"=-0.0, "acceleration"=-0.0, "jerk"=-0.0, "heading"=-0.0}, {"dt"=0.005, "x"=3.124999999999981e-05, "y"=260.0, "position"=-6.249999999999981e-05, "velocity"=-0.006249999999999962, "acceleration"=-1.2499999999999925, "jerk"=-249.9999999999985, "heading"=-0.0}, {"dt"=0.005, "x"=0.003812499999999998, "y"=260.0, "position"=-0.0038437499999999978, "velocity"=-0.7562499999999996, "acceleration"=-149.99999999999994, "jerk"=-29749.99999999999, "heading"=-0.0}, {"dt"=0.005, "x"=0.008312499999999999, "y"=260.0, "position"=-0.008343749999999999, "velocity"=-0.9000000000000001, "acceleration"=-28.750000000000096, "jerk"=24249.999999999967, "heading"=-0.0}, {"dt"=0.005, "x"=0.013593749999999998, "y"=260.0, "position"=-0.013624999999999998, "velocity"=-1.05625, "acceleration"=-31.249999999999954, "jerk"=-499.9999999999716, "heading"=-0.0}, {"dt"=0.005, "x"=0.019718749999999997, "y"=260.0, "position"=-0.019749999999999997, "velocity"=-1.2249999999999996, "acceleration"=-33.74999999999994, "jerk"=-499.99999999999784, "heading"=-0.0}, {"dt"=0.005, "x"=0.026749999999999996, "y"=260.0, "position"=-0.026781249999999996, "velocity"=-1.4062499999999998, "acceleration"=-36.25000000000003, "jerk"=-500.00000000001705, "heading"=-0.0}, {"dt"=0.005, "x"=0.03474999999999999, "y"=260.0, "position"=-0.034781249999999986, "velocity"=-1.5999999999999985, "acceleration"=-38.74999999999975, "jerk"=-499.9999999999446, "heading"=-0.0}, {"dt"=0.005, "x"=0.04378125, "y"=260.0, "position"=-0.0438125, "velocity"=-1.8062500000000024, "acceleration"=-41.25000000000076, "jerk"=-500.0000000002018, "heading"=-0.0}, {"dt"=0.005, "x"=0.053906249999999996, "y"=260.0, "position"=-0.05393749999999999, "velocity"=-2.024999999999999, "acceleration"=-43.74999999999933, "jerk"=-499.99999999971436, "heading"=-0.0}, {"dt"=0.005, "x"=0.06518749999999998, "y"=260.0, "position"=-0.06521874999999998, "velocity"=-2.256249999999997, "acceleration"=-46.24999999999959, "jerk"=-500.00000000005116, "heading"=-0.0}, {"dt"=0.005, "x"=0.07768749999999996, "y"=260.0, "position"=-0.07771874999999996, "velocity"=-2.4999999999999964, "acceleration"=-48.74999999999989, "jerk"=-500.0000000000611, "heading"=-0.0}, {"dt"=0.005, "x"=0.09143749999999998, "y"=260.0, "position"=-0.09146874999999997, "velocity"=-2.750000000000002, "acceleration"=-50.00000000000115, "jerk"=-250.00000000025153, "heading"=-0.0}, {"dt"=0.005, "x"=0.10643749999999996, "y"=260.0, "position"=-0.10646874999999996, "velocity"=-2.999999999999997, "acceleration"=-49.999999999998934, "jerk"=4.433786671143025e-10, "heading"=-0.0}, {"dt"=0.005, "x"=0.12268749999999996, "y"=260.0, "position"=-0.12271874999999996, "velocity"=-3.25, "acceleration"=-50.00000000000062, "jerk"=-3.367972567502875e-10, "heading"=-0.0}, {"dt"=0.005, "x"=0.1401874999999999, "y"=260.0, "position"=-0.1402187499999999, "velocity"=-3.4999999999999893, "acceleration"=-49.99999999999787, "jerk"=5.499600774783175e-10, "heading"=-0.0}, {"dt"=0.005, "x"=0.1589374999999999, "y"=260.0, "position"=-0.15896874999999988, "velocity"=-3.749999999999998, "acceleration"=-50.000000000001684, "jerk"=-7.631228982063476e-10, "heading"=-0.0}, {"dt"=0.005, "x"=0.1789374999999999, "y"=260.0, "position"=-0.17896874999999987, "velocity"=-3.999999999999998, "acceleration"=-50.0, "jerk"=3.367972567502875e-10, "heading"=-0.0}, {"dt"=0.005, "x"=0.20018749999999985, "y"=260.0, "position"=-0.20021874999999983, "velocity"=-4.249999999999993, "acceleration"=-49.99999999999902, "jerk"=1.9610979506978765e-10, "heading"=-0.0}, {"dt"=0.005, "x"=0.22268749999999984, "y"=260.0, "position"=-0.22271874999999983, "velocity"=-4.499999999999998, "acceleration"=-50.000000000001066, "jerk"=-4.092726157978177e-10, "heading"=-0.0}, {"dt"=0.005, "x"=0.24643749999999992, "y"=260.0, "position"=-0.2464687499999999, "velocity"=-4.750000000000015, "acceleration"=-50.000000000003375, "jerk"=-4.618527782440651e-10, "heading"=-0.0}, {"dt"=0.005, "x"=0.2714375, "y"=260.0, "position"=-0.27146875, "velocity"=-5.000000000000015, "acceleration"=-50.0, "jerk"=6.750155989720952e-10, "heading"=-0.0}, {"dt"=0.005, "x"=0.2976875, "y"=260.0, "position"=-0.29771875, "velocity"=-5.249999999999999, "acceleration"=-49.9999999999968, "jerk"=6.394884621840902e-10, "heading"=-0.0}, {"dt"=0.005, "x"=0.3251875000000001, "y"=260.0, "position"=-0.32521875000000006, "velocity"=-5.500000000000016, "acceleration"=-50.000000000003375, "jerk"=-1.3145040611561853e-09, "heading"=-0.0}, {"dt"=0.005, "x"=0.3539375000000001, "y"=260.0, "position"=-0.3539687500000001, "velocity"=-5.750000000000011, "acceleration"=-49.999999999998934, "jerk"=8.881784197001252e-10, "heading"=-0.0}, {"dt"=0.005, "x"=0.38393750000000015, "y"=260.0, "position"=-0.38396875000000014, "velocity"=-6.000000000000005, "acceleration"=-49.999999999998934, "jerk"=-0.0, "heading"=-0.0}, {"dt"=0.005, "x"=0.4151875000000002, "y"=260.0, "position"=-0.4152187500000002, "velocity"=-6.250000000000011, "acceleration"=-50.000000000001066, "jerk"=-4.263256414560601e-10, "heading"=-0.0}, {"dt"=0.005, "x"=0.44768750000000024, "y"=260.0, "position"=-0.4477187500000002, "velocity"=-6.500000000000005, "acceleration"=-49.999999999998934, "jerk"=4.263256414560601e-10, "heading"=-0.0}, {"dt"=0.005, "x"=0.4814375000000002, "y"=260.0, "position"=-0.48146875000000017, "velocity"=-6.749999999999989, "acceleration"=-49.9999999999968, "jerk"=4.263256414560601e-10, "heading"=-0.0}, {"dt"=0.005, "x"=0.5164375000000001, "y"=260.0, "position"=-0.51646875, "velocity"=-6.999999999999984, "acceleration"=-49.999999999998934, "jerk"=-4.263256414560601e-10, "heading"=-0.0}, {"dt"=0.005, "x"=0.5526875, "y"=260.0, "position"=-0.5527187499999999, "velocity"=-7.249999999999979, "acceleration"=-49.999999999998934, "jerk"=-0.0, "heading"=-0.0}, {"dt"=0.005, "x"=0.5901874999999999, "y"=260.0, "position"=-0.5902187499999998, "velocity"=-7.499999999999973, "acceleration"=-49.999999999998934, "jerk"=-0.0, "heading"=-0.0}, {"dt"=0.005, "x"=0.6289374999999997, "y"=260.0, "position"=-0.6289687499999996, "velocity"=-7.749999999999968, "acceleration"=-49.999999999998934, "jerk"=-0.0, "heading"=-0.0}, {"dt"=0.005, "x"=0.6689374999999996, "y"=260.0, "position"=-0.6689687499999996, "velocity"=-7.999999999999985, "acceleration"=-50.000000000003375, "jerk"=-8.881784197001252e-10, "heading"=-0.0}, {"dt"=0.005, "x"=0.7101874999999995, "y"=260.0, "position"=-0.7102187499999995, "velocity"=-8.249999999999979, "acceleration"=-49.99999999999876, "jerk"=9.237055564881302e-10, "heading"=-0.0}, {"dt"=0.005, "x"=0.7526874999999994, "y"=260.0, "position"=-0.7527187499999993, "velocity"=-8.499999999999973, "acceleration"=-49.999999999998934, "jerk"=-3.552713678800501e-11, "heading"=-0.0}, {"dt"=0.005, "x"=0.7964374999999992, "y"=260.0, "position"=-0.7964687499999992, "velocity"=-8.749999999999968, "acceleration"=-49.999999999998934, "jerk"=-0.0, "heading"=-0.0}, {"dt"=0.005, "x"=0.8414374999999993, "y"=260.0, "position"=-0.8414687499999992, "velocity"=-9.000000000000007, "acceleration"=-50.000000000007816, "jerk"=-1.7763568394002505e-09, "heading"=-0.0}, {"dt"=0.005, "x"=0.8876874999999992, "y"=260.0, "position"=-0.8877187499999991, "velocity"=-9.24999999999998, "acceleration"=-49.99999999999467, "jerk"=2.6290081223123707e-09, "heading"=-0.0}, {"dt"=0.005, "x"=0.9351874999999988, "y"=260.0, "position"=-0.9352187499999988, "velocity"=-9.49999999999993, "acceleration"=-49.99999999999005, "jerk"=9.237055564881302e-10, "heading"=-0.0}, {"dt"=0.005, "x"=0.9839374999999992, "y"=260.0, "position"=-0.9839687499999992, "velocity"=-9.75000000000008, "acceleration"=-50.00000000002984, "jerk"=-7.958078640513122e-09, "heading"=-0.0}, {"dt"=0.005, "x"=1.0339374999999993, "y"=260.0, "position"=-1.0339687499999992, "velocity"=-10.000000000000009, "acceleration"=-49.99999999998579, "jerk"=8.810729923425242e-09, "heading"=-0.0}, {"dt"=0.005, "x"=1.0851874999999997, "y"=260.0, "position"=-1.0852187499999997, "velocity"=-10.250000000000092, "acceleration"=-50.0000000000167, "jerk"=-6.181721801112872e-09, "heading"=-0.0}, {"dt"=0.005, "x"=1.1376875, "y"=260.0, "position"=-1.13771875, "velocity"=-10.500000000000043, "acceleration"=-49.99999999999005, "jerk"=5.329070518200751e-09, "heading"=-0.0}, {"dt"=0.005, "x"=1.1914375000000004, "y"=260.0, "position"=-1.1914687500000003, "velocity"=-10.750000000000082, "acceleration"=-50.000000000007816, "jerk"=-3.552713678800501e-09, "heading"=-0.0}, {"dt"=0.005, "x"=1.2464375000000005, "y"=260.0, "position"=-1.2464687500000005, "velocity"=-11.000000000000032, "acceleration"=-49.99999999999005, "jerk"=3.552713678800501e-09, "heading"=-0.0}, {"dt"=0.005, "x"=1.3026875000000009, "y"=260.0, "position"=-1.3027187500000008, "velocity"=-11.250000000000071, "acceleration"=-50.000000000007816, "jerk"=-3.552713678800501e-09, "heading"=-0.0}, {"dt"=0.005, "x"=1.3601875000000012, "y"=260.0, "position"=-1.3602187500000011, "velocity"=-11.500000000000066, "acceleration"=-49.999999999998934, "jerk"=1.7763568394002505e-09, "heading"=-0.0}, {"dt"=0.005, "x"=1.418937500000002, "y"=260.0, "position"=-1.4189687500000019, "velocity"=-11.75000000000015, "acceleration"=-50.0000000000167, "jerk"=-3.552713678800501e-09, "heading"=-0.0}, {"dt"=0.005, "x"=1.4789375000000022, "y"=260.0, "position"=-1.4789687500000022, "velocity"=-12.000000000000055, "acceleration"=-49.99999999998117, "jerk"=7.105427357601002e-09, "heading"=-0.0}, {"dt"=0.005, "x"=1.5401875000000025, "y"=260.0, "position"=-1.5402187500000024, "velocity"=-12.25000000000005, "acceleration"=-49.999999999998934, "jerk"=-3.552713678800501e-09, "heading"=-0.0}, {"dt"=0.005, "x"=1.602687500000003, "y"=260.0, "position"=-1.6027187500000029, "velocity"=-12.500000000000089, "acceleration"=-50.000000000007816, "jerk"=-1.7763568394002505e-09, "heading"=-0.0}, {"dt"=0.005, "x"=1.6664375000000031, "y"=260.0, "position"=-1.666468750000003, "velocity"=-12.750000000000039, "acceleration"=-49.99999999999005, "jerk"=3.552713678800501e-09, "heading"=-0.0}, {"dt"=0.005, "x"=1.7314375000000037, "y"=260.0, "position"=-1.7314687500000037, "velocity"=-13.000000000000123, "acceleration"=-50.0000000000167, "jerk"=-5.329070518200751e-09, "heading"=-0.0}, {"dt"=0.005, "x"=1.7976875000000039, "y"=260.0, "position"=-1.7977187500000038, "velocity"=-13.250000000000028, "acceleration"=-49.99999999998117, "jerk"=7.105427357601002e-09, "heading"=-0.0}, {"dt"=0.005, "x"=1.8651875000000044, "y"=260.0, "position"=-1.8652187500000044, "velocity"=-13.500000000000112, "acceleration"=-50.0000000000167, "jerk"=-7.105427357601002e-09, "heading"=-0.0}, {"dt"=0.005, "x"=1.9339375000000047, "y"=260.0, "position"=-1.9339687500000047, "velocity"=-13.750000000000062, "acceleration"=-49.99999999999005, "jerk"=5.329070518200751e-09, "heading"=-0.0}, {"dt"=0.005, "x"=2.0039375000000055, "y"=260.0, "position"=-2.0039687500000056, "velocity"=-14.000000000000146, "acceleration"=-50.0000000000167, "jerk"=-5.329070518200751e-09, "heading"=-0.0}, {"dt"=0.005, "x"=2.075187500000006, "y"=260.0, "position"=-2.075218750000006, "velocity"=-14.250000000000096, "acceleration"=-49.99999999999005, "jerk"=5.329070518200751e-09, "heading"=-0.0}, {"dt"=0.005, "x"=2.1476875000000057, "y"=260.0, "position"=-2.147718750000006, "velocity"=-14.499999999999957, "acceleration"=-49.99999999997229, "jerk"=3.552713678800501e-09, "heading"=-0.0}, {"dt"=0.005, "x"=2.2214375000000066, "y"=260.0, "position"=-2.2214687500000068, "velocity"=-14.750000000000174, "acceleration"=-50.00000000004334, "jerk"=-1.4210854715202004e-08, "heading"=-0.0}, {"dt"=0.005, "x"=2.296437500000007, "y"=260.0, "position"=-2.296468750000007, "velocity"=-15.000000000000036, "acceleration"=-49.99999999997229, "jerk"=1.4210854715202004e-08, "heading"=-0.0}, {"dt"=0.005, "x"=2.3726875000000076, "y"=260.0, "position"=-2.3727187500000078, "velocity"=-15.250000000000163, "acceleration"=-50.00000000002558, "jerk"=-1.0658141036401503e-08, "heading"=-0.0}, {"dt"=0.005, "x"=2.450187500000008, "y"=260.0, "position"=-2.4502187500000083, "velocity"=-15.500000000000114, "acceleration"=-49.99999999999005, "jerk"=7.105427357601002e-09, "heading"=-0.0}, {"dt"=0.005, "x"=2.5289375000000085, "y"=260.0, "position"=-2.5289687500000086, "velocity"=-15.750000000000064, "acceleration"=-49.99999999999005, "jerk"=-0.0, "heading"=-0.0}, {"dt"=0.005, "x"=2.608937500000009, "y"=260.0, "position"=-2.608968750000009, "velocity"=-16.000000000000103, "acceleration"=-50.000000000007816, "jerk"=-3.552713678800501e-09, "heading"=-0.0}, {"dt"=0.005, "x"=2.6901875000000093, "y"=260.0, "position"=-2.6902187500000094, "velocity"=-16.250000000000053, "acceleration"=-49.99999999999005, "jerk"=3.552713678800501e-09, "heading"=-0.0}, {"dt"=0.005, "x"=2.7726875000000097, "y"=260.0, "position"=-2.77271875000001, "velocity"=-16.500000000000092, "acceleration"=-50.000000000007816, "jerk"=-3.552713678800501e-09, "heading"=-0.0}, {"dt"=0.005, "x"=2.8564375000000104, "y"=260.0, "position"=-2.8564687500000105, "velocity"=-16.75000000000013, "acceleration"=-50.000000000007816, "jerk"=-0.0, "heading"=-0.0}, {"dt"=0.005, "x"=2.9414375000000113, "y"=260.0, "position"=-2.9414687500000114, "velocity"=-17.00000000000017, "acceleration"=-50.000000000007816, "jerk"=-0.0, "heading"=-0.0}, {"dt"=0.005, "x"=3.027687500000012, "y"=260.0, "position"=-3.027718750000012, "velocity"=-17.25000000000012, "acceleration"=-49.99999999999005, "jerk"=3.552713678800501e-09, "heading"=-0.0}, {"dt"=0.005, "x"=3.115187500000012, "y"=260.0, "position"=-3.1152187500000124, "velocity"=-17.50000000000007, "acceleration"=-49.99999999999005, "jerk"=-0.0, "heading"=-0.0}, {"dt"=0.005, "x"=3.2039375000000128, "y"=260.0, "position"=-3.203968750000013, "velocity"=-17.75000000000011, "acceleration"=-50.000000000007816, "jerk"=-3.552713678800501e-09, "heading"=-0.0}, {"dt"=0.005, "x"=3.293937500000013, "y"=260.0, "position"=-3.293968750000013, "velocity"=-18.00000000000006, "acceleration"=-49.99999999999005, "jerk"=3.552713678800501e-09, "heading"=-0.0}, {"dt"=0.005, "x"=3.3851875000000136, "y"=260.0, "position"=-3.3852187500000137, "velocity"=-18.2500000000001, "acceleration"=-50.000000000007816, "jerk"=-3.552713678800501e-09, "heading"=-0.0}, {"dt"=0.005, "x"=3.4776875000000143, "y"=260.0, "position"=-3.4777187500000144, "velocity"=-18.50000000000014, "acceleration"=-50.000000000007816, "jerk"=-0.0, "heading"=-0.0}, {"dt"=0.005, "x"=3.5714375000000147, "y"=260.0, "position"=-3.571468750000015, "velocity"=-18.75000000000009, "acceleration"=-49.99999999999005, "jerk"=3.552713678800501e-09, "heading"=-0.0}, {"dt"=0.005, "x"=3.6664375000000153, "y"=260.0, "position"=-3.6664687500000155, "velocity"=-19.000000000000128, "acceleration"=-50.000000000007816, "jerk"=-3.552713678800501e-09, "heading"=-0.0}, {"dt"=0.005, "x"=3.762687500000014, "y"=260.0, "position"=-3.762718750000014, "velocity"=-19.249999999999723, "acceleration"=-49.999999999919, "jerk"=1.7763568394002505e-08, "heading"=-0.0}, {"dt"=0.005, "x"=3.8601875000000123, "y"=260.0, "position"=-3.8602187500000125, "velocity"=-19.499999999999673, "acceleration"=-49.99999999999005, "jerk"=-1.4210854715202004e-08, "heading"=-0.0}, {"dt"=0.005, "x"=3.958937500000009, "y"=260.0, "position"=-3.9589687500000093, "velocity"=-19.749999999999357, "acceleration"=-49.99999999993676, "jerk"=1.0658141036401503e-08, "heading"=-0.0}, {"dt"=0.005, "x"=4.058937500000005, "y"=260.0, "position"=-4.058968750000005, "velocity"=-19.99999999999922, "acceleration"=-49.99999999997229, "jerk"=-7.105427357601002e-09, "heading"=-0.0}, {"dt"=0.005, "x"=4.160187500000004, "y"=260.0, "position"=-4.160218750000004, "velocity"=-20.2499999999997, "acceleration"=-50.000000000096634, "jerk"=-2.4868995751603507e-08, "heading"=-0.0}, {"dt"=0.005, "x"=4.2626875, "y"=260.0, "position"=-4.26271875, "velocity"=-20.499999999999297, "acceleration"=-49.999999999919, "jerk"=3.552713678800501e-08, "heading"=-0.0}, {"dt"=0.005, "x"=4.366437499999997, "y"=260.0, "position"=-4.3664687499999975, "velocity"=-20.749999999999424, "acceleration"=-50.00000000002558, "jerk"=-2.1316282072803006e-08, "heading"=-0.0}, {"dt"=0.005, "x"=4.471437499999994, "y"=260.0, "position"=-4.471468749999994, "velocity"=-20.999999999999375, "acceleration"=-49.99999999999005, "jerk"=7.105427357601002e-09, "heading"=-0.0}, {"dt"=0.005, "x"=4.577687499999992, "y"=260.0, "position"=-4.577718749999992, "velocity"=-21.249999999999503, "acceleration"=-50.00000000002558, "jerk"=-7.105427357601002e-09, "heading"=-0.0}, {"dt"=0.005, "x"=4.685187499999989, "y"=260.0, "position"=-4.685218749999989, "velocity"=-21.499999999999453, "acceleration"=-49.99999999999005, "jerk"=7.105427357601002e-09, "heading"=-0.0}, {"dt"=0.005, "x"=4.793937499999985, "y"=260.0, "position"=-4.793968749999985, "velocity"=-21.749999999999226, "acceleration"=-49.999999999954525, "jerk"=7.105427357601002e-09, "heading"=-0.0}, {"dt"=0.005, "x"=4.903937499999983, "y"=260.0, "position"=-4.903968749999983, "velocity"=-21.99999999999953, "acceleration"=-50.00000000006111, "jerk"=-2.1316282072803006e-08, "heading"=-0.0}, {"dt"=0.005, "x"=5.015187499999979, "y"=260.0, "position"=-5.015218749999979, "velocity"=-22.249999999999304, "acceleration"=-49.999999999954525, "jerk"=2.1316282072803006e-08, "heading"=-0.0}, {"dt"=0.005, "x"=5.1276874999999755, "y"=260.0, "position"=-5.127718749999976, "velocity"=-22.499999999999254, "acceleration"=-49.99999999999005, "jerk"=-7.105427357601002e-09, "heading"=-0.0}, {"dt"=0.005, "x"=5.241437499999972, "y"=260.0, "position"=-5.241468749999973, "velocity"=-22.749999999999382, "acceleration"=-50.00000000002558, "jerk"=-7.105427357601002e-09, "heading"=-0.0}, {"dt"=0.005, "x"=5.356437499999968, "y"=260.0, "position"=-5.356468749999968, "velocity"=-22.999999999999154, "acceleration"=-49.999999999954525, "jerk"=1.4210854715202004e-08, "heading"=-0.0}, {"dt"=0.005, "x"=5.4726874999999655, "y"=260.0, "position"=-5.472718749999966, "velocity"=-23.24999999999946, "acceleration"=-50.00000000006111, "jerk"=-2.1316282072803006e-08, "heading"=-0.0}, {"dt"=0.005, "x"=5.590187499999963, "y"=260.0, "position"=-5.590218749999963, "velocity"=-23.49999999999941, "acceleration"=-49.99999999999005, "jerk"=1.4210854715202004e-08, "heading"=-0.0}, {"dt"=0.005, "x"=5.708937499999959, "y"=260.0, "position"=-5.7089687499999595, "velocity"=-23.74999999999936, "acceleration"=-49.99999999999005, "jerk"=-0.0, "heading"=-0.0}, {"dt"=0.005, "x"=5.828937499999956, "y"=260.0, "position"=-5.828968749999956, "velocity"=-23.99999999999931, "acceleration"=-49.99999999999005, "jerk"=-0.0, "heading"=-0.0}, {"dt"=0.005, "x"=5.950187499999952, "y"=260.0, "position"=-5.950218749999952, "velocity"=-24.24999999999926, "acceleration"=-49.99999999999005, "jerk"=-0.0, "heading"=-0.0}, {"dt"=0.005, "x"=6.072687499999948, "y"=260.0, "position"=-6.072718749999948, "velocity"=-24.49999999999921, "acceleration"=-49.99999999999005, "jerk"=-0.0, "heading"=-0.0}, {"dt"=0.005, "x"=6.196437499999945, "y"=260.0, "position"=-6.196468749999945, "velocity"=-24.74999999999934, "acceleration"=-50.00000000002558, "jerk"=-7.105427357601002e-09, "heading"=-0.0}, {"dt"=0.005, "x"=6.321437499999941, "y"=260.0, "position"=-6.321468749999942, "velocity"=-24.99999999999929, "acceleration"=-49.99999999999005, "jerk"=7.105427357601002e-09, "heading"=-0.0}, {"dt"=0.005, "x"=6.447687499999938, "y"=260.0, "position"=-6.447718749999938, "velocity"=-25.24999999999924, "acceleration"=-49.99999999999005, "jerk"=-0.0, "heading"=-0.0}, {"dt"=0.005, "x"=6.5751874999999345, "y"=260.0, "position"=-6.575218749999935, "velocity"=-25.499999999999368, "acceleration"=-50.00000000002558, "jerk"=-7.105427357601002e-09, "heading"=-0.0}, {"dt"=0.005, "x"=6.703937499999931, "y"=260.0, "position"=-6.703968749999931, "velocity"=-25.749999999999318, "acceleration"=-49.99999999999005, "jerk"=7.105427357601002e-09, "heading"=-0.0}, {"dt"=0.005, "x"=6.833937499999927, "y"=260.0, "position"=-6.8339687499999275, "velocity"=-25.999999999999268, "acceleration"=-49.99999999999005, "jerk"=-0.0, "heading"=-0.0}, {"dt"=0.005, "x"=6.965187499999923, "y"=260.0, "position"=-6.965218749999923, "velocity"=-26.24999999999904, "acceleration"=-49.999999999954525, "jerk"=7.105427357601002e-09, "heading"=-0.0}, {"dt"=0.005, "x"=7.09768749999992, "y"=260.0, "position"=-7.09771874999992, "velocity"=-26.499999999999524, "acceleration"=-50.000000000096634, "jerk"=-2.8421709430404007e-08, "heading"=-0.0}, {"dt"=0.005, "x"=7.231437499999915, "y"=260.0, "position"=-7.231468749999915, "velocity"=-26.74999999999894, "acceleration"=-49.99999999988347, "jerk"=4.263256414560601e-08, "heading"=-0.0}, {"dt"=0.005, "x"=7.366437499999912, "y"=260.0, "position"=-7.366468749999912, "velocity"=-26.999999999999424, "acceleration"=-50.000000000096634, "jerk"=-4.263256414560601e-08, "heading"=-0.0}, {"dt"=0.005, "x"=7.502687499999908, "y"=260.0, "position"=-7.502718749999908, "velocity"=-27.249999999999197, "acceleration"=-49.999999999954525, "jerk"=2.8421709430404007e-08, "heading"=-0.0}, {"dt"=0.005, "x"=7.640187499999904, "y"=260.0, "position"=-7.640218749999904, "velocity"=-27.499999999999147, "acceleration"=-49.99999999999005, "jerk"=-7.105427357601002e-09, "heading"=-0.0}, {"dt"=0.005, "x"=7.7789374999999, "y"=260.0, "position"=-7.7789687499999, "velocity"=-27.749999999999275, "acceleration"=-50.00000000002558, "jerk"=-7.105427357601002e-09, "heading"=-0.0}, {"dt"=0.005, "x"=7.918937499999897, "y"=260.0, "position"=-7.918968749999897, "velocity"=-27.999999999999403, "acceleration"=-50.00000000002558, "jerk"=-0.0, "heading"=-0.0}, {"dt"=0.005, "x"=8.060187499999891, "y"=260.0, "position"=-8.06021874999989, "velocity"=-28.24999999999882, "acceleration"=-49.99999999988347, "jerk"=2.8421709430404007e-08, "heading"=-0.0}, {"dt"=0.005, "x"=8.20268749999989, "y"=260.0, "position"=-8.202718749999889, "velocity"=-28.49999999999966, "acceleration"=-50.00000000016769, "jerk"=-5.6843418860808015e-08, "heading"=-0.0}, {"dt"=0.005, "x"=8.346437499999885, "y"=260.0, "position"=-8.346468749999884, "velocity"=-28.749999999999076, "acceleration"=-49.99999999988347, "jerk"=5.6843418860808015e-08, "heading"=-0.0}, {"dt"=0.005, "x"=8.491437499999881, "y"=260.0, "position"=-8.49146874999988, "velocity"=-28.999999999999204, "acceleration"=-50.00000000002558, "jerk"=-2.8421709430404007e-08, "heading"=-0.0}, {"dt"=0.005, "x"=8.637687499999876, "y"=260.0, "position"=-8.637718749999875, "velocity"=-29.249999999998977, "acceleration"=-49.999999999954525, "jerk"=1.4210854715202004e-08, "heading"=-0.0}, {"dt"=0.005, "x"=8.785187499999873, "y"=260.0, "position"=-8.785218749999872, "velocity"=-29.49999999999946, "acceleration"=-50.000000000096634, "jerk"=-2.8421709430404007e-08, "heading"=-0.0}, {"dt"=0.005, "x"=8.933937499999868, "y"=260.0, "position"=-8.933968749999867, "velocity"=-29.749999999998877, "acceleration"=-49.99999999988347, "jerk"=4.263256414560601e-08, "heading"=-0.0}, {"dt"=0.005, "x"=9.083937499999864, "y"=260.0, "position"=-9.083968749999864, "velocity"=-29.99999999999936, "acceleration"=-50.000000000096634, "jerk"=-4.263256414560601e-08, "heading"=-0.0}, {"dt"=0.005, "x"=9.235187499999858, "y"=260.0, "position"=-9.235218749999857, "velocity"=-30.249999999998778, "acceleration"=-49.99999999988347, "jerk"=4.263256414560601e-08, "heading"=-0.0}, {"dt"=0.005, "x"=9.387687499999853, "y"=260.0, "position"=-9.387718749999852, "velocity"=-30.499999999998906, "acceleration"=-50.00000000002558, "jerk"=-2.8421709430404007e-08, "heading"=-0.0}, {"dt"=0.005, "x"=9.541437499999851, "y"=260.0, "position"=-9.54146874999985, "velocity"=-30.749999999999744, "acceleration"=-50.00000000016769, "jerk"=-2.8421709430404007e-08, "heading"=-0.0}, {"dt"=0.005, "x"=9.696437499999845, "y"=260.0, "position"=-9.696468749999845, "velocity"=-30.999999999998806, "acceleration"=-49.99999999981242, "jerk"=7.105427357601002e-08, "heading"=-0.0}, {"dt"=0.005, "x"=9.85268749999984, "y"=260.0, "position"=-9.85271874999984, "velocity"=-31.249999999998934, "acceleration"=-50.00000000002558, "jerk"=-4.263256414560601e-08, "heading"=-0.0}, {"dt"=0.005, "x"=10.010187499999837, "y"=260.0, "position"=-10.010218749999837, "velocity"=-31.499999999999417, "acceleration"=-50.000000000096634, "jerk"=-1.4210854715202004e-08, "heading"=-0.0}, {"dt"=0.005, "x"=10.168937499999831, "y"=260.0, "position"=-10.16896874999983, "velocity"=-31.749999999998835, "acceleration"=-49.99999999988347, "jerk"=4.263256414560601e-08, "heading"=-0.0}, {"dt"=0.005, "x"=10.328937499999828, "y"=260.0, "position"=-10.328968749999827, "velocity"=-31.999999999999318, "acceleration"=-50.000000000096634, "jerk"=-4.263256414560601e-08, "heading"=-0.0}, {"dt"=0.005, "x"=10.490187499999823, "y"=260.0, "position"=-10.490218749999823, "velocity"=-32.24999999999909, "acceleration"=-49.999999999954525, "jerk"=2.8421709430404007e-08, "heading"=-0.0}, {"dt"=0.005, "x"=10.65268749999982, "y"=260.0, "position"=-10.652718749999819, "velocity"=-32.49999999999922, "acceleration"=-50.00000000002558, "jerk"=-1.4210854715202004e-08, "heading"=-0.0}, {"dt"=0.005, "x"=10.816437499999815, "y"=260.0, "position"=-10.816468749999814, "velocity"=-32.74999999999899, "acceleration"=-49.999999999954525, "jerk"=1.4210854715202004e-08, "heading"=-0.0}, {"dt"=0.005, "x"=10.98143749999981, "y"=260.0, "position"=-10.98146874999981, "velocity"=-32.99999999999912, "acceleration"=-50.00000000002558, "jerk"=-1.4210854715202004e-08, "heading"=-0.0}, {"dt"=0.005, "x"=11.147687499999805, "y"=260.0, "position"=-11.147718749999804, "velocity"=-33.24999999999889, "acceleration"=-49.999999999954525, "jerk"=1.4210854715202004e-08, "heading"=-0.0}, {"dt"=0.005, "x"=11.3151874999998, "y"=260.0, "position"=-11.315218749999799, "velocity"=-33.49999999999902, "acceleration"=-50.00000000002558, "jerk"=-1.4210854715202004e-08, "heading"=-0.0}, {"dt"=0.005, "x"=11.483937499999794, "y"=260.0, "position"=-11.483968749999793, "velocity"=-33.74999999999879, "acceleration"=-49.999999999954525, "jerk"=1.4210854715202004e-08, "heading"=-0.0}, {"dt"=0.005, "x"=11.653937499999788, "y"=260.0, "position"=-11.653968749999787, "velocity"=-33.99999999999892, "acceleration"=-50.00000000002558, "jerk"=-1.4210854715202004e-08, "heading"=-0.0}, {"dt"=0.005, "x"=11.825187499999783, "y"=260.0, "position"=-11.825218749999783, "velocity"=-34.24999999999905, "acceleration"=-50.00000000002558, "jerk"=-0.0, "heading"=-0.0}, {"dt"=0.005, "x"=11.997687499999781, "y"=260.0, "position"=-11.99771874999978, "velocity"=-34.49999999999953, "acceleration"=-50.000000000096634, "jerk"=-1.4210854715202004e-08, "heading"=-0.0}, {"dt"=0.005, "x"=12.171437499999774, "y"=260.0, "position"=-12.171468749999773, "velocity"=-34.74999999999859, "acceleration"=-49.99999999981242, "jerk"=5.6843418860808015e-08, "heading"=-0.0}, {"dt"=0.005, "x"=12.346437499999771, "y"=260.0, "position"=-12.34646874999977, "velocity"=-34.99999999999943, "acceleration"=-50.00000000016769, "jerk"=-7.105427357601002e-08, "heading"=-0.0}, {"dt"=0.005, "x"=12.522687499999764, "y"=260.0, "position"=-12.522718749999763, "velocity"=-35.249999999998494, "acceleration"=-49.99999999981242, "jerk"=7.105427357601002e-08, "heading"=-0.0}, {"dt"=0.005, "x"=12.700187499999759, "y"=260.0, "position"=-12.700218749999758, "velocity"=-35.49999999999898, "acceleration"=-50.000000000096634, "jerk"=-5.6843418860808015e-08, "heading"=-0.0}, {"dt"=0.005, "x"=12.878937499999756, "y"=260.0, "position"=-12.878968749999755, "velocity"=-35.74999999999946, "acceleration"=-50.000000000096634, "jerk"=-0.0, "heading"=-0.0}, {"dt"=0.005, "x"=13.058937499999749, "y"=260.0, "position"=-13.058968749999748, "velocity"=-35.99999999999852, "acceleration"=-49.99999999981242, "jerk"=5.6843418860808015e-08, "heading"=-0.0}, {"dt"=0.005, "x"=13.240187499999745, "y"=260.0, "position"=-13.240218749999745, "velocity"=-36.24999999999936, "acceleration"=-50.00000000016769, "jerk"=-7.105427357601002e-08, "heading"=-0.0}, {"dt"=0.005, "x"=13.42268749999974, "y"=260.0, "position"=-13.422718749999738, "velocity"=-36.49999999999878, "acceleration"=-49.99999999988347, "jerk"=5.6843418860808015e-08, "heading"=-0.0}, {"dt"=0.005, "x"=13.606437499999734, "y"=260.0, "position"=-13.606468749999733, "velocity"=-36.749999999998906, "acceleration"=-50.00000000002558, "jerk"=-2.8421709430404007e-08, "heading"=-0.0}, {"dt"=0.005, "x"=13.791437499999729, "y"=260.0, "position"=-13.791468749999728, "velocity"=-36.999999999999034, "acceleration"=-50.00000000002558, "jerk"=-0.0, "heading"=-0.0}, {"dt"=0.005, "x"=13.977687499999725, "y"=260.0, "position"=-13.977718749999724, "velocity"=-37.24999999999916, "acceleration"=-50.00000000002558, "jerk"=-0.0, "heading"=-0.0}, {"dt"=0.005, "x"=14.165187499999718, "y"=260.0, "position"=-14.165218749999717, "velocity"=-37.49999999999858, "acceleration"=-49.99999999988347, "jerk"=2.8421709430404007e-08, "heading"=-0.0}, {"dt"=0.005, "x"=14.353937499999713, "y"=260.0, "position"=-14.353968749999712, "velocity"=-37.74999999999906, "acceleration"=-50.000000000096634, "jerk"=-4.263256414560601e-08, "heading"=-0.0}, {"dt"=0.005, "x"=14.543937499999707, "y"=260.0, "position"=-14.543968749999706, "velocity"=-37.999999999998835, "acceleration"=-49.999999999954525, "jerk"=2.8421709430404007e-08, "heading"=-0.0}, {"dt"=0.005, "x"=14.735187499999702, "y"=260.0, "position"=-14.735218749999701, "velocity"=-38.24999999999896, "acceleration"=-50.00000000002558, "jerk"=-1.4210854715202004e-08, "heading"=-0.0}, {"dt"=0.005, "x"=14.927687499999696, "y"=260.0, "position"=-14.927718749999695, "velocity"=-38.499999999998735, "acceleration"=-49.999999999954525, "jerk"=1.4210854715202004e-08, "heading"=-0.0}, {"dt"=0.005, "x"=15.121437499999708, "y"=260.0, "position"=-15.121468749999707, "velocity"=-38.750000000002416, "acceleration"=-50.00000000073612, "jerk"=-1.5631940186722204e-07, "heading"=-0.0}, {"dt"=0.005, "x"=15.316437499999733, "y"=260.0, "position"=-15.316468749999732, "velocity"=-39.00000000000503, "acceleration"=-50.00000000052296, "jerk"=4.263256414560601e-08, "heading"=-0.0}, {"dt"=0.005, "x"=15.512687499999753, "y"=260.0, "position"=-15.512718749999753, "velocity"=-39.25000000000409, "acceleration"=-49.99999999981242, "jerk"=1.4210854715202004e-07, "heading"=-0.0}, {"dt"=0.005, "x"=15.710187499999774, "y"=260.0, "position"=-15.710218749999774, "velocity"=-39.50000000000422, "acceleration"=-50.00000000002558, "jerk"=-4.263256414560601e-08, "heading"=-0.0}, {"dt"=0.005, "x"=15.908937499999794, "y"=260.0, "position"=-15.908968749999794, "velocity"=-39.75000000000399, "acceleration"=-49.999999999954525, "jerk"=1.4210854715202004e-08, "heading"=-0.0}, {"dt"=0.005, "x"=16.10893749999982, "y"=260.0, "position"=-16.108968749999818, "velocity"=-40.00000000000483, "acceleration"=-50.00000000016769, "jerk"=-4.263256414560601e-08, "heading"=-0.0}, {"dt"=0.005, "x"=16.31018749999984, "y"=260.0, "position"=-16.31021874999984, "velocity"=-40.250000000004604, "acceleration"=-49.999999999954525, "jerk"=4.263256414560601e-08, "heading"=-0.0}, {"dt"=0.005, "x"=16.512687499999863, "y"=260.0, "position"=-16.512718749999863, "velocity"=-40.50000000000438, "acceleration"=-49.999999999954525, "jerk"=-0.0, "heading"=-0.0}, {"dt"=0.005, "x"=16.716437499999884, "y"=260.0, "position"=-16.716468749999883, "velocity"=-40.75000000000415, "acceleration"=-49.999999999954525, "jerk"=-0.0, "heading"=-0.0}, {"dt"=0.005, "x"=16.92143749999991, "y"=260.0, "position"=-16.92146874999991, "velocity"=-41.00000000000534, "acceleration"=-50.00000000023874, "jerk"=-5.6843418860808015e-08, "heading"=-0.0}, {"dt"=0.005, "x"=17.127687499999933, "y"=260.0, "position"=-17.127718749999932, "velocity"=-41.250000000004405, "acceleration"=-49.99999999981242, "jerk"=8.526512829121202e-08, "heading"=-0.0}, {"dt"=0.005, "x"=17.335187499999954, "y"=260.0, "position"=-17.335218749999953, "velocity"=-41.50000000000418, "acceleration"=-49.999999999954525, "jerk"=-2.8421709430404007e-08, "heading"=-0.0}, {"dt"=0.005, "x"=17.543937499999974, "y"=260.0, "position"=-17.543968749999973, "velocity"=-41.75000000000395, "acceleration"=-49.999999999954525, "jerk"=-0.0, "heading"=-0.0}, {"dt"=0.005, "x"=17.7539375, "y"=260.0, "position"=-17.75396875, "velocity"=-42.000000000005144, "acceleration"=-50.00000000023874, "jerk"=-5.6843418860808015e-08, "heading"=-0.0}, {"dt"=0.005, "x"=17.96518750000002, "y"=260.0, "position"=-17.96521875000002, "velocity"=-42.250000000004206, "acceleration"=-49.99999999981242, "jerk"=8.526512829121202e-08, "heading"=-0.0}, {"dt"=0.005, "x"=18.177687500000044, "y"=260.0, "position"=-18.177718750000043, "velocity"=-42.50000000000469, "acceleration"=-50.000000000096634, "jerk"=-5.6843418860808015e-08, "heading"=-0.0}, {"dt"=0.005, "x"=18.391437500000066, "y"=260.0, "position"=-18.391468750000065, "velocity"=-42.75000000000446, "acceleration"=-49.999999999954525, "jerk"=2.8421709430404007e-08, "heading"=-0.0}, {"dt"=0.005, "x"=18.60643750000009, "y"=260.0, "position"=-18.60646875000009, "velocity"=-43.000000000004945, "acceleration"=-50.000000000096634, "jerk"=-2.8421709430404007e-08, "heading"=-0.0}, {"dt"=0.005, "x"=18.822687500000114, "y"=260.0, "position"=-18.822718750000114, "velocity"=-43.25000000000472, "acceleration"=-49.999999999954525, "jerk"=2.8421709430404007e-08, "heading"=-0.0}, {"dt"=0.005, "x"=19.04018750000014, "y"=260.0, "position"=-19.04021875000014, "velocity"=-43.5000000000052, "acceleration"=-50.000000000096634, "jerk"=-2.8421709430404007e-08, "heading"=-0.0}, {"dt"=0.005, "x"=19.25893750000016, "y"=260.0, "position"=-19.25896875000016, "velocity"=-43.75000000000426, "acceleration"=-49.99999999981242, "jerk"=5.6843418860808015e-08, "heading"=-0.0}, {"dt"=0.005, "x"=19.478937500000185, "y"=260.0, "position"=-19.478968750000185, "velocity"=-44.000000000004746, "acceleration"=-50.000000000096634, "jerk"=-5.6843418860808015e-08, "heading"=-0.0}, {"dt"=0.005, "x"=19.700187500000215, "y"=260.0, "position"=-19.700218750000214, "velocity"=-44.25000000000594, "acceleration"=-50.00000000023874, "jerk"=-2.8421709430404007e-08, "heading"=-0.0}, {"dt"=0.005, "x"=19.922687500000237, "y"=260.0, "position"=-19.922718750000236, "velocity"=-44.50000000000429, "acceleration"=-49.99999999967031, "jerk"=1.1368683772161603e-07, "heading"=-0.0}, {"dt"=0.005, "x"=20.14643750000026, "y"=260.0, "position"=-20.14646875000026, "velocity"=-44.750000000004775, "acceleration"=-50.000000000096634, "jerk"=-8.526512829121202e-08, "heading"=-0.0}, {"dt"=0.005, "x"=20.371437500000287, "y"=260.0, "position"=-20.371468750000286, "velocity"=-45.00000000000526, "acceleration"=-50.000000000096634, "jerk"=-0.0, "heading"=-0.0}, {"dt"=0.005, "x"=20.597687500000312, "y"=260.0, "position"=-20.59771875000031, "velocity"=-45.25000000000503, "acceleration"=-49.999999999954525, "jerk"=2.8421709430404007e-08, "heading"=-0.0}, {"dt"=0.005, "x"=20.825187500000336, "y"=260.0, "position"=-20.825218750000335, "velocity"=-45.5000000000048, "acceleration"=-49.999999999954525, "jerk"=-0.0, "heading"=-0.0}, {"dt"=0.005, "x"=21.05393750000036, "y"=260.0, "position"=-21.053968750000358, "velocity"=-45.750000000004576, "acceleration"=-49.999999999954525, "jerk"=-0.0, "heading"=-0.0}, {"dt"=0.005, "x"=21.283937500000388, "y"=260.0, "position"=-21.283968750000387, "velocity"=-46.00000000000577, "acceleration"=-50.00000000023874, "jerk"=-5.6843418860808015e-08, "heading"=-0.0}, {"dt"=0.005, "x"=21.515187500000412, "y"=260.0, "position"=-21.51521875000041, "velocity"=-46.25000000000483, "acceleration"=-49.99999999981242, "jerk"=8.526512829121202e-08, "heading"=-0.0}, {"dt"=0.005, "x"=21.74768750000044, "y"=260.0, "position"=-21.747718750000438, "velocity"=-46.500000000005315, "acceleration"=-50.000000000096634, "jerk"=-5.6843418860808015e-08, "heading"=-0.0}, {"dt"=0.005, "x"=21.981437500000467, "y"=260.0, "position"=-21.981468750000467, "velocity"=-46.7500000000058, "acceleration"=-50.000000000096634, "jerk"=-0.0, "heading"=-0.0}, {"dt"=0.005, "x"=22.21643750000049, "y"=260.0, "position"=-22.21646875000049, "velocity"=-47.00000000000486, "acceleration"=-49.99999999981242, "jerk"=5.6843418860808015e-08, "heading"=-0.0}, {"dt"=0.005, "x"=22.45268750000052, "y"=260.0, "position"=-22.452718750000518, "velocity"=-47.25000000000534, "acceleration"=-50.000000000096634, "jerk"=-5.6843418860808015e-08, "heading"=-0.0}, {"dt"=0.005, "x"=22.69018750000054, "y"=260.0, "position"=-22.69021875000054, "velocity"=-47.500000000004405, "acceleration"=-49.99999999981242, "jerk"=5.6843418860808015e-08, "heading"=-0.0}, {"dt"=0.005, "x"=22.92890625000057, "y"=260.0, "position"=-22.92893750000057, "velocity"=-47.74375000000575, "acceleration"=-48.7500000002683, "jerk"=249.99999990882316, "heading"=-0.0}, {"dt"=0.005, "x"=23.168781250000595, "y"=260.0, "position"=-23.168812500000595, "velocity"=-47.97500000000525, "acceleration"=-46.24999999990109, "jerk"=500.0000000734417, "heading"=-0.0}, {"dt"=0.005, "x"=23.409750000000624, "y"=260.0, "position"=-23.409781250000623, "velocity"=-48.193750000005764, "acceleration"=-43.75000000010232, "jerk"=499.99999995975486, "heading"=-0.0}, {"dt"=0.005, "x"=23.65175000000065, "y"=260.0, "position"=-23.65178125000065, "velocity"=-48.40000000000515, "acceleration"=-41.24999999987722, "jerk"=500.00000004502, "heading"=-0.0}, {"dt"=0.005, "x"=23.894718750000678, "y"=260.0, "position"=-23.894750000000677, "velocity"=-48.59375000000554, "acceleration"=-38.750000000078444, "jerk"=499.99999995975486, "heading"=-0.0}, {"dt"=0.005, "x"=24.1385937500007, "y"=260.0, "position"=-24.1386250000007, "velocity"=-48.77500000000481, "acceleration"=-36.249999999853344, "jerk"=500.00000004502, "heading"=-0.0}, {"dt"=0.005, "x"=24.383312500000727, "y"=260.0, "position"=-24.383343750000726, "velocity"=-48.94375000000508, "acceleration"=-33.75000000005457, "jerk"=499.99999995975486, "heading"=-0.0}, {"dt"=0.005, "x"=24.62881250000076, "y"=260.0, "position"=-24.628843750000758, "velocity"=-49.10000000000636, "acceleration"=-31.250000000255795, "jerk"=499.99999995975486, "heading"=-0.0}, {"dt"=0.005, "x"=24.875031250000788, "y"=260.0, "position"=-24.875062500000787, "velocity"=-49.243750000005804, "acceleration"=-28.749999999888587, "jerk"=500.0000000734417, "heading"=-0.0}, {"dt"=0.005, "x"=25.121906250000812, "y"=260.0, "position"=-25.12193750000081, "velocity"=-49.37500000000483, "acceleration"=-26.249999999805596, "jerk"=500.0000000165983, "heading"=-0.0}, {"dt"=0.005, "x"=25.36937500000084, "y"=260.0, "position"=-25.36940625000084, "velocity"=-49.493750000005576, "acceleration"=-23.75000000014893, "jerk"=499.99999993133315, "heading"=-0.0}, {"dt"=0.005, "x"=25.61737500000087, "y"=260.0, "position"=-25.61740625000087, "velocity"=-49.600000000005906, "acceleration"=-21.25000000006594, "jerk"=500.0000000165983, "heading"=-0.0}, {"dt"=0.005, "x"=25.865843750000895, "y"=260.0, "position"=-25.865875000000894, "velocity"=-49.69375000000511, "acceleration"=-18.74999999984084, "jerk"=500.00000004502, "heading"=-0.0}, {"dt"=0.005, "x"=26.114718750000925, "y"=260.0, "position"=-26.114750000000925, "velocity"=-49.77500000000603, "acceleration"=-16.250000000184173, "jerk"=499.99999993133315, "heading"=-0.0}, {"dt"=0.005, "x"=26.363937500000954, "y"=260.0, "position"=-26.363968750000954, "velocity"=-49.84375000000583, "acceleration"=-13.749999999959073, "jerk"=500.00000004502, "heading"=-0.0}, {"dt"=0.005, "x"=26.61343750000098, "y"=260.0, "position"=-26.61346875000098, "velocity"=-49.90000000000521, "acceleration"=-11.249999999876081, "jerk"=500.0000000165983, "heading"=-0.0}, {"dt"=0.005, "x"=26.86315625000101, "y"=260.0, "position"=-26.863187500001008, "velocity"=-49.94375000000559, "acceleration"=-8.750000000077307, "jerk"=499.99999995975486, "heading"=-0.0}, {"dt"=0.005, "x"=27.11303125000104, "y"=260.0, "position"=-27.11306250000104, "velocity"=-49.975000000006276, "acceleration"=-6.250000000136424, "jerk"=499.99999998817657, "heading"=-0.0}, {"dt"=0.005, "x"=27.363000000001062, "y"=260.0, "position"=-27.36303125000106, "velocity"=-49.99375000000441, "acceleration"=-3.749999999627107, "jerk"=500.0000001018634, "heading"=-0.0}, {"dt"=0.005, "x"=27.613000000001094, "y"=260.0, "position"=-27.613031250001093, "velocity"=-50.000000000006395, "acceleration"=-1.250000000396767, "jerk"=499.999999846068, "heading"=-0.0}, {"dt"=0.005, "x"=27.86300000000112, "y"=260.0, "position"=-27.863031250001118, "velocity"=-50.000000000004974, "acceleration"=2.842170943040401e-10, "jerk"=250.00000013619683, "heading"=-0.0}, {"dt"=0.005, "x"=28.113000000001147, "y"=260.0, "position"=-28.113031250001146, "velocity"=-50.000000000005684, "acceleration"=-1.4210854715202004e-10, "jerk"=-8.526512829121202e-08, "heading"=-0.0}, {"dt"=0.005, "x"=28.363000000001172, "y"=260.0, "position"=-28.36303125000117, "velocity"=-50.000000000004974, "acceleration"=1.4210854715202004e-10, "jerk"=5.6843418860808015e-08, "heading"=-0.0}, {"dt"=0.005, "x"=28.6130000000012, "y"=260.0, "position"=-28.6130312500012, "velocity"=-50.000000000005684, "acceleration"=-1.4210854715202004e-10, "jerk"=-5.6843418860808015e-08, "heading"=-0.0}, {"dt"=0.005, "x"=28.863000000001232, "y"=260.0, "position"=-28.86303125000123, "velocity"=-50.000000000006395, "acceleration"=-1.4210854715202004e-10, "jerk"=-0.0, "heading"=-0.0}, {"dt"=0.005, "x"=29.113000000001257, "y"=260.0, "position"=-29.113031250001256, "velocity"=-50.000000000004974, "acceleration"=2.842170943040401e-10, "jerk"=8.526512829121202e-08, "heading"=-0.0}, {"dt"=0.005, "x"=29.363000000001282, "y"=260.0, "position"=-29.36303125000128, "velocity"=-50.000000000004974, "acceleration"=-0.0, "jerk"=-5.6843418860808015e-08, "heading"=-0.0}, {"dt"=0.005, "x"=29.61300000000131, "y"=260.0, "position"=-29.61303125000131, "velocity"=-50.000000000005684, "acceleration"=-1.4210854715202004e-10, "jerk"=-2.8421709430404007e-08, "heading"=-0.0}, {"dt"=0.005, "x"=29.863000000001342, "y"=260.0, "position"=-29.86303125000134, "velocity"=-50.000000000006395, "acceleration"=-1.4210854715202004e-10, "jerk"=-0.0, "heading"=-0.0}, {"dt"=0.005, "x"=30.113000000001367, "y"=260.0, "position"=-30.113031250001367, "velocity"=-50.000000000004974, "acceleration"=2.842170943040401e-10, "jerk"=8.526512829121202e-08, "heading"=-0.0}, {"dt"=0.005, "x"=30.363000000001392, "y"=260.0, "position"=-30.36303125000139, "velocity"=-50.000000000004974, "acceleration"=-0.0, "jerk"=-5.6843418860808015e-08, "heading"=-0.0}, {"dt"=0.005, "x"=30.613000000001417, "y"=260.0, "position"=-30.613031250001416, "velocity"=-50.000000000004974, "acceleration"=-0.0, "jerk"=-0.0, "heading"=-0.0}, {"dt"=0.005, "x"=30.86300000000145, "y"=260.0, "position"=-30.86303125000145, "velocity"=-50.000000000006395, "acceleration"=-2.842170943040401e-10, "jerk"=-5.6843418860808015e-08, "heading"=-0.0}, {"dt"=0.005, "x"=31.113000000001477, "y"=260.0, "position"=-31.113031250001477, "velocity"=-50.000000000005684, "acceleration"=1.4210854715202004e-10, "jerk"=8.526512829121202e-08, "heading"=-0.0}, {"dt"=0.005, "x"=31.36300000000151, "y"=260.0, "position"=-31.36303125000151, "velocity"=-50.000000000006395, "acceleration"=-1.4210854715202004e-10, "jerk"=-5.6843418860808015e-08, "heading"=-0.0}, {"dt"=0.005, "x"=31.613000000001534, "y"=260.0, "position"=-31.613031250001534, "velocity"=-50.000000000004974, "acceleration"=2.842170943040401e-10, "jerk"=8.526512829121202e-08, "heading"=-0.0}, {"dt"=0.005, "x"=31.86300000000156, "y"=260.0, "position"=-31.86303125000156, "velocity"=-50.000000000004974, "acceleration"=-0.0, "jerk"=-5.6843418860808015e-08, "heading"=-0.0}, {"dt"=0.005, "x"=32.113000000001584, "y"=260.0, "position"=-32.11303125000158, "velocity"=-50.000000000004974, "acceleration"=-0.0, "jerk"=-0.0, "heading"=-0.0}, {"dt"=0.005, "x"=32.36300000000161, "y"=260.0, "position"=-32.36303125000161, "velocity"=-50.000000000005684, "acceleration"=-1.4210854715202004e-10, "jerk"=-2.8421709430404007e-08, "heading"=-0.0}, {"dt"=0.005, "x"=32.613000000001634, "y"=260.0, "position"=-32.61303125000163, "velocity"=-50.00000000000426, "acceleration"=2.842170943040401e-10, "jerk"=8.526512829121202e-08, "heading"=-0.0}, {"dt"=0.005, "x"=32.86300000000167, "y"=260.0, "position"=-32.86303125000167, "velocity"=-50.000000000007105, "acceleration"=-5.684341886080801e-10, "jerk"=-1.7053025658242404e-07, "heading"=-0.0}, {"dt"=0.005, "x"=33.113000000001705, "y"=260.0, "position"=-33.113031250001704, "velocity"=-50.000000000007105, "acceleration"=-0.0, "jerk"=1.1368683772161603e-07, "heading"=-0.0}, {"dt"=0.005, "x"=33.363000000001726, "y"=260.0, "position"=-33.363031250001725, "velocity"=-50.00000000000426, "acceleration"=5.684341886080801e-10, "jerk"=1.1368683772161603e-07, "heading"=-0.0}, {"dt"=0.005, "x"=33.613000000001755, "y"=260.0, "position"=-33.613031250001754, "velocity"=-50.000000000005684, "acceleration"=-2.842170943040401e-10, "jerk"=-1.7053025658242404e-07, "heading"=-0.0}, {"dt"=0.005, "x"=33.863000000001776, "y"=260.0, "position"=-33.863031250001775, "velocity"=-50.00000000000426, "acceleration"=2.842170943040401e-10, "jerk"=1.1368683772161603e-07, "heading"=-0.0}, {"dt"=0.005, "x"=34.113000000001804, "y"=260.0, "position"=-34.113031250001804, "velocity"=-50.000000000005684, "acceleration"=-2.842170943040401e-10, "jerk"=-1.1368683772161603e-07, "heading"=-0.0}, {"dt"=0.005, "x"=34.36300000000183, "y"=260.0, "position"=-34.36303125000183, "velocity"=-50.000000000005684, "acceleration"=-0.0, "jerk"=5.6843418860808015e-08, "heading"=-0.0}, {"dt"=0.005, "x"=34.61300000000186, "y"=260.0, "position"=-34.61303125000186, "velocity"=-50.000000000005684, "acceleration"=-0.0, "jerk"=-0.0, "heading"=-0.0}, {"dt"=0.005, "x"=34.8630000000019, "y"=260.0, "position"=-34.863031250001896, "velocity"=-50.000000000007105, "acceleration"=-2.842170943040401e-10, "jerk"=-5.6843418860808015e-08, "heading"=-0.0}, {"dt"=0.005, "x"=35.11300000000192, "y"=260.0, "position"=-35.11303125000192, "velocity"=-50.00000000000426, "acceleration"=5.684341886080801e-10, "jerk"=1.7053025658242404e-07, "heading"=-0.0}, {"dt"=0.005, "x"=35.363000000001946, "y"=260.0, "position"=-35.363031250001946, "velocity"=-50.000000000005684, "acceleration"=-2.842170943040401e-10, "jerk"=-1.7053025658242404e-07, "heading"=-0.0}, {"dt"=0.005, "x"=35.613000000001975, "y"=260.0, "position"=-35.613031250001974, "velocity"=-50.000000000005684, "acceleration"=-0.0, "jerk"=5.6843418860808015e-08, "heading"=-0.0}, {"dt"=0.005, "x"=35.863000000001996, "y"=260.0, "position"=-35.863031250001995, "velocity"=-50.00000000000426, "acceleration"=2.842170943040401e-10, "jerk"=5.6843418860808015e-08, "heading"=-0.0}, {"dt"=0.005, "x"=36.113000000002025, "y"=260.0, "position"=-36.113031250002024, "velocity"=-50.000000000005684, "acceleration"=-2.842170943040401e-10, "jerk"=-1.1368683772161603e-07, "heading"=-0.0}, {"dt"=0.005, "x"=36.36300000000205, "y"=260.0, "position"=-36.36303125000205, "velocity"=-50.000000000005684, "acceleration"=-0.0, "jerk"=5.6843418860808015e-08, "heading"=-0.0}, {"dt"=0.005, "x"=36.61300000000209, "y"=260.0, "position"=-36.61303125000209, "velocity"=-50.000000000007105, "acceleration"=-2.842170943040401e-10, "jerk"=-5.6843418860808015e-08, "heading"=-0.0}, {"dt"=0.005, "x"=36.86300000000211, "y"=260.0, "position"=-36.86303125000211, "velocity"=-50.00000000000426, "acceleration"=5.684341886080801e-10, "jerk"=1.7053025658242404e-07, "heading"=-0.0}, {"dt"=0.005, "x"=37.11300000000214, "y"=260.0, "position"=-37.11303125000214, "velocity"=-50.000000000005684, "acceleration"=-2.842170943040401e-10, "jerk"=-1.7053025658242404e-07, "heading"=-0.0}, {"dt"=0.005, "x"=37.36300000000217, "y"=260.0, "position"=-37.363031250002166, "velocity"=-50.000000000005684, "acceleration"=-0.0, "jerk"=5.6843418860808015e-08, "heading"=-0.0}, {"dt"=0.005, "x"=37.613000000002195, "y"=260.0, "position"=-37.613031250002194, "velocity"=-50.000000000005684, "acceleration"=-0.0, "jerk"=-0.0, "heading"=-0.0}, {"dt"=0.005, "x"=37.863000000002216, "y"=260.0, "position"=-37.863031250002216, "velocity"=-50.00000000000426, "acceleration"=2.842170943040401e-10, "jerk"=5.6843418860808015e-08, "heading"=-0.0}, {"dt"=0.005, "x"=38.113000000002245, "y"=260.0, "position"=-38.113031250002244, "velocity"=-50.000000000005684, "acceleration"=-2.842170943040401e-10, "jerk"=-1.1368683772161603e-07, "heading"=-0.0}, {"dt"=0.005, "x"=38.36300000000227, "y"=260.0, "position"=-38.36303125000227, "velocity"=-50.000000000005684, "acceleration"=-0.0, "jerk"=5.6843418860808015e-08, "heading"=-0.0}, {"dt"=0.005, "x"=38.6130000000023, "y"=260.0, "position"=-38.6130312500023, "velocity"=-50.000000000005684, "acceleration"=-0.0, "jerk"=-0.0, "heading"=-0.0}, {"dt"=0.005, "x"=38.86300000000234, "y"=260.0, "position"=-38.86303125000234, "velocity"=-50.000000000007105, "acceleration"=-2.842170943040401e-10, "jerk"=-5.6843418860808015e-08, "heading"=-0.0}, {"dt"=0.005, "x"=39.11300000000236, "y"=260.0, "position"=-39.11303125000236, "velocity"=-50.00000000000426, "acceleration"=5.684341886080801e-10, "jerk"=1.7053025658242404e-07, "heading"=-0.0}, {"dt"=0.005, "x"=39.36300000000239, "y"=260.0, "position"=-39.363031250002386, "velocity"=-50.000000000005684, "acceleration"=-2.842170943040401e-10, "jerk"=-1.7053025658242404e-07, "heading"=-0.0}, {"dt"=0.005, "x"=39.613000000002415, "y"=260.0, "position"=-39.613031250002415, "velocity"=-50.000000000005684, "acceleration"=-0.0, "jerk"=5.6843418860808015e-08, "heading"=-0.0}, {"dt"=0.005, "x"=39.86300000000244, "y"=260.0, "position"=-39.863031250002436, "velocity"=-50.00000000000426, "acceleration"=2.842170943040401e-10, "jerk"=5.6843418860808015e-08, "heading"=-0.0}, {"dt"=0.005, "x"=40.113000000002465, "y"=260.0, "position"=-40.113031250002464, "velocity"=-50.000000000005684, "acceleration"=-2.842170943040401e-10, "jerk"=-1.1368683772161603e-07, "heading"=-0.0}, {"dt"=0.005, "x"=40.36300000000249, "y"=260.0, "position"=-40.36303125000249, "velocity"=-50.000000000005684, "acceleration"=-0.0, "jerk"=5.6843418860808015e-08, "heading"=-0.0}, {"dt"=0.005, "x"=40.61300000000253, "y"=260.0, "position"=-40.61303125000253, "velocity"=-50.000000000007105, "acceleration"=-2.842170943040401e-10, "jerk"=-5.6843418860808015e-08, "heading"=-0.0}, {"dt"=0.005, "x"=40.86300000000256, "y"=260.0, "position"=-40.86303125000256, "velocity"=-50.000000000005684, "acceleration"=2.842170943040401e-10, "jerk"=1.1368683772161603e-07, "heading"=-0.0}, {"dt"=0.005, "x"=41.11300000000258, "y"=260.0, "position"=-41.11303125000258, "velocity"=-50.00000000000426, "acceleration"=2.842170943040401e-10, "jerk"=-0.0, "heading"=-0.0}, {"dt"=0.005, "x"=41.36300000000261, "y"=260.0, "position"=-41.36303125000261, "velocity"=-50.000000000005684, "acceleration"=-2.842170943040401e-10, "jerk"=-1.1368683772161603e-07, "heading"=-0.0}, {"dt"=0.005, "x"=41.61300000000263, "y"=260.0, "position"=-41.61303125000263, "velocity"=-50.00000000000426, "acceleration"=2.842170943040401e-10, "jerk"=1.1368683772161603e-07, "heading"=-0.0}, {"dt"=0.005, "x"=41.86300000000266, "y"=260.0, "position"=-41.863031250002656, "velocity"=-50.000000000005684, "acceleration"=-2.842170943040401e-10, "jerk"=-1.1368683772161603e-07, "heading"=-0.0}, {"dt"=0.005, "x"=42.11300000000269, "y"=260.0, "position"=-42.11303125000269, "velocity"=-50.000000000007105, "acceleration"=-2.842170943040401e-10, "jerk"=-0.0, "heading"=-0.0}, {"dt"=0.005, "x"=42.36300000000272, "y"=260.0, "position"=-42.36303125000272, "velocity"=-50.000000000005684, "acceleration"=2.842170943040401e-10, "jerk"=1.1368683772161603e-07, "heading"=-0.0}, {"dt"=0.005, "x"=42.61300000000275, "y"=260.0, "position"=-42.61303125000275, "velocity"=-50.000000000005684, "acceleration"=-0.0, "jerk"=-5.6843418860808015e-08, "heading"=-0.0}, {"dt"=0.005, "x"=42.86300000000277, "y"=260.0, "position"=-42.86303125000277, "velocity"=-50.00000000000426, "acceleration"=2.842170943040401e-10, "jerk"=5.6843418860808015e-08, "heading"=-0.0}, {"dt"=0.005, "x"=43.1130000000028, "y"=260.0, "position"=-43.1130312500028, "velocity"=-50.000000000005684, "acceleration"=-2.842170943040401e-10, "jerk"=-1.1368683772161603e-07, "heading"=-0.0}, {"dt"=0.005, "x"=43.36300000000283, "y"=260.0, "position"=-43.36303125000283, "velocity"=-50.000000000005684, "acceleration"=-0.0, "jerk"=5.6843418860808015e-08, "heading"=-0.0}, {"dt"=0.005, "x"=43.61300000000285, "y"=260.0, "position"=-43.61303125000285, "velocity"=-50.00000000000426, "acceleration"=2.842170943040401e-10, "jerk"=5.6843418860808015e-08, "heading"=-0.0}, {"dt"=0.005, "x"=43.86300000000288, "y"=260.0, "position"=-43.86303125000288, "velocity"=-50.000000000005684, "acceleration"=-2.842170943040401e-10, "jerk"=-1.1368683772161603e-07, "heading"=-0.0}, {"dt"=0.005, "x"=44.11300000000291, "y"=260.0, "position"=-44.11303125000291, "velocity"=-50.000000000007105, "acceleration"=-2.842170943040401e-10, "jerk"=-0.0, "heading"=-0.0}, {"dt"=0.005, "x"=44.363000000002934, "y"=260.0, "position"=-44.36303125000293, "velocity"=-50.00000000000426, "acceleration"=5.684341886080801e-10, "jerk"=1.7053025658242404e-07, "heading"=-0.0}, {"dt"=0.005, "x"=44.61300000000297, "y"=260.0, "position"=-44.61303125000297, "velocity"=-50.000000000007105, "acceleration"=-5.684341886080801e-10, "jerk"=-2.2737367544323206e-07, "heading"=-0.0}, {"dt"=0.005, "x"=44.86300000000299, "y"=260.0, "position"=-44.86303125000299, "velocity"=-50.00000000000426, "acceleration"=5.684341886080801e-10, "jerk"=2.2737367544323206e-07, "heading"=-0.0}, {"dt"=0.005, "x"=45.11300000000302, "y"=260.0, "position"=-45.11303125000302, "velocity"=-50.000000000005684, "acceleration"=-2.842170943040401e-10, "jerk"=-1.7053025658242404e-07, "heading"=-0.0}, {"dt"=0.005, "x"=45.36300000000304, "y"=260.0, "position"=-45.36303125000304, "velocity"=-50.00000000000426, "acceleration"=2.842170943040401e-10, "jerk"=1.1368683772161603e-07, "heading"=-0.0}, {"dt"=0.005, "x"=45.61300000000307, "y"=260.0, "position"=-45.61303125000307, "velocity"=-50.000000000005684, "acceleration"=-2.842170943040401e-10, "jerk"=-1.1368683772161603e-07, "heading"=-0.0}, {"dt"=0.005, "x"=45.863000000003105, "y"=260.0, "position"=-45.863031250003104, "velocity"=-50.000000000007105, "acceleration"=-2.842170943040401e-10, "jerk"=-0.0, "heading"=-0.0}, {"dt"=0.005, "x"=46.113000000003126, "y"=260.0, "position"=-46.113031250003125, "velocity"=-50.00000000000426, "acceleration"=5.684341886080801e-10, "jerk"=1.7053025658242404e-07, "heading"=-0.0}, {"dt"=0.005, "x"=46.36300000000316, "y"=260.0, "position"=-46.36303125000316, "velocity"=-50.000000000007105, "acceleration"=-5.684341886080801e-10, "jerk"=-2.2737367544323206e-07, "heading"=-0.0}, {"dt"=0.005, "x"=46.61300000000318, "y"=260.0, "position"=-46.61303125000318, "velocity"=-50.00000000000426, "acceleration"=5.684341886080801e-10, "jerk"=2.2737367544323206e-07, "heading"=-0.0}, {"dt"=0.005, "x"=46.86300000000321, "y"=260.0, "position"=-46.86303125000321, "velocity"=-50.000000000005684, "acceleration"=-2.842170943040401e-10, "jerk"=-1.7053025658242404e-07, "heading"=-0.0}, {"dt"=0.005, "x"=47.11300000000324, "y"=260.0, "position"=-47.11303125000324, "velocity"=-50.000000000005684, "acceleration"=-0.0, "jerk"=5.6843418860808015e-08, "heading"=-0.0}, {"dt"=0.005, "x"=47.36300000000326, "y"=260.0, "position"=-47.36303125000326, "velocity"=-50.00000000000426, "acceleration"=2.842170943040401e-10, "jerk"=5.6843418860808015e-08, "heading"=-0.0}, {"dt"=0.005, "x"=47.61300000000329, "y"=260.0, "position"=-47.61303125000329, "velocity"=-50.000000000005684, "acceleration"=-2.842170943040401e-10, "jerk"=-1.1368683772161603e-07, "heading"=-0.0}, {"dt"=0.005, "x"=47.863000000003325, "y"=260.0, "position"=-47.863031250003324, "velocity"=-50.000000000007105, "acceleration"=-2.842170943040401e-10, "jerk"=-0.0, "heading"=-0.0}, {"dt"=0.005, "x"=48.11300000000335, "y"=260.0, "position"=-48.11303125000335, "velocity"=-50.000000000005684, "acceleration"=2.842170943040401e-10, "jerk"=1.1368683772161603e-07, "heading"=-0.0}, {"dt"=0.005, "x"=48.36300000000338, "y"=260.0, "position"=-48.36303125000338, "velocity"=-50.000000000005684, "acceleration"=-0.0, "jerk"=-5.6843418860808015e-08, "heading"=-0.0}, {"dt"=0.005, "x"=48.6130000000034, "y"=260.0, "position"=-48.6130312500034, "velocity"=-50.00000000000426, "acceleration"=2.842170943040401e-10, "jerk"=5.6843418860808015e-08, "heading"=-0.0}, {"dt"=0.005, "x"=48.86300000000343, "y"=260.0, "position"=-48.86303125000343, "velocity"=-50.000000000005684, "acceleration"=-2.842170943040401e-10, "jerk"=-1.1368683772161603e-07, "heading"=-0.0}, {"dt"=0.005, "x"=49.11300000000346, "y"=260.0, "position"=-49.11303125000346, "velocity"=-50.000000000005684, "acceleration"=-0.0, "jerk"=5.6843418860808015e-08, "heading"=-0.0}, {"dt"=0.005, "x"=49.36300000000348, "y"=260.0, "position"=-49.36303125000348, "velocity"=-50.00000000000426, "acceleration"=2.842170943040401e-10, "jerk"=5.6843418860808015e-08, "heading"=-0.0}, {"dt"=0.005, "x"=49.61300000000352, "y"=260.0, "position"=-49.613031250003516, "velocity"=-50.000000000007105, "acceleration"=-5.684341886080801e-10, "jerk"=-1.7053025658242404e-07, "heading"=-0.0}, {"dt"=0.005, "x"=49.863000000003545, "y"=260.0, "position"=-49.863031250003544, "velocity"=-50.000000000005684, "acceleration"=2.842170943040401e-10, "jerk"=1.7053025658242404e-07, "heading"=-0.0}, {"dt"=0.005, "x"=50.113000000003574, "y"=260.0, "position"=-50.11303125000357, "velocity"=-50.000000000005684, "acceleration"=-0.0, "jerk"=-5.6843418860808015e-08, "heading"=-0.0}, {"dt"=0.005, "x"=50.3630000000036, "y"=260.0, "position"=-50.3630312500036, "velocity"=-50.000000000005684, "acceleration"=-0.0, "jerk"=-0.0, "heading"=-0.0}, {"dt"=0.005, "x"=50.61300000000362, "y"=260.0, "position"=-50.61303125000362, "velocity"=-50.00000000000426, "acceleration"=2.842170943040401e-10, "jerk"=5.6843418860808015e-08, "heading"=-0.0}, {"dt"=0.005, "x"=50.86300000000365, "y"=260.0, "position"=-50.86303125000365, "velocity"=-50.000000000005684, "acceleration"=-2.842170943040401e-10, "jerk"=-1.1368683772161603e-07, "heading"=-0.0}, {"dt"=0.005, "x"=51.11300000000368, "y"=260.0, "position"=-51.11303125000368, "velocity"=-50.000000000005684, "acceleration"=-0.0, "jerk"=5.6843418860808015e-08, "heading"=-0.0}, {"dt"=0.005, "x"=51.3630000000037, "y"=260.0, "position"=-51.3630312500037, "velocity"=-50.00000000000426, "acceleration"=2.842170943040401e-10, "jerk"=5.6843418860808015e-08, "heading"=-0.0}, {"dt"=0.005, "x"=51.613000000003744, "y"=260.0, "position"=-51.61303125000374, "velocity"=-50.00000000000853, "acceleration"=-8.526512829121202e-10, "jerk"=-2.2737367544323206e-07, "heading"=-0.0}, {"dt"=0.005, "x"=51.86300000000376, "y"=260.0, "position"=-51.86303125000376, "velocity"=-50.00000000000284, "acceleration"=1.1368683772161603e-09, "jerk"=3.979039320256561e-07, "heading"=-0.0}, {"dt"=0.005, "x"=52.113000000003794, "y"=260.0, "position"=-52.11303125000379, "velocity"=-50.000000000007105, "acceleration"=-8.526512829121202e-10, "jerk"=-3.979039320256561e-07, "heading"=-0.0}, {"dt"=0.005, "x"=52.36300000000382, "y"=260.0, "position"=-52.36303125000382, "velocity"=-50.000000000005684, "acceleration"=2.842170943040401e-10, "jerk"=2.2737367544323206e-07, "heading"=-0.0}, {"dt"=0.005, "x"=52.613000000003844, "y"=260.0, "position"=-52.61303125000384, "velocity"=-50.00000000000426, "acceleration"=2.842170943040401e-10, "jerk"=-0.0, "heading"=-0.0}, {"dt"=0.005, "x"=52.86300000000387, "y"=260.0, "position"=-52.86303125000387, "velocity"=-50.000000000005684, "acceleration"=-2.842170943040401e-10, "jerk"=-1.1368683772161603e-07, "heading"=-0.0}, {"dt"=0.005, "x"=53.11300000000389, "y"=260.0, "position"=-53.11303125000389, "velocity"=-50.00000000000426, "acceleration"=2.842170943040401e-10, "jerk"=1.1368683772161603e-07, "heading"=-0.0}, {"dt"=0.005, "x"=53.36300000000393, "y"=260.0, "position"=-53.36303125000393, "velocity"=-50.000000000007105, "acceleration"=-5.684341886080801e-10, "jerk"=-1.7053025658242404e-07, "heading"=-0.0}, {"dt"=0.005, "x"=53.61300000000396, "y"=260.0, "position"=-53.61303125000396, "velocity"=-50.000000000005684, "acceleration"=2.842170943040401e-10, "jerk"=1.7053025658242404e-07, "heading"=-0.0}, {"dt"=0.005, "x"=53.863000000003986, "y"=260.0, "position"=-53.863031250003985, "velocity"=-50.000000000005684, "acceleration"=-0.0, "jerk"=-5.6843418860808015e-08, "heading"=-0.0}, {"dt"=0.005, "x"=54.113000000004014, "y"=260.0, "position"=-54.11303125000401, "velocity"=-50.000000000005684, "acceleration"=-0.0, "jerk"=-0.0, "heading"=-0.0}, {"dt"=0.005, "x"=54.363000000004035, "y"=260.0, "position"=-54.363031250004035, "velocity"=-50.00000000000426, "acceleration"=2.842170943040401e-10, "jerk"=5.6843418860808015e-08, "heading"=-0.0}, {"dt"=0.005, "x"=54.613000000004064, "y"=260.0, "position"=-54.61303125000406, "velocity"=-50.000000000005684, "acceleration"=-2.842170943040401e-10, "jerk"=-1.1368683772161603e-07, "heading"=-0.0}, {"dt"=0.005, "x"=54.86300000000409, "y"=260.0, "position"=-54.86303125000409, "velocity"=-50.000000000005684, "acceleration"=-0.0, "jerk"=5.6843418860808015e-08, "heading"=-0.0}, {"dt"=0.005, "x"=55.113000000004114, "y"=260.0, "position"=-55.11303125000411, "velocity"=-50.00000000000426, "acceleration"=2.842170943040401e-10, "jerk"=5.6843418860808015e-08, "heading"=-0.0}, {"dt"=0.005, "x"=55.36300000000415, "y"=260.0, "position"=-55.36303125000415, "velocity"=-50.000000000007105, "acceleration"=-5.684341886080801e-10, "jerk"=-1.7053025658242404e-07, "heading"=-0.0}, {"dt"=0.005, "x"=55.61300000000418, "y"=260.0, "position"=-55.61303125000418, "velocity"=-50.000000000005684, "acceleration"=2.842170943040401e-10, "jerk"=1.7053025658242404e-07, "heading"=-0.0}, {"dt"=0.005, "x"=55.863000000004206, "y"=260.0, "position"=-55.863031250004205, "velocity"=-50.000000000005684, "acceleration"=-0.0, "jerk"=-5.6843418860808015e-08, "heading"=-0.0}, {"dt"=0.005, "x"=56.113000000004234, "y"=260.0, "position"=-56.113031250004234, "velocity"=-50.000000000005684, "acceleration"=-0.0, "jerk"=-0.0, "heading"=-0.0}, {"dt"=0.005, "x"=56.363000000004256, "y"=260.0, "position"=-56.363031250004255, "velocity"=-50.00000000000426, "acceleration"=2.842170943040401e-10, "jerk"=5.6843418860808015e-08, "heading"=-0.0}, {"dt"=0.005, "x"=56.613000000004284, "y"=260.0, "position"=-56.61303125000428, "velocity"=-50.000000000005684, "acceleration"=-2.842170943040401e-10, "jerk"=-1.1368683772161603e-07, "heading"=-0.0}, {"dt"=0.005, "x"=56.863000000004305, "y"=260.0, "position"=-56.863031250004305, "velocity"=-50.00000000000426, "acceleration"=2.842170943040401e-10, "jerk"=1.1368683772161603e-07, "heading"=-0.0}, {"dt"=0.005, "x"=57.11300000000434, "y"=260.0, "position"=-57.11303125000434, "velocity"=-50.000000000007105, "acceleration"=-5.684341886080801e-10, "jerk"=-1.7053025658242404e-07, "heading"=-0.0}, {"dt"=0.005, "x"=57.36300000000438, "y"=260.0, "position"=-57.363031250004376, "velocity"=-50.000000000007105, "acceleration"=-0.0, "jerk"=1.1368683772161603e-07, "heading"=-0.0}, {"dt"=0.005, "x"=57.6130000000044, "y"=260.0, "position"=-57.6130312500044, "velocity"=-50.00000000000426, "acceleration"=5.684341886080801e-10, "jerk"=1.1368683772161603e-07, "heading"=-0.0}, {"dt"=0.005, "x"=57.863000000004426, "y"=260.0, "position"=-57.863031250004425, "velocity"=-50.000000000005684, "acceleration"=-2.842170943040401e-10, "jerk"=-1.7053025658242404e-07, "heading"=-0.0}, {"dt"=0.005, "x"=58.11300000000445, "y"=260.0, "position"=-58.11303125000445, "velocity"=-50.00000000000426, "acceleration"=2.842170943040401e-10, "jerk"=1.1368683772161603e-07, "heading"=-0.0}, {"dt"=0.005, "x"=58.363000000004476, "y"=260.0, "position"=-58.363031250004475, "velocity"=-50.000000000005684, "acceleration"=-2.842170943040401e-10, "jerk"=-1.1368683772161603e-07, "heading"=-0.0}, {"dt"=0.005, "x"=58.613000000004504, "y"=260.0, "position"=-58.613031250004504, "velocity"=-50.000000000005684, "acceleration"=-0.0, "jerk"=5.6843418860808015e-08, "heading"=-0.0}, {"dt"=0.005, "x"=58.863000000004526, "y"=260.0, "position"=-58.863031250004525, "velocity"=-50.00000000000426, "acceleration"=2.842170943040401e-10, "jerk"=5.6843418860808015e-08, "heading"=-0.0}, {"dt"=0.005, "x"=59.11300000000457, "y"=260.0, "position"=-59.11303125000457, "velocity"=-50.00000000000853, "acceleration"=-8.526512829121202e-10, "jerk"=-2.2737367544323206e-07, "heading"=-0.0}, {"dt"=0.005, "x"=59.36300000000459, "y"=260.0, "position"=-59.36303125000459, "velocity"=-50.00000000000426, "acceleration"=8.526512829121202e-10, "jerk"=3.410605131648481e-07, "heading"=-0.0}, {"dt"=0.005, "x"=59.61300000000462, "y"=260.0, "position"=-59.61303125000462, "velocity"=-50.000000000005684, "acceleration"=-2.842170943040401e-10, "jerk"=-2.2737367544323206e-07, "heading"=-0.0}, {"dt"=0.005, "x"=59.86300000000465, "y"=260.0, "position"=-59.863031250004646, "velocity"=-50.000000000005684, "acceleration"=-0.0, "jerk"=5.6843418860808015e-08, "heading"=-0.0}, {"dt"=0.005, "x"=60.11300000000467, "y"=260.0, "position"=-60.11303125000467, "velocity"=-50.00000000000426, "acceleration"=2.842170943040401e-10, "jerk"=5.6843418860808015e-08, "heading"=-0.0}, {"dt"=0.005, "x"=60.363000000004696, "y"=260.0, "position"=-60.363031250004695, "velocity"=-50.000000000005684, "acceleration"=-2.842170943040401e-10, "jerk"=-1.1368683772161603e-07, "heading"=-0.0}, {"dt"=0.005, "x"=60.613000000004725, "y"=260.0, "position"=-60.613031250004724, "velocity"=-50.000000000005684, "acceleration"=-0.0, "jerk"=5.6843418860808015e-08, "heading"=-0.0}, {"dt"=0.005, "x"=60.863000000004746, "y"=260.0, "position"=-60.863031250004745, "velocity"=-50.00000000000426, "acceleration"=2.842170943040401e-10, "jerk"=5.6843418860808015e-08, "heading"=-0.0}, {"dt"=0.005, "x"=61.113000000004774, "y"=260.0, "position"=-61.113031250004774, "velocity"=-50.000000000005684, "acceleration"=-2.842170943040401e-10, "jerk"=-1.1368683772161603e-07, "heading"=-0.0}, {"dt"=0.005, "x"=61.3630000000048, "y"=260.0, "position"=-61.3630312500048, "velocity"=-50.000000000005684, "acceleration"=-0.0, "jerk"=5.6843418860808015e-08, "heading"=-0.0}, {"dt"=0.005, "x"=61.613000000004824, "y"=260.0, "position"=-61.61303125000482, "velocity"=-50.00000000000426, "acceleration"=2.842170943040401e-10, "jerk"=5.6843418860808015e-08, "heading"=-0.0}, {"dt"=0.005, "x"=61.86300000000487, "y"=260.0, "position"=-61.863031250004866, "velocity"=-50.00000000000853, "acceleration"=-8.526512829121202e-10, "jerk"=-2.2737367544323206e-07, "heading"=-0.0}, {"dt"=0.005, "x"=62.1130000000049, "y"=260.0, "position"=-62.1130312500049, "velocity"=-50.000000000007105, "acceleration"=2.842170943040401e-10, "jerk"=2.2737367544323206e-07, "heading"=-0.0}, {"dt"=0.005, "x"=62.36300000000493, "y"=260.0, "position"=-62.36303125000493, "velocity"=-50.000000000005684, "acceleration"=2.842170943040401e-10, "jerk"=-0.0, "heading"=-0.0}, {"dt"=0.005, "x"=62.61300000000495, "y"=260.0, "position"=-62.61303125000495, "velocity"=-50.00000000000426, "acceleration"=2.842170943040401e-10, "jerk"=-0.0, "heading"=-0.0}, {"dt"=0.005, "x"=62.86300000000498, "y"=260.0, "position"=-62.86303125000498, "velocity"=-50.000000000005684, "acceleration"=-2.842170943040401e-10, "jerk"=-1.1368683772161603e-07, "heading"=-0.0}, {"dt"=0.005, "x"=63.11300000000501, "y"=260.0, "position"=-63.11303125000501, "velocity"=-50.000000000005684, "acceleration"=-0.0, "jerk"=5.6843418860808015e-08, "heading"=-0.0}, {"dt"=0.005, "x"=63.36300000000503, "y"=260.0, "position"=-63.36303125000503, "velocity"=-50.00000000000426, "acceleration"=2.842170943040401e-10, "jerk"=5.6843418860808015e-08, "heading"=-0.0}, {"dt"=0.005, "x"=63.61300000000506, "y"=260.0, "position"=-63.61303125000506, "velocity"=-50.000000000005684, "acceleration"=-2.842170943040401e-10, "jerk"=-1.1368683772161603e-07, "heading"=-0.0}, {"dt"=0.005, "x"=63.86300000000509, "y"=260.0, "position"=-63.863031250005086, "velocity"=-50.000000000005684, "acceleration"=-0.0, "jerk"=5.6843418860808015e-08, "heading"=-0.0}, {"dt"=0.005, "x"=64.11300000000512, "y"=260.0, "position"=-64.11303125000512, "velocity"=-50.000000000005684, "acceleration"=-0.0, "jerk"=-0.0, "heading"=-0.0}, {"dt"=0.005, "x"=64.36300000000513, "y"=260.0, "position"=-64.36303125000514, "velocity"=-50.00000000000284, "acceleration"=5.684341886080801e-10, "jerk"=1.1368683772161603e-07, "heading"=-0.0}, {"dt"=0.005, "x"=64.61300000000516, "y"=260.0, "position"=-64.61303125000516, "velocity"=-50.000000000005684, "acceleration"=-5.684341886080801e-10, "jerk"=-2.2737367544323206e-07, "heading"=-0.0}, {"dt"=0.005, "x"=64.86300000000519, "y"=260.0, "position"=-64.86303125000519, "velocity"=-50.000000000005684, "acceleration"=-0.0, "jerk"=1.1368683772161603e-07, "heading"=-0.0}, {"dt"=0.005, "x"=65.11300000000521, "y"=260.0, "position"=-65.11303125000522, "velocity"=-50.000000000005684, "acceleration"=-0.0, "jerk"=-0.0, "heading"=-0.0}, {"dt"=0.005, "x"=65.36300000000524, "y"=260.0, "position"=-65.36303125000525, "velocity"=-50.000000000005684, "acceleration"=-0.0, "jerk"=-0.0, "heading"=-0.0}, {"dt"=0.005, "x"=65.61300000000526, "y"=260.0, "position"=-65.61303125000526, "velocity"=-50.00000000000284, "acceleration"=5.684341886080801e-10, "jerk"=1.1368683772161603e-07, "heading"=-0.0}, {"dt"=0.005, "x"=65.8630000000053, "y"=260.0, "position"=-65.8630312500053, "velocity"=-50.00000000000853, "acceleration"=-1.1368683772161603e-09, "jerk"=-3.410605131648481e-07, "heading"=-0.0}, {"dt"=0.005, "x"=66.11300000000533, "y"=260.0, "position"=-66.11303125000533, "velocity"=-50.000000000005684, "acceleration"=5.684341886080801e-10, "jerk"=3.410605131648481e-07, "heading"=-0.0}, {"dt"=0.005, "x"=66.36300000000536, "y"=260.0, "position"=-66.36303125000536, "velocity"=-50.000000000005684, "acceleration"=-0.0, "jerk"=-1.1368683772161603e-07, "heading"=-0.0}, {"dt"=0.005, "x"=66.61300000000539, "y"=260.0, "position"=-66.61303125000539, "velocity"=-50.000000000005684, "acceleration"=-0.0, "jerk"=-0.0, "heading"=-0.0}, {"dt"=0.005, "x"=66.8630000000054, "y"=260.0, "position"=-66.8630312500054, "velocity"=-50.00000000000284, "acceleration"=5.684341886080801e-10, "jerk"=1.1368683772161603e-07, "heading"=-0.0}, {"dt"=0.005, "x"=67.11300000000543, "y"=260.0, "position"=-67.11303125000543, "velocity"=-50.000000000005684, "acceleration"=-5.684341886080801e-10, "jerk"=-2.2737367544323206e-07, "heading"=-0.0}, {"dt"=0.005, "x"=67.36300000000546, "y"=260.0, "position"=-67.36303125000546, "velocity"=-50.000000000005684, "acceleration"=-0.0, "jerk"=1.1368683772161603e-07, "heading"=-0.0}, {"dt"=0.005, "x"=67.6130000000055, "y"=260.0, "position"=-67.6130312500055, "velocity"=-50.00000000000853, "acceleration"=-5.684341886080801e-10, "jerk"=-1.1368683772161603e-07, "heading"=-0.0}, {"dt"=0.005, "x"=67.86300000000553, "y"=260.0, "position"=-67.86303125000553, "velocity"=-50.000000000005684, "acceleration"=5.684341886080801e-10, "jerk"=2.2737367544323206e-07, "heading"=-0.0}, {"dt"=0.005, "x"=68.11300000000554, "y"=260.0, "position"=-68.11303125000555, "velocity"=-50.00000000000284, "acceleration"=5.684341886080801e-10, "jerk"=-0.0, "heading"=-0.0}, {"dt"=0.005, "x"=68.36300000000557, "y"=260.0, "position"=-68.36303125000558, "velocity"=-50.000000000005684, "acceleration"=-5.684341886080801e-10, "jerk"=-2.2737367544323206e-07, "heading"=-0.0}, {"dt"=0.005, "x"=68.6130000000056, "y"=260.0, "position"=-68.6130312500056, "velocity"=-50.000000000005684, "acceleration"=-0.0, "jerk"=1.1368683772161603e-07, "heading"=-0.0}, {"dt"=0.005, "x"=68.86300000000563, "y"=260.0, "position"=-68.86303125000563, "velocity"=-50.000000000005684, "acceleration"=-0.0, "jerk"=-0.0, "heading"=-0.0}, {"dt"=0.005, "x"=69.11300000000566, "y"=260.0, "position"=-69.11303125000566, "velocity"=-50.000000000005684, "acceleration"=-0.0, "jerk"=-0.0, "heading"=-0.0}, {"dt"=0.005, "x"=69.36300000000568, "y"=260.0, "position"=-69.36303125000569, "velocity"=-50.000000000005684, "acceleration"=-0.0, "jerk"=-0.0, "heading"=-0.0}, {"dt"=0.005, "x"=69.61300000000571, "y"=260.0, "position"=-69.61303125000572, "velocity"=-50.000000000005684, "acceleration"=-0.0, "jerk"=-0.0, "heading"=-0.0}, {"dt"=0.005, "x"=69.86300000000574, "y"=260.0, "position"=-69.86303125000575, "velocity"=-50.000000000005684, "acceleration"=-0.0, "jerk"=-0.0, "heading"=-0.0}, {"dt"=0.005, "x"=70.11300000000577, "y"=260.0, "position"=-70.11303125000578, "velocity"=-50.000000000005684, "acceleration"=-0.0, "jerk"=-0.0, "heading"=-0.0}, {"dt"=0.005, "x"=70.3630000000058, "y"=260.0, "position"=-70.3630312500058, "velocity"=-50.000000000005684, "acceleration"=-0.0, "jerk"=-0.0, "heading"=-0.0}, {"dt"=0.005, "x"=70.61300000000583, "y"=260.0, "position"=-70.61303125000583, "velocity"=-50.000000000005684, "acceleration"=-0.0, "jerk"=-0.0, "heading"=-0.0}, {"dt"=0.005, "x"=70.86300000000584, "y"=260.0, "position"=-70.86303125000585, "velocity"=-50.00000000000284, "acceleration"=5.684341886080801e-10, "jerk"=1.1368683772161603e-07, "heading"=-0.0}, {"dt"=0.005, "x"=71.11300000000587, "y"=260.0, "position"=-71.11303125000587, "velocity"=-50.000000000005684, "acceleration"=-5.684341886080801e-10, "jerk"=-2.2737367544323206e-07, "heading"=-0.0}, {"dt"=0.005, "x"=71.36300000000591, "y"=260.0, "position"=-71.36303125000592, "velocity"=-50.00000000000853, "acceleration"=-5.684341886080801e-10, "jerk"=-0.0, "heading"=-0.0}, {"dt"=0.005, "x"=71.61300000000594, "y"=260.0, "position"=-71.61303125000595, "velocity"=-50.000000000005684, "acceleration"=5.684341886080801e-10, "jerk"=2.2737367544323206e-07, "heading"=-0.0}, {"dt"=0.005, "x"=71.86300000000597, "y"=260.0, "position"=-71.86303125000597, "velocity"=-50.000000000005684, "acceleration"=-0.0, "jerk"=-1.1368683772161603e-07, "heading"=-0.0}, {"dt"=0.005, "x"=72.11300000000598, "y"=260.0, "position"=-72.11303125000599, "velocity"=-50.00000000000284, "acceleration"=5.684341886080801e-10, "jerk"=1.1368683772161603e-07, "heading"=-0.0}, {"dt"=0.005, "x"=72.36300000000601, "y"=260.0, "position"=-72.36303125000602, "velocity"=-50.000000000005684, "acceleration"=-5.684341886080801e-10, "jerk"=-2.2737367544323206e-07, "heading"=-0.0}, {"dt"=0.005, "x"=72.61300000000604, "y"=260.0, "position"=-72.61303125000605, "velocity"=-50.000000000005684, "acceleration"=-0.0, "jerk"=1.1368683772161603e-07, "heading"=-0.0}, {"dt"=0.005, "x"=72.86300000000607, "y"=260.0, "position"=-72.86303125000607, "velocity"=-50.000000000005684, "acceleration"=-0.0, "jerk"=-0.0, "heading"=-0.0}, {"dt"=0.005, "x"=73.1130000000061, "y"=260.0, "position"=-73.1130312500061, "velocity"=-50.000000000005684, "acceleration"=-0.0, "jerk"=-0.0, "heading"=-0.0}, {"dt"=0.005, "x"=73.36300000000612, "y"=260.0, "position"=-73.36303125000613, "velocity"=-50.000000000005684, "acceleration"=-0.0, "jerk"=-0.0, "heading"=-0.0}, {"dt"=0.005, "x"=73.61300000000615, "y"=260.0, "position"=-73.61303125000616, "velocity"=-50.000000000005684, "acceleration"=-0.0, "jerk"=-0.0, "heading"=-0.0}, {"dt"=0.005, "x"=73.86300000000618, "y"=260.0, "position"=-73.86303125000619, "velocity"=-50.000000000005684, "acceleration"=-0.0, "jerk"=-0.0, "heading"=-0.0}, {"dt"=0.005, "x"=74.11300000000621, "y"=260.0, "position"=-74.11303125000622, "velocity"=-50.000000000005684, "acceleration"=-0.0, "jerk"=-0.0, "heading"=-0.0}, {"dt"=0.005, "x"=74.36300000000624, "y"=260.0, "position"=-74.36303125000624, "velocity"=-50.000000000005684, "acceleration"=-0.0, "jerk"=-0.0, "heading"=-0.0}, {"dt"=0.005, "x"=74.61300000000625, "y"=260.0, "position"=-74.61303125000626, "velocity"=-50.00000000000284, "acceleration"=5.684341886080801e-10, "jerk"=1.1368683772161603e-07, "heading"=-0.0}, {"dt"=0.005, "x"=74.86300000000628, "y"=260.0, "position"=-74.86303125000629, "velocity"=-50.000000000005684, "acceleration"=-5.684341886080801e-10, "jerk"=-2.2737367544323206e-07, "heading"=-0.0}, {"dt"=0.005, "x"=75.11300000000632, "y"=260.0, "position"=-75.11303125000633, "velocity"=-50.00000000000853, "acceleration"=-5.684341886080801e-10, "jerk"=-0.0, "heading"=-0.0}, {"dt"=0.005, "x"=75.36300000000635, "y"=260.0, "position"=-75.36303125000636, "velocity"=-50.000000000005684, "acceleration"=5.684341886080801e-10, "jerk"=2.2737367544323206e-07, "heading"=-0.0}, {"dt"=0.005, "x"=75.61300000000638, "y"=260.0, "position"=-75.61303125000639, "velocity"=-50.000000000005684, "acceleration"=-0.0, "jerk"=-1.1368683772161603e-07, "heading"=-0.0}, {"dt"=0.005, "x"=75.8630000000064, "y"=260.0, "position"=-75.8630312500064, "velocity"=-50.00000000000284, "acceleration"=5.684341886080801e-10, "jerk"=1.1368683772161603e-07, "heading"=-0.0}, {"dt"=0.005, "x"=76.11300000000642, "y"=260.0, "position"=-76.11303125000643, "velocity"=-50.000000000005684, "acceleration"=-5.684341886080801e-10, "jerk"=-2.2737367544323206e-07, "heading"=-0.0}, {"dt"=0.005, "x"=76.36300000000645, "y"=260.0, "position"=-76.36303125000646, "velocity"=-50.000000000005684, "acceleration"=-0.0, "jerk"=1.1368683772161603e-07, "heading"=-0.0}, {"dt"=0.005, "x"=76.61300000000648, "y"=260.0, "position"=-76.61303125000649, "velocity"=-50.000000000005684, "acceleration"=-0.0, "jerk"=-0.0, "heading"=-0.0}, {"dt"=0.005, "x"=76.86300000000651, "y"=260.0, "position"=-76.86303125000651, "velocity"=-50.000000000005684, "acceleration"=-0.0, "jerk"=-0.0, "heading"=-0.0}, {"dt"=0.005, "x"=77.11300000000654, "y"=260.0, "position"=-77.11303125000654, "velocity"=-50.000000000005684, "acceleration"=-0.0, "jerk"=-0.0, "heading"=-0.0}, {"dt"=0.005, "x"=77.36300000000656, "y"=260.0, "position"=-77.36303125000657, "velocity"=-50.000000000005684, "acceleration"=-0.0, "jerk"=-0.0, "heading"=-0.0}, {"dt"=0.005, "x"=77.6130000000066, "y"=260.0, "position"=-77.6130312500066, "velocity"=-50.000000000005684, "acceleration"=-0.0, "jerk"=-0.0, "heading"=-0.0}, {"dt"=0.005, "x"=77.86300000000662, "y"=260.0, "position"=-77.86303125000663, "velocity"=-50.000000000005684, "acceleration"=-0.0, "jerk"=-0.0, "heading"=-0.0}, {"dt"=0.005, "x"=78.11300000000665, "y"=260.0, "position"=-78.11303125000666, "velocity"=-50.000000000005684, "acceleration"=-0.0, "jerk"=-0.0, "heading"=-0.0}, {"dt"=0.005, "x"=78.36300000000666, "y"=260.0, "position"=-78.36303125000667, "velocity"=-50.00000000000284, "acceleration"=5.684341886080801e-10, "jerk"=1.1368683772161603e-07, "heading"=-0.0}, {"dt"=0.005, "x"=78.61300000000669, "y"=260.0, "position"=-78.6130312500067, "velocity"=-50.000000000005684, "acceleration"=-5.684341886080801e-10, "jerk"=-2.2737367544323206e-07, "heading"=-0.0}, {"dt"=0.005, "x"=78.86300000000674, "y"=260.0, "position"=-78.86303125000674, "velocity"=-50.00000000000853, "acceleration"=-5.684341886080801e-10, "jerk"=-0.0, "heading"=-0.0}, {"dt"=0.005, "x"=79.11300000000676, "y"=260.0, "position"=-79.11303125000677, "velocity"=-50.000000000005684, "acceleration"=5.684341886080801e-10, "jerk"=2.2737367544323206e-07, "heading"=-0.0}, {"dt"=0.005, "x"=79.36300000000679, "y"=260.0, "position"=-79.3630312500068, "velocity"=-50.000000000005684, "acceleration"=-0.0, "jerk"=-1.1368683772161603e-07, "heading"=-0.0}, {"dt"=0.005, "x"=79.6130000000068, "y"=260.0, "position"=-79.61303125000681, "velocity"=-50.00000000000284, "acceleration"=5.684341886080801e-10, "jerk"=1.1368683772161603e-07, "heading"=-0.0}, {"dt"=0.005, "x"=79.86300000000683, "y"=260.0, "position"=-79.86303125000684, "velocity"=-50.000000000005684, "acceleration"=-5.684341886080801e-10, "jerk"=-2.2737367544323206e-07, "heading"=-0.0}, {"dt"=0.005, "x"=80.11300000000686, "y"=260.0, "position"=-80.11303125000687, "velocity"=-50.000000000005684, "acceleration"=-0.0, "jerk"=1.1368683772161603e-07, "heading"=-0.0}, {"dt"=0.005, "x"=80.36300000000689, "y"=260.0, "position"=-80.3630312500069, "velocity"=-50.000000000005684, "acceleration"=-0.0, "jerk"=-0.0, "heading"=-0.0}, {"dt"=0.005, "x"=80.61300000000692, "y"=260.0, "position"=-80.61303125000693, "velocity"=-50.000000000005684, "acceleration"=-0.0, "jerk"=-0.0, "heading"=-0.0}, {"dt"=0.005, "x"=80.86300000000695, "y"=260.0, "position"=-80.86303125000696, "velocity"=-50.000000000005684, "acceleration"=-0.0, "jerk"=-0.0, "heading"=-0.0}, {"dt"=0.005, "x"=81.11300000000698, "y"=260.0, "position"=-81.11303125000698, "velocity"=-50.000000000005684, "acceleration"=-0.0, "jerk"=-0.0, "heading"=-0.0}, {"dt"=0.005, "x"=81.363000000007, "y"=260.0, "position"=-81.36303125000701, "velocity"=-50.000000000005684, "acceleration"=-0.0, "jerk"=-0.0, "heading"=-0.0}, {"dt"=0.005, "x"=81.61300000000703, "y"=260.0, "position"=-81.61303125000704, "velocity"=-50.000000000005684, "acceleration"=-0.0, "jerk"=-0.0, "heading"=-0.0}, {"dt"=0.005, "x"=81.86300000000706, "y"=260.0, "position"=-81.86303125000707, "velocity"=-50.000000000005684, "acceleration"=-0.0, "jerk"=-0.0, "heading"=-0.0}, {"dt"=0.005, "x"=82.11300000000708, "y"=260.0, "position"=-82.11303125000708, "velocity"=-50.00000000000284, "acceleration"=5.684341886080801e-10, "jerk"=1.1368683772161603e-07, "heading"=-0.0}, {"dt"=0.005, "x"=82.3630000000071, "y"=260.0, "position"=-82.36303125000711, "velocity"=-50.000000000005684, "acceleration"=-5.684341886080801e-10, "jerk"=-2.2737367544323206e-07, "heading"=-0.0}, {"dt"=0.005, "x"=82.61300000000715, "y"=260.0, "position"=-82.61303125000715, "velocity"=-50.00000000000853, "acceleration"=-5.684341886080801e-10, "jerk"=-0.0, "heading"=-0.0}, {"dt"=0.005, "x"=82.86300000000718, "y"=260.0, "position"=-82.86303125000718, "velocity"=-50.000000000005684, "acceleration"=5.684341886080801e-10, "jerk"=2.2737367544323206e-07, "heading"=-0.0}, {"dt"=0.005, "x"=83.1130000000072, "y"=260.0, "position"=-83.11303125000721, "velocity"=-50.000000000005684, "acceleration"=-0.0, "jerk"=-1.1368683772161603e-07, "heading"=-0.0}, {"dt"=0.005, "x"=83.36300000000722, "y"=260.0, "position"=-83.36303125000723, "velocity"=-50.00000000000284, "acceleration"=5.684341886080801e-10, "jerk"=1.1368683772161603e-07, "heading"=-0.0}, {"dt"=0.005, "x"=83.61300000000725, "y"=260.0, "position"=-83.61303125000725, "velocity"=-50.000000000005684, "acceleration"=-5.684341886080801e-10, "jerk"=-2.2737367544323206e-07, "heading"=-0.0}, {"dt"=0.005, "x"=83.86300000000728, "y"=260.0, "position"=-83.86303125000728, "velocity"=-50.000000000005684, "acceleration"=-0.0, "jerk"=1.1368683772161603e-07, "heading"=-0.0}, {"dt"=0.005, "x"=84.1130000000073, "y"=260.0, "position"=-84.11303125000731, "velocity"=-50.000000000005684, "acceleration"=-0.0, "jerk"=-0.0, "heading"=-0.0}, {"dt"=0.005, "x"=84.36300000000733, "y"=260.0, "position"=-84.36303125000734, "velocity"=-50.000000000005684, "acceleration"=-0.0, "jerk"=-0.0, "heading"=-0.0}, {"dt"=0.005, "x"=84.61300000000736, "y"=260.0, "position"=-84.61303125000737, "velocity"=-50.000000000005684, "acceleration"=-0.0, "jerk"=-0.0, "heading"=-0.0}, {"dt"=0.005, "x"=84.86300000000739, "y"=260.0, "position"=-84.8630312500074, "velocity"=-50.000000000005684, "acceleration"=-0.0, "jerk"=-0.0, "heading"=-0.0}, {"dt"=0.005, "x"=85.11300000000742, "y"=260.0, "position"=-85.11303125000742, "velocity"=-50.000000000005684, "acceleration"=-0.0, "jerk"=-0.0, "heading"=-0.0}, {"dt"=0.005, "x"=85.36300000000745, "y"=260.0, "position"=-85.36303125000745, "velocity"=-50.000000000005684, "acceleration"=-0.0, "jerk"=-0.0, "heading"=-0.0}, {"dt"=0.005, "x"=85.61300000000747, "y"=260.0, "position"=-85.61303125000748, "velocity"=-50.000000000005684, "acceleration"=-0.0, "jerk"=-0.0, "heading"=-0.0}, {"dt"=0.005, "x"=85.8630000000075, "y"=260.0, "position"=-85.86303125000751, "velocity"=-50.000000000005684, "acceleration"=-0.0, "jerk"=-0.0, "heading"=-0.0}, {"dt"=0.005, "x"=86.11300000000752, "y"=260.0, "position"=-86.11303125000752, "velocity"=-50.00000000000284, "acceleration"=5.684341886080801e-10, "jerk"=1.1368683772161603e-07, "heading"=-0.0}, {"dt"=0.005, "x"=86.36300000000756, "y"=260.0, "position"=-86.36303125000757, "velocity"=-50.00000000000853, "acceleration"=-1.1368683772161603e-09, "jerk"=-3.410605131648481e-07, "heading"=-0.0}, {"dt"=0.005, "x"=86.61300000000759, "y"=260.0, "position"=-86.6130312500076, "velocity"=-50.000000000005684, "acceleration"=5.684341886080801e-10, "jerk"=3.410605131648481e-07, "heading"=-0.0}, {"dt"=0.005, "x"=86.86300000000762, "y"=260.0, "position"=-86.86303125000762, "velocity"=-50.000000000005684, "acceleration"=-0.0, "jerk"=-1.1368683772161603e-07, "heading"=-0.0}, {"dt"=0.005, "x"=87.11300000000764, "y"=260.0, "position"=-87.11303125000765, "velocity"=-50.000000000005684, "acceleration"=-0.0, "jerk"=-0.0, "heading"=-0.0}, {"dt"=0.005, "x"=87.36300000000766, "y"=260.0, "position"=-87.36303125000767, "velocity"=-50.00000000000284, "acceleration"=5.684341886080801e-10, "jerk"=1.1368683772161603e-07, "heading"=-0.0}, {"dt"=0.005, "x"=87.61300000000769, "y"=260.0, "position"=-87.6130312500077, "velocity"=-50.000000000005684, "acceleration"=-5.684341886080801e-10, "jerk"=-2.2737367544323206e-07, "heading"=-0.0}, {"dt"=0.005, "x"=87.86300000000772, "y"=260.0, "position"=-87.86303125000772, "velocity"=-50.000000000005684, "acceleration"=-0.0, "jerk"=1.1368683772161603e-07, "heading"=-0.0}, {"dt"=0.005, "x"=88.11300000000774, "y"=260.0, "position"=-88.11303125000775, "velocity"=-50.000000000005684, "acceleration"=-0.0, "jerk"=-0.0, "heading"=-0.0}, {"dt"=0.005, "x"=88.36300000000779, "y"=260.0, "position"=-88.3630312500078, "velocity"=-50.00000000000853, "acceleration"=-5.684341886080801e-10, "jerk"=-1.1368683772161603e-07, "heading"=-0.0}, {"dt"=0.005, "x"=88.6130000000078, "y"=260.0, "position"=-88.61303125000781, "velocity"=-50.00000000000284, "acceleration"=1.1368683772161603e-09, "jerk"=3.410605131648481e-07, "heading"=-0.0}, {"dt"=0.005, "x"=88.86300000000783, "y"=260.0, "position"=-88.86303125000784, "velocity"=-50.000000000005684, "acceleration"=-5.684341886080801e-10, "jerk"=-3.410605131648481e-07, "heading"=-0.0}, {"dt"=0.005, "x"=89.11300000000786, "y"=260.0, "position"=-89.11303125000786, "velocity"=-50.000000000005684, "acceleration"=-0.0, "jerk"=1.1368683772161603e-07, "heading"=-0.0}, {"dt"=0.005, "x"=89.36300000000789, "y"=260.0, "position"=-89.3630312500079, "velocity"=-50.000000000005684, "acceleration"=-0.0, "jerk"=-0.0, "heading"=-0.0}, {"dt"=0.005, "x"=89.61300000000791, "y"=260.0, "position"=-89.61303125000792, "velocity"=-50.000000000005684, "acceleration"=-0.0, "jerk"=-0.0, "heading"=-0.0}, {"dt"=0.005, "x"=89.86300000000793, "y"=260.0, "position"=-89.86303125000794, "velocity"=-50.00000000000284, "acceleration"=5.684341886080801e-10, "jerk"=1.1368683772161603e-07, "heading"=-0.0}, {"dt"=0.005, "x"=90.11300000000797, "y"=260.0, "position"=-90.11303125000798, "velocity"=-50.00000000000853, "acceleration"=-1.1368683772161603e-09, "jerk"=-3.410605131648481e-07, "heading"=-0.0}, {"dt"=0.005, "x"=90.363000000008, "y"=260.0, "position"=-90.363031250008, "velocity"=-50.000000000005684, "acceleration"=5.684341886080801e-10, "jerk"=3.410605131648481e-07, "heading"=-0.0}, {"dt"=0.005, "x"=90.61300000000803, "y"=260.0, "position"=-90.61303125000804, "velocity"=-50.000000000005684, "acceleration"=-0.0, "jerk"=-1.1368683772161603e-07, "heading"=-0.0}, {"dt"=0.005, "x"=90.86300000000806, "y"=260.0, "position"=-90.86303125000806, "velocity"=-50.000000000005684, "acceleration"=-0.0, "jerk"=-0.0, "heading"=-0.0}, {"dt"=0.005, "x"=91.11300000000807, "y"=260.0, "position"=-91.11303125000808, "velocity"=-50.00000000000284, "acceleration"=5.684341886080801e-10, "jerk"=1.1368683772161603e-07, "heading"=-0.0}, {"dt"=0.005, "x"=91.3630000000081, "y"=260.0, "position"=-91.3630312500081, "velocity"=-50.000000000005684, "acceleration"=-5.684341886080801e-10, "jerk"=-2.2737367544323206e-07, "heading"=-0.0}, {"dt"=0.005, "x"=91.61300000000813, "y"=260.0, "position"=-91.61303125000813, "velocity"=-50.000000000005684, "acceleration"=-0.0, "jerk"=1.1368683772161603e-07, "heading"=-0.0}, {"dt"=0.005, "x"=91.86300000000816, "y"=260.0, "position"=-91.86303125000816, "velocity"=-50.000000000005684, "acceleration"=-0.0, "jerk"=-0.0, "heading"=-0.0}, {"dt"=0.005, "x"=92.1130000000082, "y"=260.0, "position"=-92.1130312500082, "velocity"=-50.00000000000853, "acceleration"=-5.684341886080801e-10, "jerk"=-1.1368683772161603e-07, "heading"=-0.0}, {"dt"=0.005, "x"=92.36300000000821, "y"=260.0, "position"=-92.36303125000822, "velocity"=-50.00000000000284, "acceleration"=1.1368683772161603e-09, "jerk"=3.410605131648481e-07, "heading"=-0.0}, {"dt"=0.005, "x"=92.61300000000824, "y"=260.0, "position"=-92.61303125000825, "velocity"=-50.000000000005684, "acceleration"=-5.684341886080801e-10, "jerk"=-3.410605131648481e-07, "heading"=-0.0}, {"dt"=0.005, "x"=92.86297025000827, "y"=260.0, "position"=-92.86300150000828, "velocity"=-49.994050000006496, "acceleration"=1.1899999998377098, "jerk"=238.0000000812288, "heading"=-0.0}, {"dt"=0.005, "x"=93.1128497500083, "y"=260.0, "position"=-93.1128810000083, "velocity"=-49.975900000004, "acceleration"=3.6300000004985122, "jerk"=488.0000001321605, "heading"=-0.0}, {"dt"=0.005, "x"=93.36257600000832, "y"=260.0, "position"=-93.36260725000832, "velocity"=-49.94525000000465, "acceleration"=6.129999999870961, "jerk"=499.99999987448973, "heading"=-0.0}, {"dt"=0.005, "x"=93.61208650000833, "y"=260.0, "position"=-93.61211775000834, "velocity"=-49.90210000000275, "acceleration"=8.630000000380278, "jerk"=500.0000001018634, "heading"=-0.0}, {"dt"=0.005, "x"=93.86131875000834, "y"=260.0, "position"=-93.86135000000834, "velocity"=-49.84645000000114, "acceleration"=11.13000000032116, "jerk"=499.99999998817657, "heading"=-0.0}, {"dt"=0.005, "x"=94.11021025000836, "y"=260.0, "position"=-94.11024150000837, "velocity"=-49.778300000005515, "acceleration"=13.629999999125175, "jerk"=499.9999997608029, "heading"=-0.0}, {"dt"=0.005, "x"=94.35869850000837, "y"=260.0, "position"=-94.35872975000838, "velocity"=-49.69765000000166, "acceleration"=16.13000000077136, "jerk"=500.0000003292371, "heading"=-0.0}, {"dt"=0.005, "x"=94.60672100000838, "y"=260.0, "position"=-94.60675225000838, "velocity"=-49.60450000000094, "acceleration"=18.63000000014381, "jerk"=499.99999987448973, "heading"=-0.0}, {"dt"=0.005, "x"=94.85421525000838, "y"=260.0, "position"=-94.85424650000839, "velocity"=-49.498850000000516, "acceleration"=21.130000000084692, "jerk"=499.99999998817657, "heading"=-0.0}, {"dt"=0.005, "x"=95.10111875000837, "y"=260.0, "position"=-95.10115000000837, "velocity"=-49.380699999997546, "acceleration"=23.63000000059401, "jerk"=500.0000001018634, "heading"=-0.0}, {"dt"=0.005, "x"=95.34736900000837, "y"=260.0, "position"=-95.34740025000838, "velocity"=-49.250050000000556, "acceleration"=26.129999999398024, "jerk"=499.9999997608029, "heading"=-0.0}, {"dt"=0.005, "x"=95.59290350000836, "y"=260.0, "position"=-95.59293475000837, "velocity"=-49.10689999999818, "acceleration"=28.630000000475775, "jerk"=500.00000021555024, "heading"=-0.0}, {"dt"=0.005, "x"=95.83765975000834, "y"=260.0, "position"=-95.83769100000835, "velocity"=-48.951249999996094, "acceleration"=31.130000000416658, "jerk"=499.99999998817657, "heading"=-0.0}, {"dt"=0.005, "x"=96.08157525000834, "y"=260.0, "position"=-96.08160650000835, "velocity"=-48.78309999999999, "acceleration"=33.62999999922067, "jerk"=499.9999997608029, "heading"=-0.0}, {"dt"=0.005, "x"=96.32458750000833, "y"=260.0, "position"=-96.32461875000834, "velocity"=-48.6024499999985, "acceleration"=36.13000000029842, "jerk"=500.00000021555024, "heading"=-0.0}, {"dt"=0.005, "x"=96.56663400000832, "y"=260.0, "position"=-96.56666525000833, "velocity"=-48.4092999999973, "acceleration"=38.630000000239306, "jerk"=499.99999998817657, "heading"=-0.0}, {"dt"=0.005, "x"=96.80765225000829, "y"=260.0, "position"=-96.8076835000083, "velocity"=-48.20364999999356, "acceleration"=41.13000000074862, "jerk"=500.0000001018634, "heading"=-0.0}, {"dt"=0.005, "x"=97.04757975000827, "y"=260.0, "position"=-97.04761100000827, "velocity"=-47.985499999995795, "acceleration"=43.62999999955264, "jerk"=499.9999997608029, "heading"=-0.0}, {"dt"=0.005, "x"=97.28635400000825, "y"=260.0, "position"=-97.28638525000825, "velocity"=-47.754849999995486, "acceleration"=46.130000000061955, "jerk"=500.0000001018634, "heading"=-0.0}, {"dt"=0.005, "x"=97.52391250000822, "y"=260.0, "position"=-97.52394375000823, "velocity"=-47.51169999999547, "acceleration"=48.63000000000284, "jerk"=499.99999998817657, "heading"=-0.0}, {"dt"=0.005, "x"=97.76022250000818, "y"=260.0, "position"=-97.76025375000819, "velocity"=-47.2619999999921, "acceleration"=49.940000000674445, "jerk"=262.00000013432145, "heading"=-0.0}, {"dt"=0.005, "x"=97.99528250000816, "y"=260.0, "position"=-97.99531375000817, "velocity"=-47.01199999999517, "acceleration"=49.99999999938609, "jerk"=11.999999742329237, "heading"=-0.0}, {"dt"=0.005, "x"=98.22909250000814, "y"=260.0, "position"=-98.22912375000814, "velocity"=-46.761999999995396, "acceleration"=49.999999999954525, "jerk"=1.1368683772161603e-07, "heading"=-0.0}, {"dt"=0.005, "x"=98.46165250000813, "y"=260.0, "position"=-98.46168375000813, "velocity"=-46.511999999998466, "acceleration"=49.99999999938609, "jerk"=-1.1368683772161603e-07, "heading"=-0.0}, {"dt"=0.005, "x"=98.6929625000081, "y"=260.0, "position"=-98.6929937500081, "velocity"=-46.26199999999301, "acceleration"=50.000000001091394, "jerk"=3.410605131648481e-07, "heading"=-0.0}, {"dt"=0.005, "x"=98.92302250000807, "y"=260.0, "position"=-98.92305375000808, "velocity"=-46.01199999999608, "acceleration"=49.99999999938609, "jerk"=-3.410605131648481e-07, "heading"=-0.0}, {"dt"=0.005, "x"=99.15183250000803, "y"=260.0, "position"=-99.15186375000803, "velocity"=-45.76199999999062, "acceleration"=50.000000001091394, "jerk"=3.410605131648481e-07, "heading"=-0.0}, {"dt"=0.005, "x"=99.37939250000798, "y"=260.0, "position"=-99.37942375000799, "velocity"=-45.51199999999085, "acceleration"=49.999999999954525, "jerk"=-2.2737367544323206e-07, "heading"=-0.0}, {"dt"=0.005, "x"=99.60570250000795, "y"=260.0, "position"=-99.60573375000796, "velocity"=-45.26199999999392, "acceleration"=49.99999999938609, "jerk"=-1.1368683772161603e-07, "heading"=-0.0}, {"dt"=0.005, "x"=99.83076250000792, "y"=260.0, "position"=-99.83079375000793, "velocity"=-45.011999999994146, "acceleration"=49.999999999954525, "jerk"=1.1368683772161603e-07, "heading"=-0.0}, {"dt"=0.005, "x"=100.0545725000079, "y"=260.0, "position"=-100.0546037500079, "velocity"=-44.76199999999437, "acceleration"=49.999999999954525, "jerk"=-0.0, "heading"=-0.0}, {"dt"=0.005, "x"=100.27713250000785, "y"=260.0, "position"=-100.27716375000786, "velocity"=-44.51199999999176, "acceleration"=50.00000000052296, "jerk"=1.1368683772161603e-07, "heading"=-0.0}, {"dt"=0.005, "x"=100.49844250000783, "y"=260.0, "position"=-100.49847375000783, "velocity"=-44.26199999999483, "acceleration"=49.99999999938609, "jerk"=-2.2737367544323206e-07, "heading"=-0.0}, {"dt"=0.005, "x"=100.71850250000782, "y"=260.0, "position"=-100.71853375000782, "velocity"=-44.0119999999979, "acceleration"=49.99999999938609, "jerk"=-0.0, "heading"=-0.0}, {"dt"=0.005, "x"=100.93731250000776, "y"=260.0, "position"=-100.93734375000777, "velocity"=-43.7619999999896, "acceleration"=50.00000000165983, "jerk"=4.547473508864641e-07, "heading"=-0.0}, {"dt"=0.005, "x"=101.15487250000774, "y"=260.0, "position"=-101.15490375000775, "velocity"=-43.51199999999551, "acceleration"=49.99999999881766, "jerk"=-5.684341886080801e-07, "heading"=-0.0}, {"dt"=0.005, "x"=101.3711825000077, "y"=260.0, "position"=-101.37121375000771, "velocity"=-43.261999999992895, "acceleration"=50.00000000052296, "jerk"=3.410605131648481e-07, "heading"=-0.0}, {"dt"=0.005, "x"=101.58624250000767, "y"=260.0, "position"=-101.58627375000768, "velocity"=-43.01199999999312, "acceleration"=49.999999999954525, "jerk"=-1.1368683772161603e-07, "heading"=-0.0}, {"dt"=0.005, "x"=101.80005250000765, "y"=260.0, "position"=-101.80008375000766, "velocity"=-42.76199999999619, "acceleration"=49.99999999938609, "jerk"=-1.1368683772161603e-07, "heading"=-0.0}, {"dt"=0.005, "x"=102.0126125000076, "y"=260.0, "position"=-102.01264375000761, "velocity"=-42.511999999990735, "acceleration"=50.000000001091394, "jerk"=3.410605131648481e-07, "heading"=-0.0}, {"dt"=0.005, "x"=102.22392250000756, "y"=260.0, "position"=-102.22395375000757, "velocity"=-42.26199999999096, "acceleration"=49.999999999954525, "jerk"=-2.2737367544323206e-07, "heading"=-0.0}, {"dt"=0.005, "x"=102.43398250000753, "y"=260.0, "position"=-102.43401375000754, "velocity"=-42.01199999999403, "acceleration"=49.99999999938609, "jerk"=-1.1368683772161603e-07, "heading"=-0.0}, {"dt"=0.005, "x"=102.6427925000075, "y"=260.0, "position"=-102.64282375000751, "velocity"=-41.76199999999426, "acceleration"=49.999999999954525, "jerk"=1.1368683772161603e-07, "heading"=-0.0}, {"dt"=0.005, "x"=102.85035250000746, "y"=260.0, "position"=-102.85038375000747, "velocity"=-41.511999999991644, "acceleration"=50.00000000052296, "jerk"=1.1368683772161603e-07, "heading"=-0.0}, {"dt"=0.005, "x"=103.05666250000743, "y"=260.0, "position"=-103.05669375000744, "velocity"=-41.261999999994714, "acceleration"=49.99999999938609, "jerk"=-2.2737367544323206e-07, "heading"=-0.0}, {"dt"=0.005, "x"=103.26172250000741, "y"=260.0, "position"=-103.26175375000741, "velocity"=-41.01199999999494, "acceleration"=49.999999999954525, "jerk"=1.1368683772161603e-07, "heading"=-0.0}, {"dt"=0.005, "x"=103.46553250000737, "y"=260.0, "position"=-103.46556375000738, "velocity"=-40.76199999999233, "acceleration"=50.00000000052296, "jerk"=1.1368683772161603e-07, "heading"=-0.0}, {"dt"=0.005, "x"=103.66809250000735, "y"=260.0, "position"=-103.66812375000735, "velocity"=-40.511999999995396, "acceleration"=49.99999999938609, "jerk"=-2.2737367544323206e-07, "heading"=-0.0}, {"dt"=0.005, "x"=103.86940250000733, "y"=260.0, "position"=-103.86943375000733, "velocity"=-40.26199999999562, "acceleration"=49.999999999954525, "jerk"=1.1368683772161603e-07, "heading"=-0.0}, {"dt"=0.005, "x"=104.06946250000728, "y"=260.0, "position"=-104.06949375000728, "velocity"=-40.01199999999017, "acceleration"=50.000000001091394, "jerk"=2.2737367544323206e-07, "heading"=-0.0}, {"dt"=0.005, "x"=104.26827250000726, "y"=260.0, "position"=-104.26830375000726, "velocity"=-39.76199999999608, "acceleration"=49.99999999881766, "jerk"=-4.547473508864641e-07, "heading"=-0.0}, {"dt"=0.005, "x"=104.46583250000721, "y"=260.0, "position"=-104.46586375000722, "velocity"=-39.51199999999062, "acceleration"=50.000000001091394, "jerk"=4.547473508864641e-07, "heading"=-0.0}, {"dt"=0.005, "x"=104.66214250000716, "y"=260.0, "position"=-104.66217375000717, "velocity"=-39.26199999999085, "acceleration"=49.999999999954525, "jerk"=-2.2737367544323206e-07, "heading"=-0.0}, {"dt"=0.005, "x"=104.85720250000713, "y"=260.0, "position"=-104.85723375000714, "velocity"=-39.01199999999392, "acceleration"=49.99999999938609, "jerk"=-1.1368683772161603e-07, "heading"=-0.0}, {"dt"=0.005, "x"=105.05101250000709, "y"=260.0, "position"=-105.0510437500071, "velocity"=-38.7619999999913, "acceleration"=50.00000000052296, "jerk"=2.2737367544323206e-07, "heading"=-0.0}, {"dt"=0.005, "x"=105.24357250000706, "y"=260.0, "position"=-105.24360375000707, "velocity"=-38.51199999999437, "acceleration"=49.99999999938609, "jerk"=-2.2737367544323206e-07, "heading"=-0.0}, {"dt"=0.005, "x"=105.43488250000703, "y"=260.0, "position"=-105.43491375000704, "velocity"=-38.2619999999946, "acceleration"=49.999999999954525, "jerk"=1.1368683772161603e-07, "heading"=-0.0}, {"dt"=0.005, "x"=105.624942500007, "y"=260.0, "position"=-105.624973750007, "velocity"=-38.011999999991986, "acceleration"=50.00000000052296, "jerk"=1.1368683772161603e-07, "heading"=-0.0}, {"dt"=0.005, "x"=105.81375250000697, "y"=260.0, "position"=-105.81378375000698, "velocity"=-37.761999999995055, "acceleration"=49.99999999938609, "jerk"=-2.2737367544323206e-07, "heading"=-0.0}, {"dt"=0.005, "x"=106.00131250000693, "y"=260.0, "position"=-106.00134375000694, "velocity"=-37.51199999999244, "acceleration"=50.00000000052296, "jerk"=2.2737367544323206e-07, "heading"=-0.0}, {"dt"=0.005, "x"=106.1876225000069, "y"=260.0, "position"=-106.1876537500069, "velocity"=-37.26199999999267, "acceleration"=49.999999999954525, "jerk"=-1.1368683772161603e-07, "heading"=-0.0}, {"dt"=0.005, "x"=106.37268250000686, "y"=260.0, "position"=-106.37271375000687, "velocity"=-37.011999999992895, "acceleration"=49.999999999954525, "jerk"=-0.0, "heading"=-0.0}, {"dt"=0.005, "x"=106.55649250000683, "y"=260.0, "position"=-106.55652375000683, "velocity"=-36.76199999999312, "acceleration"=49.999999999954525, "jerk"=-0.0, "heading"=-0.0}, {"dt"=0.005, "x"=106.73905250000678, "y"=260.0, "position"=-106.73908375000678, "velocity"=-36.51199999999051, "acceleration"=50.00000000052296, "jerk"=1.1368683772161603e-07, "heading"=-0.0}, {"dt"=0.005, "x"=106.92036250000675, "y"=260.0, "position"=-106.92039375000675, "velocity"=-36.26199999999358, "acceleration"=49.99999999938609, "jerk"=-2.2737367544323206e-07, "heading"=-0.0}, {"dt"=0.005, "x"=107.1004225000067, "y"=260.0, "position"=-107.10045375000671, "velocity"=-36.01199999999096, "acceleration"=50.00000000052296, "jerk"=2.2737367544323206e-07, "heading"=-0.0}, {"dt"=0.005, "x"=107.27923250000667, "y"=260.0, "position"=-107.27926375000668, "velocity"=-35.76199999999403, "acceleration"=49.99999999938609, "jerk"=-2.2737367544323206e-07, "heading"=-0.0}, {"dt"=0.005, "x"=107.45679250000663, "y"=260.0, "position"=-107.45682375000663, "velocity"=-35.51199999999142, "acceleration"=50.00000000052296, "jerk"=2.2737367544323206e-07, "heading"=-0.0}, {"dt"=0.005, "x"=107.6331025000066, "y"=260.0, "position"=-107.6331337500066, "velocity"=-35.26199999999449, "acceleration"=49.99999999938609, "jerk"=-2.2737367544323206e-07, "heading"=-0.0}, {"dt"=0.005, "x"=107.80816250000656, "y"=260.0, "position"=-107.80819375000657, "velocity"=-35.01199999999187, "acceleration"=50.00000000052296, "jerk"=2.2737367544323206e-07, "heading"=-0.0}, {"dt"=0.005, "x"=107.98197250000652, "y"=260.0, "position"=-107.98200375000653, "velocity"=-34.7619999999921, "acceleration"=49.999999999954525, "jerk"=-1.1368683772161603e-07, "heading"=-0.0}, {"dt"=0.005, "x"=108.15453250000648, "y"=260.0, "position"=-108.15456375000649, "velocity"=-34.51199999999233, "acceleration"=49.999999999954525, "jerk"=-0.0, "heading"=-0.0}, {"dt"=0.005, "x"=108.32584250000647, "y"=260.0, "position"=-108.32587375000648, "velocity"=-34.26199999999824, "acceleration"=49.99999999881766, "jerk"=-2.2737367544323206e-07, "heading"=-0.0}, {"dt"=0.005, "x"=108.49590250000642, "y"=260.0, "position"=-108.49593375000643, "velocity"=-34.01199999998994, "acceleration"=50.00000000165983, "jerk"=5.684341886080801e-07, "heading"=-0.0}, {"dt"=0.005, "x"=108.66471250000639, "y"=260.0, "position"=-108.6647437500064, "velocity"=-33.76199999999301, "acceleration"=49.99999999938609, "jerk"=-4.547473508864641e-07, "heading"=-0.0}, {"dt"=0.005, "x"=108.83227250000635, "y"=260.0, "position"=-108.83230375000636, "velocity"=-33.511999999993236, "acceleration"=49.999999999954525, "jerk"=1.1368683772161603e-07, "heading"=-0.0}, {"dt"=0.005, "x"=108.99858250000631, "y"=260.0, "position"=-108.99861375000631, "velocity"=-33.26199999999062, "acceleration"=50.00000000052296, "jerk"=1.1368683772161603e-07, "heading"=-0.0}, {"dt"=0.005, "x"=109.16364250000626, "y"=260.0, "position"=-109.16367375000627, "velocity"=-33.01199999999085, "acceleration"=49.999999999954525, "jerk"=-1.1368683772161603e-07, "heading"=-0.0}, {"dt"=0.005, "x"=109.32745250000623, "y"=260.0, "position"=-109.32748375000624, "velocity"=-32.76199999999392, "acceleration"=49.99999999938609, "jerk"=-1.1368683772161603e-07, "heading"=-0.0}, {"dt"=0.005, "x"=109.49001250000619, "y"=260.0, "position"=-109.4900437500062, "velocity"=-32.5119999999913, "acceleration"=50.00000000052296, "jerk"=2.2737367544323206e-07, "heading"=-0.0}, {"dt"=0.005, "x"=109.65132250000615, "y"=260.0, "position"=-109.65135375000615, "velocity"=-32.26199999999153, "acceleration"=49.999999999954525, "jerk"=-1.1368683772161603e-07, "heading"=-0.0}, {"dt"=0.005, "x"=109.81138250000612, "y"=260.0, "position"=-109.81141375000612, "velocity"=-32.0119999999946, "acceleration"=49.99999999938609, "jerk"=-1.1368683772161603e-07, "heading"=-0.0}, {"dt"=0.005, "x"=109.97019250000606, "y"=260.0, "position"=-109.97022375000607, "velocity"=-31.761999999989143, "acceleration"=50.000000001091394, "jerk"=3.410605131648481e-07, "heading"=-0.0}, {"dt"=0.005, "x"=110.12775250000603, "y"=260.0, "position"=-110.12778375000603, "velocity"=-31.511999999992213, "acceleration"=49.99999999938609, "jerk"=-3.410605131648481e-07, "heading"=-0.0}, {"dt"=0.005, "x"=110.284062500006, "y"=260.0, "position"=-110.28409375000601, "velocity"=-31.261999999995282, "acceleration"=49.99999999938609, "jerk"=-0.0, "heading"=-0.0}, {"dt"=0.005, "x"=110.43912250000598, "y"=260.0, "position"=-110.43915375000599, "velocity"=-31.01199999999551, "acceleration"=49.999999999954525, "jerk"=1.1368683772161603e-07, "heading"=-0.0}, {"dt"=0.005, "x"=110.59293250000593, "y"=260.0, "position"=-110.59296375000594, "velocity"=-30.761999999990053, "acceleration"=50.000000001091394, "jerk"=2.2737367544323206e-07, "heading"=-0.0}, {"dt"=0.005, "x"=110.7454925000059, "y"=260.0, "position"=-110.7455237500059, "velocity"=-30.511999999993122, "acceleration"=49.99999999938609, "jerk"=-3.410605131648481e-07, "heading"=-0.0}, {"dt"=0.005, "x"=110.89680250000585, "y"=260.0, "position"=-110.89683375000585, "velocity"=-30.261999999990508, "acceleration"=50.00000000052296, "jerk"=2.2737367544323206e-07, "heading"=-0.0}, {"dt"=0.005, "x"=111.0468625000058, "y"=260.0, "position"=-111.04689375000581, "velocity"=-30.011999999990735, "acceleration"=49.999999999954525, "jerk"=-1.1368683772161603e-07, "heading"=-0.0}, {"dt"=0.005, "x"=111.19567250000576, "y"=260.0, "position"=-111.19570375000576, "velocity"=-29.761999999990962, "acceleration"=49.999999999954525, "jerk"=-0.0, "heading"=-0.0}, {"dt"=0.005, "x"=111.34323250000571, "y"=260.0, "position"=-111.34326375000572, "velocity"=-29.51199999999119, "acceleration"=49.999999999954525, "jerk"=-0.0, "heading"=-0.0}, {"dt"=0.005, "x"=111.48954250000568, "y"=260.0, "position"=-111.48957375000569, "velocity"=-29.26199999999426, "acceleration"=49.99999999938609, "jerk"=-1.1368683772161603e-07, "heading"=-0.0}, {"dt"=0.005, "x"=111.63460250000564, "y"=260.0, "position"=-111.63463375000565, "velocity"=-29.011999999991644, "acceleration"=50.00000000052296, "jerk"=2.2737367544323206e-07, "heading"=-0.0}, {"dt"=0.005, "x"=111.77841250000559, "y"=260.0, "position"=-111.7784437500056, "velocity"=-28.76199999998903, "acceleration"=50.00000000052296, "jerk"=-0.0, "heading"=-0.0}, {"dt"=0.005, "x"=111.92097250000555, "y"=260.0, "position"=-111.92100375000555, "velocity"=-28.5119999999921, "acceleration"=49.99999999938609, "jerk"=-2.2737367544323206e-07, "heading"=-0.0}, {"dt"=0.005, "x"=112.06228250000552, "y"=260.0, "position"=-112.06231375000553, "velocity"=-28.26199999999517, "acceleration"=49.99999999938609, "jerk"=-0.0, "heading"=-0.0}, {"dt"=0.005, "x"=112.2023425000055, "y"=260.0, "position"=-112.2023737500055, "velocity"=-28.011999999995396, "acceleration"=49.999999999954525, "jerk"=1.1368683772161603e-07, "heading"=-0.0}, {"dt"=0.005, "x"=112.34115250000545, "y"=260.0, "position"=-112.34118375000546, "velocity"=-27.76199999998994, "acceleration"=50.000000001091394, "jerk"=2.2737367544323206e-07, "heading"=-0.0}, {"dt"=0.005, "x"=112.4787125000054, "y"=260.0, "position"=-112.4787437500054, "velocity"=-27.511999999990167, "acceleration"=49.999999999954525, "jerk"=-2.2737367544323206e-07, "heading"=-0.0}, {"dt"=0.005, "x"=112.61502250000535, "y"=260.0, "position"=-112.61505375000536, "velocity"=-27.261999999990394, "acceleration"=49.999999999954525, "jerk"=-0.0, "heading"=-0.0}, {"dt"=0.005, "x"=112.7500825000053, "y"=260.0, "position"=-112.75011375000531, "velocity"=-27.01199999999062, "acceleration"=49.999999999954525, "jerk"=-0.0, "heading"=-0.0}, {"dt"=0.005, "x"=112.88389250000526, "y"=260.0, "position"=-112.88392375000527, "velocity"=-26.76199999999085, "acceleration"=49.999999999954525, "jerk"=-0.0, "heading"=-0.0}, {"dt"=0.005, "x"=113.01645250000522, "y"=260.0, "position"=-113.01648375000522, "velocity"=-26.511999999991076, "acceleration"=49.999999999954525, "jerk"=-0.0, "heading"=-0.0}, {"dt"=0.005, "x"=113.14776250000517, "y"=260.0, "position"=-113.14779375000518, "velocity"=-26.261999999991303, "acceleration"=49.999999999954525, "jerk"=-0.0, "heading"=-0.0}, {"dt"=0.005, "x"=113.27782250000513, "y"=260.0, "position"=-113.27785375000514, "velocity"=-26.01199999999153, "acceleration"=49.999999999954525, "jerk"=-0.0, "heading"=-0.0}, {"dt"=0.005, "x"=113.4066325000051, "y"=260.0, "position"=-113.40666375000511, "velocity"=-25.7619999999946, "acceleration"=49.99999999938609, "jerk"=-1.1368683772161603e-07, "heading"=-0.0}, {"dt"=0.005, "x"=113.53419250000506, "y"=260.0, "position"=-113.53422375000507, "velocity"=-25.511999999991986, "acceleration"=50.00000000052296, "jerk"=2.2737367544323206e-07, "heading"=-0.0}, {"dt"=0.005, "x"=113.66050250000501, "y"=260.0, "position"=-113.66053375000502, "velocity"=-25.26199999998937, "acceleration"=50.00000000052296, "jerk"=-0.0, "heading"=-0.0}, {"dt"=0.005, "x"=113.78556250000497, "y"=260.0, "position"=-113.78559375000498, "velocity"=-25.01199999999244, "acceleration"=49.99999999938609, "jerk"=-2.2737367544323206e-07, "heading"=-0.0}, {"dt"=0.005, "x"=113.90937250000495, "y"=260.0, "position"=-113.90940375000496, "velocity"=-24.76199999999551, "acceleration"=49.99999999938609, "jerk"=-0.0, "heading"=-0.0}, {"dt"=0.005, "x"=114.0319325000049, "y"=260.0, "position"=-114.0319637500049, "velocity"=-24.511999999990053, "acceleration"=50.000000001091394, "jerk"=3.410605131648481e-07, "heading"=-0.0}, {"dt"=0.005, "x"=114.15324250000486, "y"=260.0, "position"=-114.15327375000487, "velocity"=-24.261999999993122, "acceleration"=49.99999999938609, "jerk"=-3.410605131648481e-07, "heading"=-0.0}, {"dt"=0.005, "x"=114.2733025000048, "y"=260.0, "position"=-114.27333375000481, "velocity"=-24.011999999987665, "acceleration"=50.000000001091394, "jerk"=3.410605131648481e-07, "heading"=-0.0}, {"dt"=0.005, "x"=114.39211250000476, "y"=260.0, "position"=-114.39214375000476, "velocity"=-23.761999999990735, "acceleration"=49.99999999938609, "jerk"=-3.410605131648481e-07, "heading"=-0.0}, {"dt"=0.005, "x"=114.50967250000471, "y"=260.0, "position"=-114.50970375000472, "velocity"=-23.511999999990962, "acceleration"=49.999999999954525, "jerk"=1.1368683772161603e-07, "heading"=-0.0}, {"dt"=0.005, "x"=114.62598250000467, "y"=260.0, "position"=-114.62601375000467, "velocity"=-23.26199999999119, "acceleration"=49.999999999954525, "jerk"=-0.0, "heading"=-0.0}, {"dt"=0.005, "x"=114.74104250000462, "y"=260.0, "position"=-114.74107375000463, "velocity"=-23.011999999991417, "acceleration"=49.999999999954525, "jerk"=-0.0, "heading"=-0.0}, {"dt"=0.005, "x"=114.85485250000458, "y"=260.0, "position"=-114.85488375000459, "velocity"=-22.761999999991644, "acceleration"=49.999999999954525, "jerk"=-0.0, "heading"=-0.0}, {"dt"=0.005, "x"=114.96741250000453, "y"=260.0, "position"=-114.96744375000453, "velocity"=-22.51199999998903, "acceleration"=50.00000000052296, "jerk"=1.1368683772161603e-07, "heading"=-0.0}, {"dt"=0.005, "x"=115.07872250000449, "y"=260.0, "position"=-115.0787537500045, "velocity"=-22.2619999999921, "acceleration"=49.99999999938609, "jerk"=-2.2737367544323206e-07, "heading"=-0.0}, {"dt"=0.005, "x"=115.18878250000444, "y"=260.0, "position"=-115.18881375000444, "velocity"=-22.011999999989484, "acceleration"=50.00000000052296, "jerk"=2.2737367544323206e-07, "heading"=-0.0}, {"dt"=0.005, "x"=115.29759250000441, "y"=260.0, "position"=-115.29762375000442, "velocity"=-21.761999999995396, "acceleration"=49.99999999881766, "jerk"=-3.410605131648481e-07, "heading"=-0.0}, {"dt"=0.005, "x"=115.40515250000438, "y"=260.0, "position"=-115.40518375000438, "velocity"=-21.51199999999278, "acceleration"=50.00000000052296, "jerk"=3.410605131648481e-07, "heading"=-0.0}, {"dt"=0.005, "x"=115.51146250000434, "y"=260.0, "position"=-115.51149375000435, "velocity"=-21.26199999999301, "acceleration"=49.999999999954525, "jerk"=-1.1368683772161603e-07, "heading"=-0.0}, {"dt"=0.005, "x"=115.6165225000043, "y"=260.0, "position"=-115.6165537500043, "velocity"=-21.011999999990394, "acceleration"=50.00000000052296, "jerk"=1.1368683772161603e-07, "heading"=-0.0}, {"dt"=0.005, "x"=115.72033250000425, "y"=260.0, "position"=-115.72036375000425, "velocity"=-20.76199999999062, "acceleration"=49.999999999954525, "jerk"=-1.1368683772161603e-07, "heading"=-0.0}, {"dt"=0.005, "x"=115.82289250000417, "y"=260.0, "position"=-115.82292375000418, "velocity"=-20.511999999985164, "acceleration"=50.000000001091394, "jerk"=2.2737367544323206e-07, "heading"=-0.0}, {"dt"=0.005, "x"=115.92420250000413, "y"=260.0, "position"=-115.92423375000413, "velocity"=-20.261999999991076, "acceleration"=49.99999999881766, "jerk"=-4.547473508864641e-07, "heading"=-0.0}, {"dt"=0.005, "x"=116.02426250000408, "y"=260.0, "position"=-116.02429375000409, "velocity"=-20.011999999991303, "acceleration"=49.999999999954525, "jerk"=2.2737367544323206e-07, "heading"=-0.0}, {"dt"=0.005, "x"=116.12307250000404, "y"=260.0, "position"=-116.12310375000405, "velocity"=-19.76199999999153, "acceleration"=49.999999999954525, "jerk"=-0.0, "heading"=-0.0}, {"dt"=0.005, "x"=116.220632500004, "y"=260.0, "position"=-116.22066375000401, "velocity"=-19.511999999991758, "acceleration"=49.999999999954525, "jerk"=-0.0, "heading"=-0.0}, {"dt"=0.005, "x"=116.31694250000396, "y"=260.0, "position"=-116.31697375000397, "velocity"=-19.261999999991986, "acceleration"=49.999999999954525, "jerk"=-0.0, "heading"=-0.0}, {"dt"=0.005, "x"=116.41200250000391, "y"=260.0, "position"=-116.41203375000391, "velocity"=-19.01199999998937, "acceleration"=50.00000000052296, "jerk"=1.1368683772161603e-07, "heading"=-0.0}, {"dt"=0.005, "x"=116.50581250000387, "y"=260.0, "position"=-116.50584375000388, "velocity"=-18.76199999999244, "acceleration"=49.99999999938609, "jerk"=-2.2737367544323206e-07, "heading"=-0.0}, {"dt"=0.005, "x"=116.59837250000383, "y"=260.0, "position"=-116.59840375000384, "velocity"=-18.511999999992668, "acceleration"=49.999999999954525, "jerk"=1.1368683772161603e-07, "heading"=-0.0}, {"dt"=0.005, "x"=116.6896825000038, "y"=260.0, "position"=-116.6897137500038, "velocity"=-18.261999999992895, "acceleration"=49.999999999954525, "jerk"=-0.0, "heading"=-0.0}, {"dt"=0.005, "x"=116.77974250000374, "y"=260.0, "position"=-116.77977375000374, "velocity"=-18.011999999987438, "acceleration"=50.000000001091394, "jerk"=2.2737367544323206e-07, "heading"=-0.0}, {"dt"=0.005, "x"=116.86855250000369, "y"=260.0, "position"=-116.8685837500037, "velocity"=-17.761999999990508, "acceleration"=49.99999999938609, "jerk"=-3.410605131648481e-07, "heading"=-0.0}, {"dt"=0.005, "x"=116.95611250000364, "y"=260.0, "position"=-116.95614375000365, "velocity"=-17.511999999990735, "acceleration"=49.999999999954525, "jerk"=1.1368683772161603e-07, "heading"=-0.0}, {"dt"=0.005, "x"=117.0424225000036, "y"=260.0, "position"=-117.0424537500036, "velocity"=-17.261999999990962, "acceleration"=49.999999999954525, "jerk"=-0.0, "heading"=-0.0}, {"dt"=0.005, "x"=117.12748250000354, "y"=260.0, "position"=-117.12751375000354, "velocity"=-17.011999999988348, "acceleration"=50.00000000052296, "jerk"=1.1368683772161603e-07, "heading"=-0.0}, {"dt"=0.005, "x"=117.2112925000035, "y"=260.0, "position"=-117.2113237500035, "velocity"=-16.761999999991417, "acceleration"=49.99999999938609, "jerk"=-2.2737367544323206e-07, "heading"=-0.0}, {"dt"=0.005, "x"=117.29385250000345, "y"=260.0, "position"=-117.29388375000346, "velocity"=-16.511999999991644, "acceleration"=49.999999999954525, "jerk"=1.1368683772161603e-07, "heading"=-0.0}, {"dt"=0.005, "x"=117.37516250000338, "y"=260.0, "position"=-117.37519375000339, "velocity"=-16.261999999986188, "acceleration"=50.000000001091394, "jerk"=2.2737367544323206e-07, "heading"=-0.0}, {"dt"=0.005, "x"=117.45522250000334, "y"=260.0, "position"=-117.45525375000335, "velocity"=-16.0119999999921, "acceleration"=49.99999999881766, "jerk"=-4.547473508864641e-07, "heading"=-0.0}, {"dt"=0.005, "x"=117.53403250000332, "y"=260.0, "position"=-117.53406375000333, "velocity"=-15.761999999995169, "acceleration"=49.99999999938609, "jerk"=1.1368683772161603e-07, "heading"=-0.0}, {"dt"=0.005, "x"=117.61159250000327, "y"=260.0, "position"=-117.61162375000328, "velocity"=-15.511999999989712, "acceleration"=50.000000001091394, "jerk"=3.410605131648481e-07, "heading"=-0.0}, {"dt"=0.005, "x"=117.68790250000323, "y"=260.0, "position"=-117.68793375000324, "velocity"=-15.261999999992781, "acceleration"=49.99999999938609, "jerk"=-3.410605131648481e-07, "heading"=-0.0}, {"dt"=0.005, "x"=117.76296250000318, "y"=260.0, "position"=-117.76299375000319, "velocity"=-15.011999999990167, "acceleration"=50.00000000052296, "jerk"=2.2737367544323206e-07, "heading"=-0.0}, {"dt"=0.005, "x"=117.83677250000312, "y"=260.0, "position"=-117.83680375000313, "velocity"=-14.761999999987552, "acceleration"=50.00000000052296, "jerk"=-0.0, "heading"=-0.0}, {"dt"=0.005, "x"=117.90933250000307, "y"=260.0, "position"=-117.90936375000308, "velocity"=-14.511999999990621, "acceleration"=49.99999999938609, "jerk"=-2.2737367544323206e-07, "heading"=-0.0}, {"dt"=0.005, "x"=117.98064250000303, "y"=260.0, "position"=-117.98067375000304, "velocity"=-14.261999999990849, "acceleration"=49.999999999954525, "jerk"=1.1368683772161603e-07, "heading"=-0.0}, {"dt"=0.005, "x"=118.05070250000297, "y"=260.0, "position"=-118.05073375000298, "velocity"=-14.011999999988234, "acceleration"=50.00000000052296, "jerk"=1.1368683772161603e-07, "heading"=-0.0}, {"dt"=0.005, "x"=118.11951250000293, "y"=260.0, "position"=-118.11954375000293, "velocity"=-13.761999999991303, "acceleration"=49.99999999938609, "jerk"=-2.2737367544323206e-07, "heading"=-0.0}, {"dt"=0.005, "x"=118.18707250000287, "y"=260.0, "position"=-118.18710375000288, "velocity"=-13.511999999988689, "acceleration"=50.00000000052296, "jerk"=2.2737367544323206e-07, "heading"=-0.0}, {"dt"=0.005, "x"=118.25338250000283, "y"=260.0, "position"=-118.25341375000284, "velocity"=-13.261999999991758, "acceleration"=49.99999999938609, "jerk"=-2.2737367544323206e-07, "heading"=-0.0}, {"dt"=0.005, "x"=118.31844250000277, "y"=260.0, "position"=-118.31847375000278, "velocity"=-13.011999999989143, "acceleration"=50.00000000052296, "jerk"=2.2737367544323206e-07, "heading"=-0.0}, {"dt"=0.005, "x"=118.38225250000274, "y"=260.0, "position"=-118.38228375000274, "velocity"=-12.761999999992213, "acceleration"=49.99999999938609, "jerk"=-2.2737367544323206e-07, "heading"=-0.0}, {"dt"=0.005, "x"=118.44481250000268, "y"=260.0, "position"=-118.44484375000269, "velocity"=-12.511999999989598, "acceleration"=50.00000000052296, "jerk"=2.2737367544323206e-07, "heading"=-0.0}, {"dt"=0.005, "x"=118.50612250000265, "y"=260.0, "position"=-118.50615375000265, "velocity"=-12.261999999992668, "acceleration"=49.99999999938609, "jerk"=-2.2737367544323206e-07, "heading"=-0.0}, {"dt"=0.005, "x"=118.5661825000026, "y"=260.0, "position"=-118.5662137500026, "velocity"=-12.011999999990053, "acceleration"=50.00000000052296, "jerk"=2.2737367544323206e-07, "heading"=-0.0}, {"dt"=0.005, "x"=118.62499250000255, "y"=260.0, "position"=-118.62502375000255, "velocity"=-11.76199999999028, "acceleration"=49.999999999954525, "jerk"=-1.1368683772161603e-07, "heading"=-0.0}, {"dt"=0.005, "x"=118.68255250000249, "y"=260.0, "position"=-118.6825837500025, "velocity"=-11.511999999987665, "acceleration"=50.00000000052296, "jerk"=1.1368683772161603e-07, "heading"=-0.0}, {"dt"=0.005, "x"=118.73886250000244, "y"=260.0, "position"=-118.73889375000245, "velocity"=-11.261999999990735, "acceleration"=49.99999999938609, "jerk"=-2.2737367544323206e-07, "heading"=-0.0}, {"dt"=0.005, "x"=118.79392250000238, "y"=260.0, "position"=-118.79395375000239, "velocity"=-11.01199999998812, "acceleration"=50.00000000052296, "jerk"=2.2737367544323206e-07, "heading"=-0.0}, {"dt"=0.005, "x"=118.84773250000232, "y"=260.0, "position"=-118.84776375000233, "velocity"=-10.761999999988348, "acceleration"=49.999999999954525, "jerk"=-1.1368683772161603e-07, "heading"=-0.0}, {"dt"=0.005, "x"=118.90029250000228, "y"=260.0, "position"=-118.90032375000229, "velocity"=-10.511999999991417, "acceleration"=49.99999999938609, "jerk"=-1.1368683772161603e-07, "heading"=-0.0}, {"dt"=0.005, "x"=118.95160250000222, "y"=260.0, "position"=-118.95163375000223, "velocity"=-10.261999999988802, "acceleration"=50.00000000052296, "jerk"=2.2737367544323206e-07, "heading"=-0.0}, {"dt"=0.005, "x"=119.00166250000217, "y"=260.0, "position"=-119.00169375000218, "velocity"=-10.01199999998903, "acceleration"=49.999999999954525, "jerk"=-1.1368683772161603e-07, "heading"=-0.0}, {"dt"=0.005, "x"=119.05047250000212, "y"=260.0, "position"=-119.05050375000212, "velocity"=-9.761999999989257, "acceleration"=49.999999999954525, "jerk"=-0.0, "heading"=-0.0}, {"dt"=0.005, "x"=119.09803250000208, "y"=260.0, "position"=-119.09806375000208, "velocity"=-9.511999999992327, "acceleration"=49.99999999938609, "jerk"=-1.1368683772161603e-07, "heading"=-0.0}, {"dt"=0.005, "x"=119.14434250000204, "y"=260.0, "position"=-119.14437375000205, "velocity"=-9.261999999992554, "acceleration"=49.999999999954525, "jerk"=1.1368683772161603e-07, "heading"=-0.0}, {"dt"=0.005, "x"=119.18940250000199, "y"=260.0, "position"=-119.189433750002, "velocity"=-9.01199999998994, "acceleration"=50.00000000052296, "jerk"=1.1368683772161603e-07, "heading"=-0.0}, {"dt"=0.005, "x"=119.23321250000195, "y"=260.0, "position"=-119.23324375000196, "velocity"=-8.761999999993009, "acceleration"=49.99999999938609, "jerk"=-2.2737367544323206e-07, "heading"=-0.0}, {"dt"=0.005, "x"=119.27577250000189, "y"=260.0, "position"=-119.2758037500019, "velocity"=-8.511999999987552, "acceleration"=50.000000001091394, "jerk"=3.410605131648481e-07, "heading"=-0.0}, {"dt"=0.005, "x"=119.31708250000183, "y"=260.0, "position"=-119.31711375000184, "velocity"=-8.26199999998778, "acceleration"=49.999999999954525, "jerk"=-2.2737367544323206e-07, "heading"=-0.0}, {"dt"=0.005, "x"=119.35714250000179, "y"=260.0, "position"=-119.35717375000179, "velocity"=-8.011999999990849, "acceleration"=49.99999999938609, "jerk"=-1.1368683772161603e-07, "heading"=-0.0}, {"dt"=0.005, "x"=119.39595250000171, "y"=260.0, "position"=-119.39598375000172, "velocity"=-7.761999999985392, "acceleration"=50.000000001091394, "jerk"=3.410605131648481e-07, "heading"=-0.0}, {"dt"=0.005, "x"=119.43351250000167, "y"=260.0, "position"=-119.43354375000168, "velocity"=-7.511999999991303, "acceleration"=49.99999999881766, "jerk"=-4.547473508864641e-07, "heading"=-0.0}, {"dt"=0.005, "x"=119.46982250000163, "y"=260.0, "position"=-119.46985375000163, "velocity"=-7.261999999991531, "acceleration"=49.999999999954525, "jerk"=2.2737367544323206e-07, "heading"=-0.0}, {"dt"=0.005, "x"=119.50488250000157, "y"=260.0, "position"=-119.50491375000158, "velocity"=-7.011999999988916, "acceleration"=50.00000000052296, "jerk"=1.1368683772161603e-07, "heading"=-0.0}, {"dt"=0.005, "x"=119.53869250000152, "y"=260.0, "position"=-119.53872375000152, "velocity"=-6.761999999989143, "acceleration"=49.999999999954525, "jerk"=-1.1368683772161603e-07, "heading"=-0.0}, {"dt"=0.005, "x"=119.57125250000146, "y"=260.0, "position"=-119.57128375000147, "velocity"=-6.511999999989371, "acceleration"=49.999999999954525, "jerk"=-0.0, "heading"=-0.0}, {"dt"=0.005, "x"=119.60256250000143, "y"=260.0, "position"=-119.60259375000143, "velocity"=-6.26199999999244, "acceleration"=49.99999999938609, "jerk"=-1.1368683772161603e-07, "heading"=-0.0}, {"dt"=0.005, "x"=119.63262250000137, "y"=260.0, "position"=-119.63265375000138, "velocity"=-6.0119999999898255, "acceleration"=50.00000000052296, "jerk"=2.2737367544323206e-07, "heading"=-0.0}, {"dt"=0.005, "x"=119.66143250000133, "y"=260.0, "position"=-119.66146375000133, "velocity"=-5.761999999990053, "acceleration"=49.999999999954525, "jerk"=-1.1368683772161603e-07, "heading"=-0.0}, {"dt"=0.005, "x"=119.68899250000128, "y"=260.0, "position"=-119.68902375000128, "velocity"=-5.51199999999028, "acceleration"=49.999999999954525, "jerk"=-0.0, "heading"=-0.0}, {"dt"=0.005, "x"=119.7153025000012, "y"=260.0, "position"=-119.71533375000121, "velocity"=-5.261999999984823, "acceleration"=50.000000001091394, "jerk"=2.2737367544323206e-07, "heading"=-0.0}, {"dt"=0.005, "x"=119.74036250000115, "y"=260.0, "position"=-119.74039375000116, "velocity"=-5.011999999990735, "acceleration"=49.99999999881766, "jerk"=-4.547473508864641e-07, "heading"=-0.0}, {"dt"=0.005, "x"=119.76417250000108, "y"=260.0, "position"=-119.76420375000109, "velocity"=-4.761999999985278, "acceleration"=50.000000001091394, "jerk"=4.547473508864641e-07, "heading"=-0.0}, {"dt"=0.005, "x"=119.78673250000102, "y"=260.0, "position"=-119.78676375000103, "velocity"=-4.5119999999883476, "acceleration"=49.99999999938609, "jerk"=-3.410605131648481e-07, "heading"=-0.0}, {"dt"=0.005, "x"=119.80804250000098, "y"=260.0, "position"=-119.80807375000099, "velocity"=-4.261999999991417, "acceleration"=49.99999999938609, "jerk"=-0.0, "heading"=-0.0}, {"dt"=0.005, "x"=119.82810250000094, "y"=260.0, "position"=-119.82813375000094, "velocity"=-4.0119999999916445, "acceleration"=49.999999999954525, "jerk"=1.1368683772161603e-07, "heading"=-0.0}, {"dt"=0.005, "x"=119.84691250000087, "y"=260.0, "position"=-119.84694375000088, "velocity"=-3.7619999999861875, "acceleration"=50.000000001091394, "jerk"=2.2737367544323206e-07, "heading"=-0.0}, {"dt"=0.005, "x"=119.86447250000082, "y"=260.0, "position"=-119.86450375000082, "velocity"=-3.511999999989257, "acceleration"=49.99999999938609, "jerk"=-3.410605131648481e-07, "heading"=-0.0}, {"dt"=0.005, "x"=119.88078250000076, "y"=260.0, "position"=-119.88081375000077, "velocity"=-3.2619999999894844, "acceleration"=49.999999999954525, "jerk"=1.1368683772161603e-07, "heading"=-0.0}, {"dt"=0.005, "x"=119.89584250000071, "y"=260.0, "position"=-119.89587375000072, "velocity"=-3.011999999989712, "acceleration"=49.999999999954525, "jerk"=-0.0, "heading"=-0.0}, {"dt"=0.005, "x"=119.90965250000066, "y"=260.0, "position"=-119.90968375000067, "velocity"=-2.761999999989939, "acceleration"=49.999999999954525, "jerk"=-0.0, "heading"=-0.0}, {"dt"=0.005, "x"=119.92221250000061, "y"=260.0, "position"=-119.92224375000062, "velocity"=-2.5119999999901665, "acceleration"=49.999999999954525, "jerk"=-0.0, "heading"=-0.0}, {"dt"=0.005, "x"=119.93355225000059, "y"=260.0, "position"=-119.9335835000006, "velocity"=-2.267949999995267, "acceleration"=48.80999999897995, "jerk"=-238.00000019491563, "heading"=-0.0}, {"dt"=0.005, "x"=119.94373275000054, "y"=260.0, "position"=-119.94376400000054, "velocity"=-2.0360999999894602, "acceleration"=46.370000001161316, "jerk"=-487.9999995637263, "heading"=-0.0}, {"dt"=0.005, "x"=119.95281650000047, "y"=260.0, "position"=-119.95284775000047, "velocity"=-1.8167499999862002, "acceleration"=43.870000000652, "jerk"=-500.0000001018634, "heading"=-0.0}, {"dt"=0.005, "x"=119.96086600000042, "y"=260.0, "position"=-119.96089725000043, "velocity"=-1.6098999999911712, "acceleration"=41.36999999900581, "jerk"=-500.0000003292371, "heading"=-0.0}, {"dt"=0.005, "x"=119.96794375000037, "y"=260.0, "position"=-119.96797500000038, "velocity"=-1.4155499999901622, "acceleration"=38.8700000002018, "jerk"=-499.9999997608029, "heading"=-0.0}, {"dt"=0.005, "x"=119.97411225000033, "y"=260.0, "position"=-119.97414350000034, "velocity"=-1.2336999999916998, "acceleration"=36.36999999969248, "jerk"=-500.0000001018634, "heading"=-0.0}, {"dt"=0.005, "x"=119.97943400000031, "y"=260.0, "position"=-119.97946525000032, "velocity"=-1.064349999995784, "acceleration"=33.869999999183165, "jerk"=-500.0000001018634, "heading"=-0.0}, {"dt"=0.005, "x"=119.98397150000027, "y"=260.0, "position"=-119.98400275000027, "velocity"=-0.907499999991046, "acceleration"=31.370000000947584, "jerk"=-499.99999964711606, "heading"=-0.0}, {"dt"=0.005, "x"=119.98778725000024, "y"=260.0, "position"=-119.98781850000024, "velocity"=-0.763149999994539, "acceleration"=28.8699999993014, "jerk"=-500.0000003292371, "heading"=-0.0}, {"dt"=0.005, "x"=119.99094375000023, "y"=260.0, "position"=-119.99097500000023, "velocity"=-0.6312999999977364, "acceleration"=26.369999999360516, "jerk"=-499.99999998817657, "heading"=-0.0}, {"dt"=0.005, "x"=119.99350350000017, "y"=260.0, "position"=-119.99353475000018, "velocity"=-0.5119499999892696, "acceleration"=23.87000000169337, "jerk"=-499.9999995334292, "heading"=-0.0}, {"dt"=0.005, "x"=119.99552900000015, "y"=260.0, "position"=-119.99556025000015, "velocity"=-0.405099999994718, "acceleration"=21.369999998910316, "jerk"=-500.00000055661076, "heading"=-0.0}, {"dt"=0.005, "x"=119.99708275000015, "y"=260.0, "position"=-119.99711400000015, "velocity"=-0.31074999999987085, "acceleration"=18.869999998969433, "jerk"=-499.99999998817657, "heading"=-0.0}, {"dt"=0.005, "x"=119.99822725000011, "y"=260.0, "position"=-119.99825850000012, "velocity"=-0.22889999999335942, "acceleration"=16.370000001302287, "jerk"=-499.9999995334292, "heading"=-0.0}, {"dt"=0.005, "x"=119.99902500000012, "y"=260.0, "position"=-119.99905625000012, "velocity"=-0.15955000000076325, "acceleration"=13.869999998519233, "jerk"=-500.00000055661076, "heading"=-0.0}, {"dt"=0.005, "x"=119.99953850000009, "y"=260.0, "position"=-119.99956975000009, "velocity"=-0.10269999999366064, "acceleration"=11.370000001420522, "jerk"=-499.9999994197424, "heading"=-0.0}, {"dt"=0.005, "x"=119.99983025000007, "y"=260.0, "position"=-119.99986150000008, "velocity"=-0.05834999999763113, "acceleration"=8.869999999205902, "jerk"=-500.0000004429239, "heading"=-0.0}, {"dt"=0.005, "x"=119.99996275000007, "y"=260.0, "position"=-119.99999400000007, "velocity"=-0.026499999998463863, "acceleration"=6.369999999833453, "jerk"=-499.99999987448973, "heading"=-0.0}, {"dt"=0.005, "x"=119.99999850000006, "y"=260.0, "position"=-120.00002975000007, "velocity"=-0.007149999999001011, "acceleration"=3.8699999998925705, "jerk"=-499.99999998817657, "heading"=-0.0}, {"dt"=0.005, "x"=120.0, "y"=260.0, "position"=-120.00003125, "velocity"=-0.00029999998787388904, "acceleration"=1.3700000022254244, "jerk"=-499.9999995334292, "heading"=-0.0}, {"dt"=0.005, "x"=120.0, "y"=260.0, "position"=-120.00003125, "velocity"=-0.0, "acceleration"=0.05999999757477781, "jerk"=-262.0000009301293, "heading"=-0.0}])   [LabVIEW 2016]
uses:
  Pathfinder/VIs/Segment.ctl
  Pathfinder/VIs/Waypoint.ctl
  Pathfinder/Pathfinder.lvlib
panel:
  in  "path":T1[](array[typedef])=[{"x"=0.0, "y"=246.0, "angle"=0.0}, {"x"=120.0, "y"=246.0, "angle"=0.0}]
  out "Position":cluster{dbl[], dbl[]}[](graph)
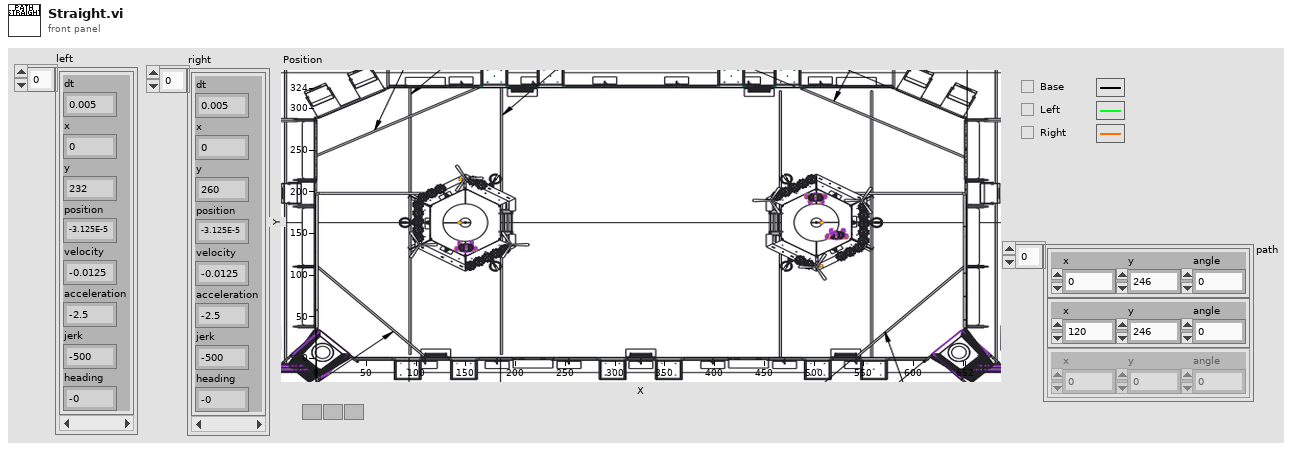
[diagram p1: front panel]
types:
  T1 = typedef "Pathfinder.lvlib/Waypoint.ctl" = cluster{"x":dbl, "y":dbl, "angle":dbl}
  T2 = typedef "Pathfinder.lvlib/Segment.ctl" = cluster{"dt":dbl, "x":dbl, "y":dbl, "position":dbl, "velocity":dbl, "acceleration":dbl, "jerk":dbl, "heading":dbl}
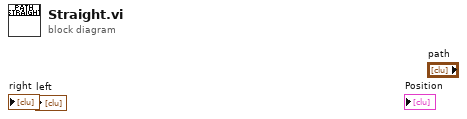
[diagram p0: block diagram]
diagram:
